vi "CRYGet Error Message.vi"(9 "String In":string, 10 "Error No":i32, 11 "Kind":string) -> (0 "Message Sub 3":string, 1 "Unicode Message Sub":string[](array[string]), 2 "Message Sub":string[](array[string]), 3 "Message":string, 4 "Unicode Message":string, 5 "Window Title":string)   [LabVIEW 2013]
uses:
  CRYMainGlobal.vi
panel:
  # "Get All Error Message."
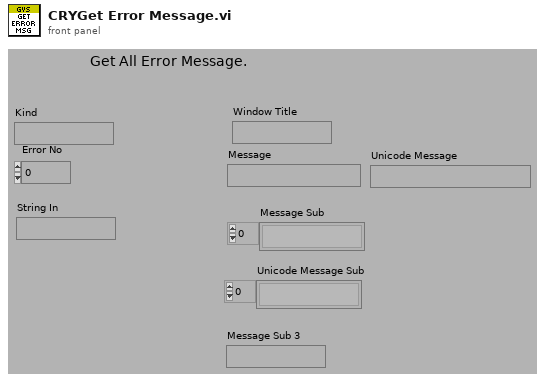
[diagram p1: front panel]
types:
  T1 = enum32{"English", "Chinese", "Korean", "Japanese", "Russian", "Chinese traditional"}
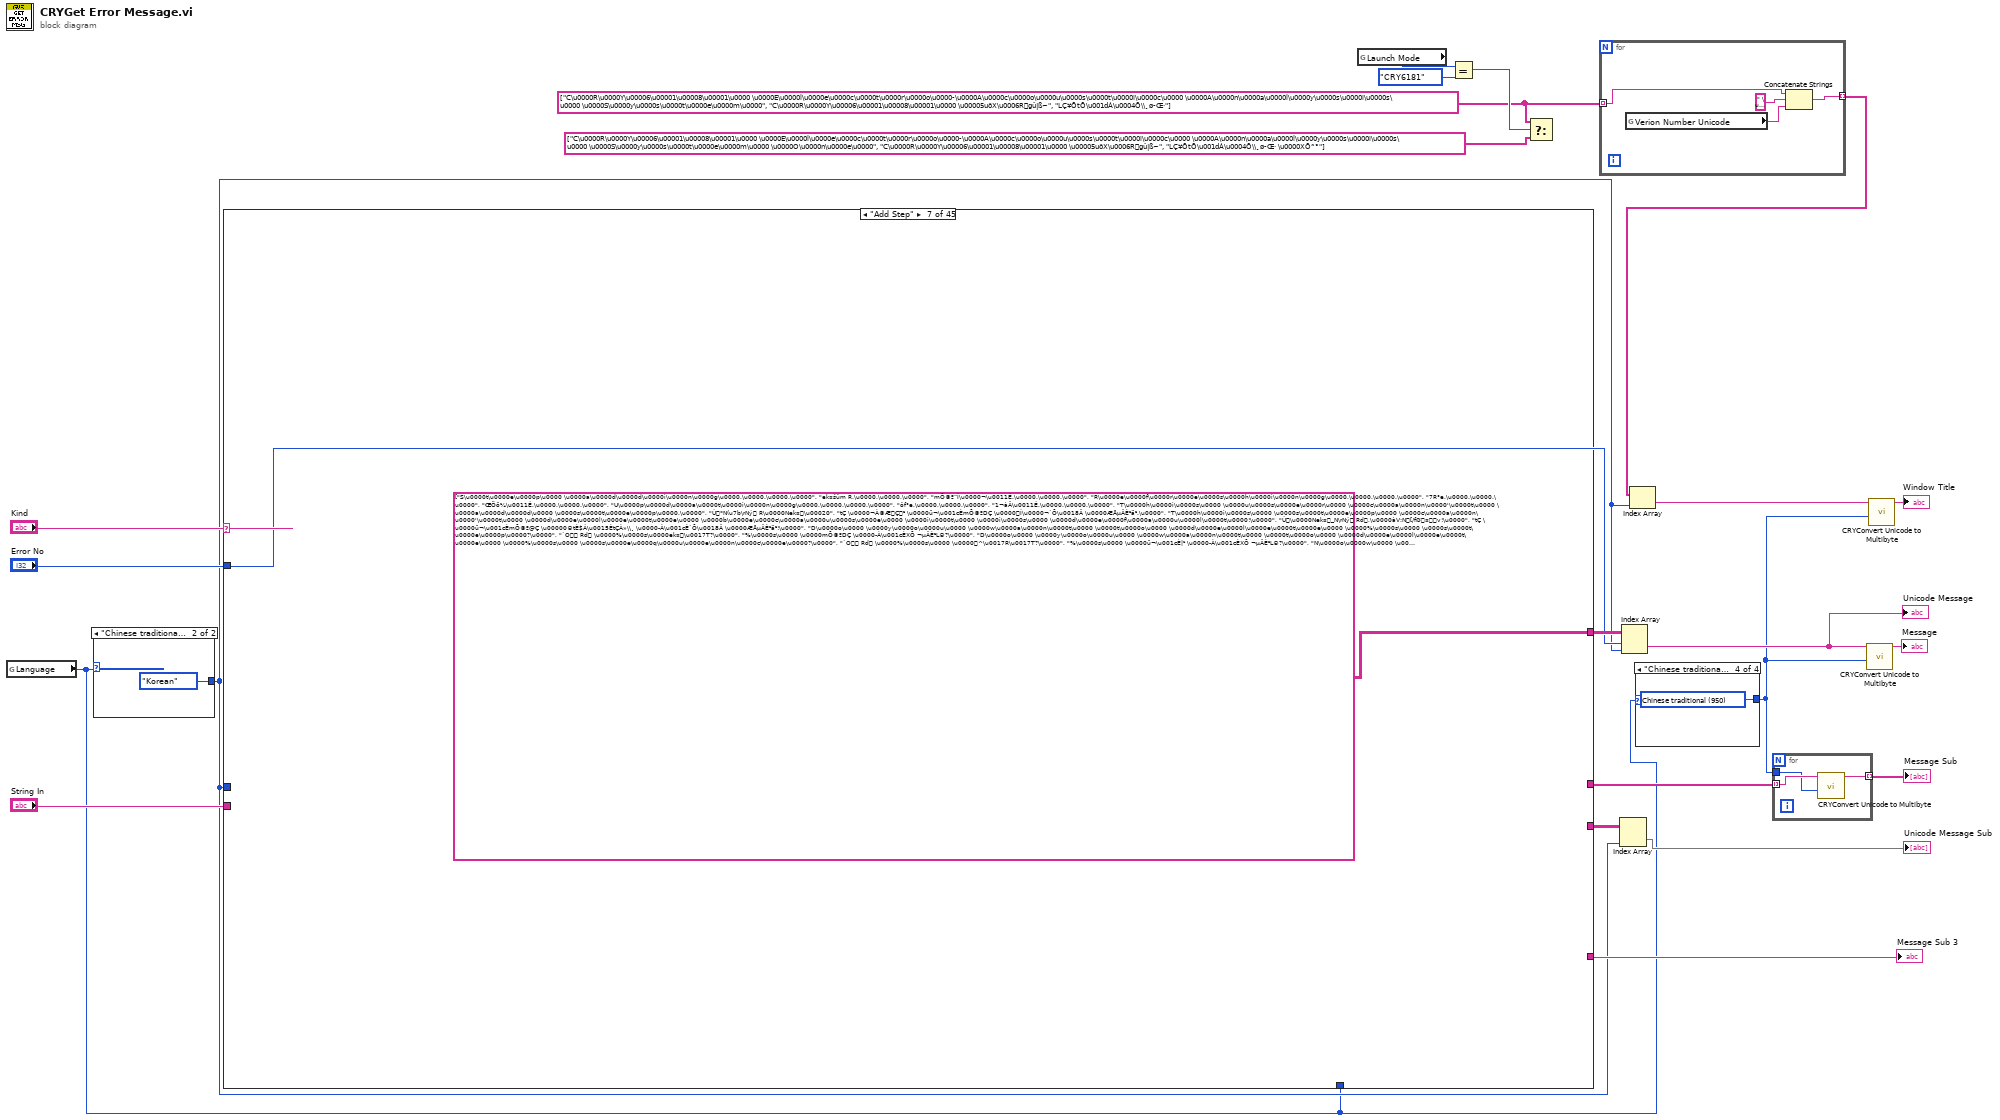
[diagram p0: block diagram]
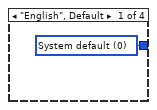
[diagram p3: hidden frame]
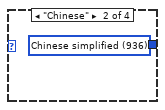
[diagram p4: hidden frame]
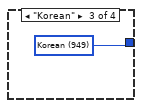
[diagram p5: hidden frame]
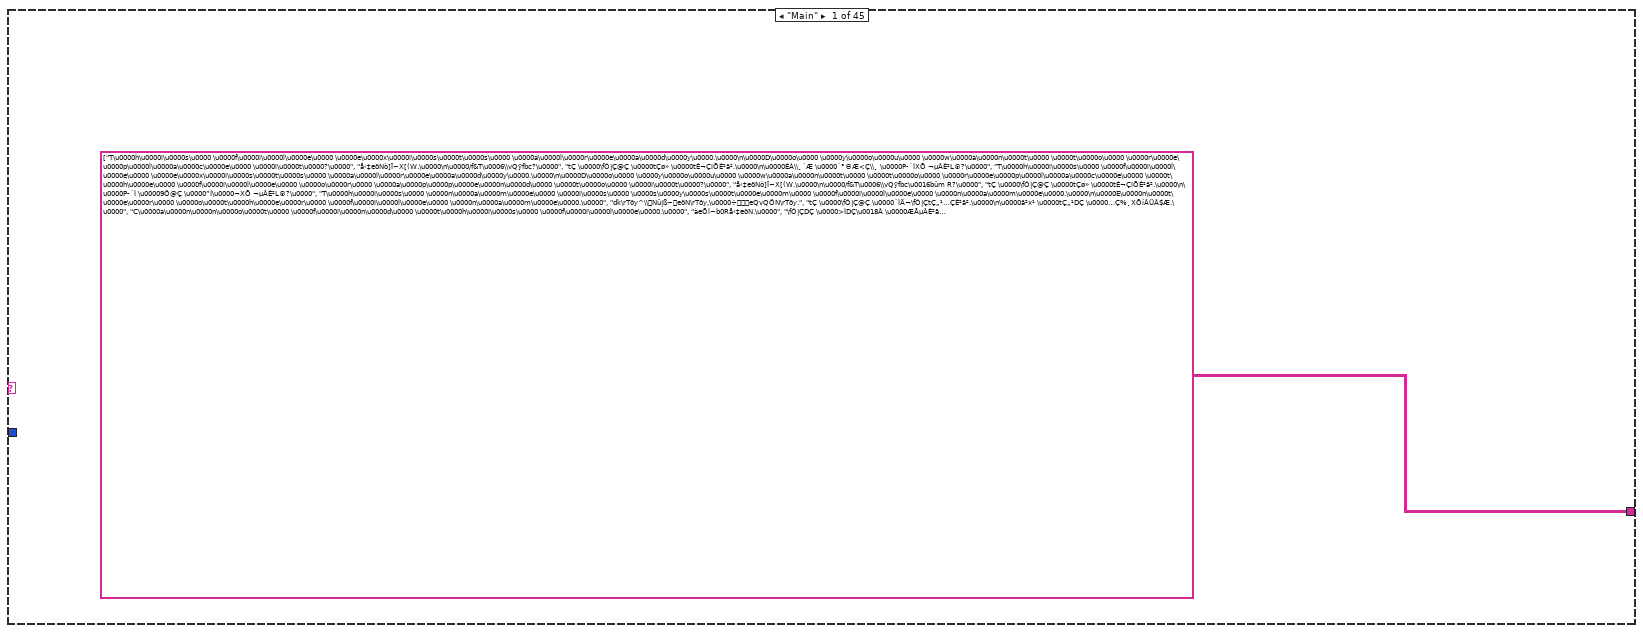
[diagram p6: hidden frame]
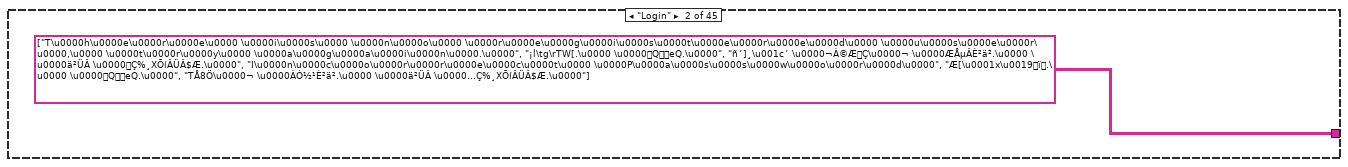
[diagram p7: hidden frame]
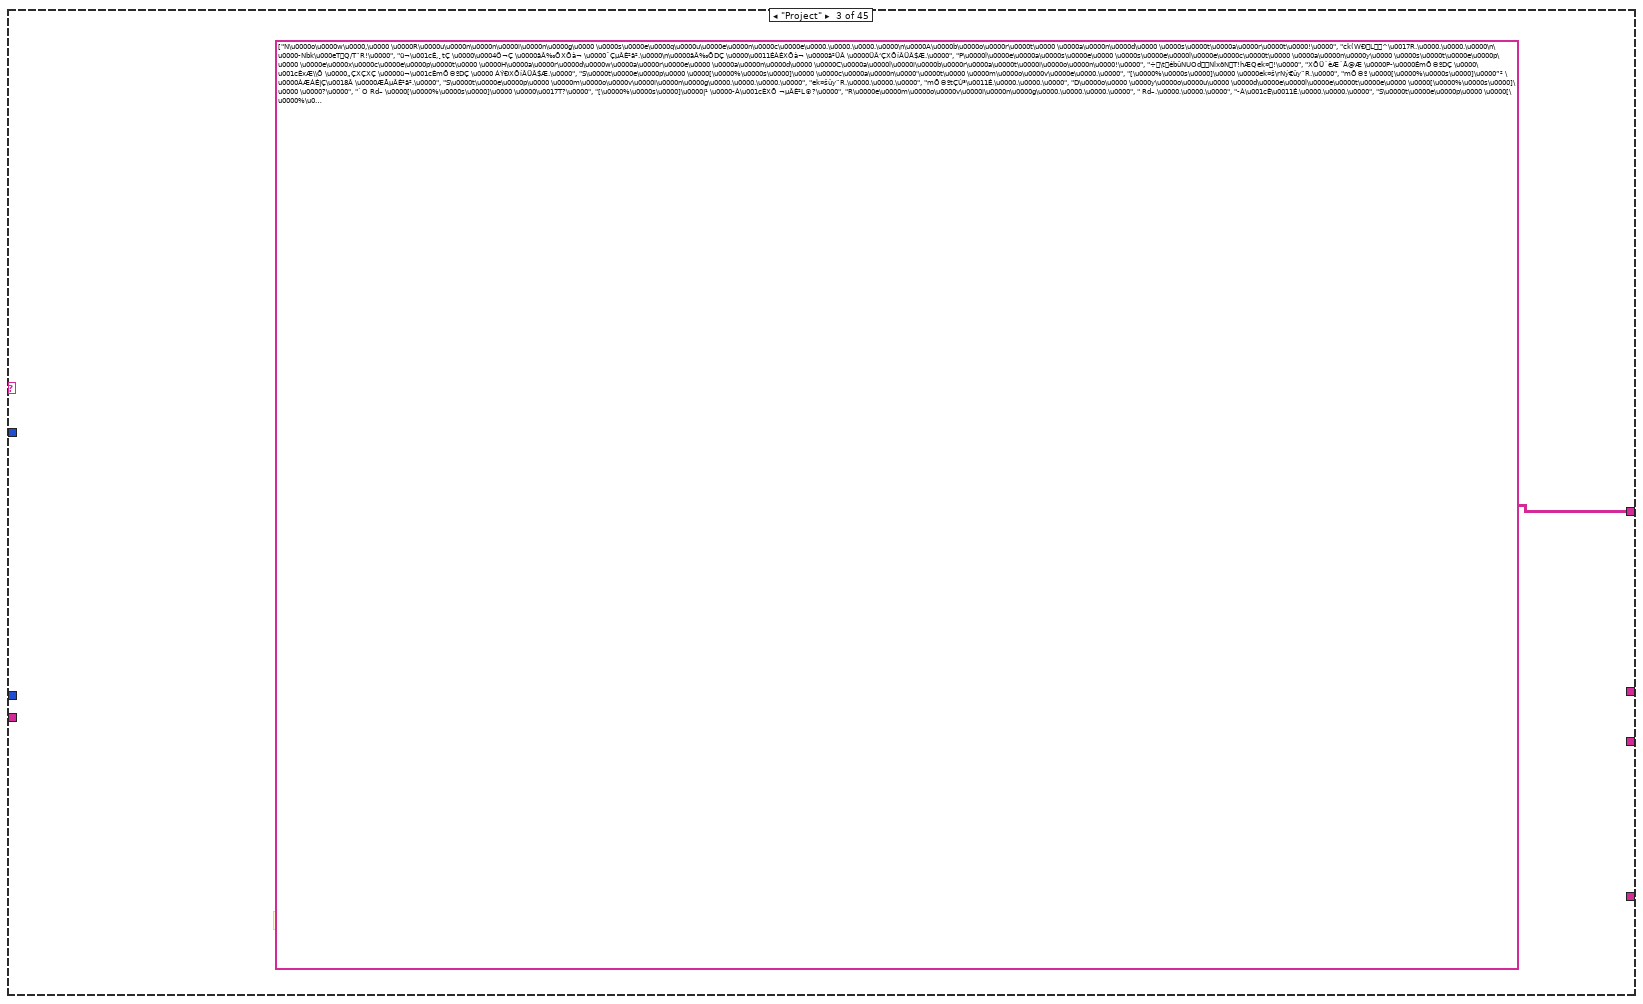
[diagram p8: hidden frame]
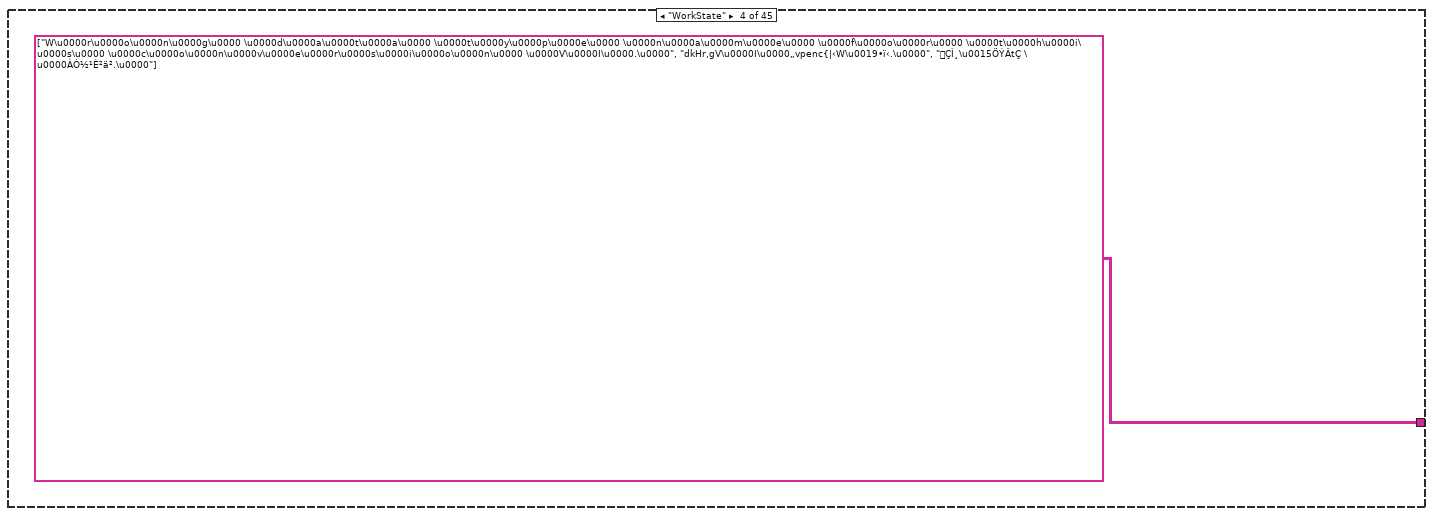
[diagram p9: hidden frame]
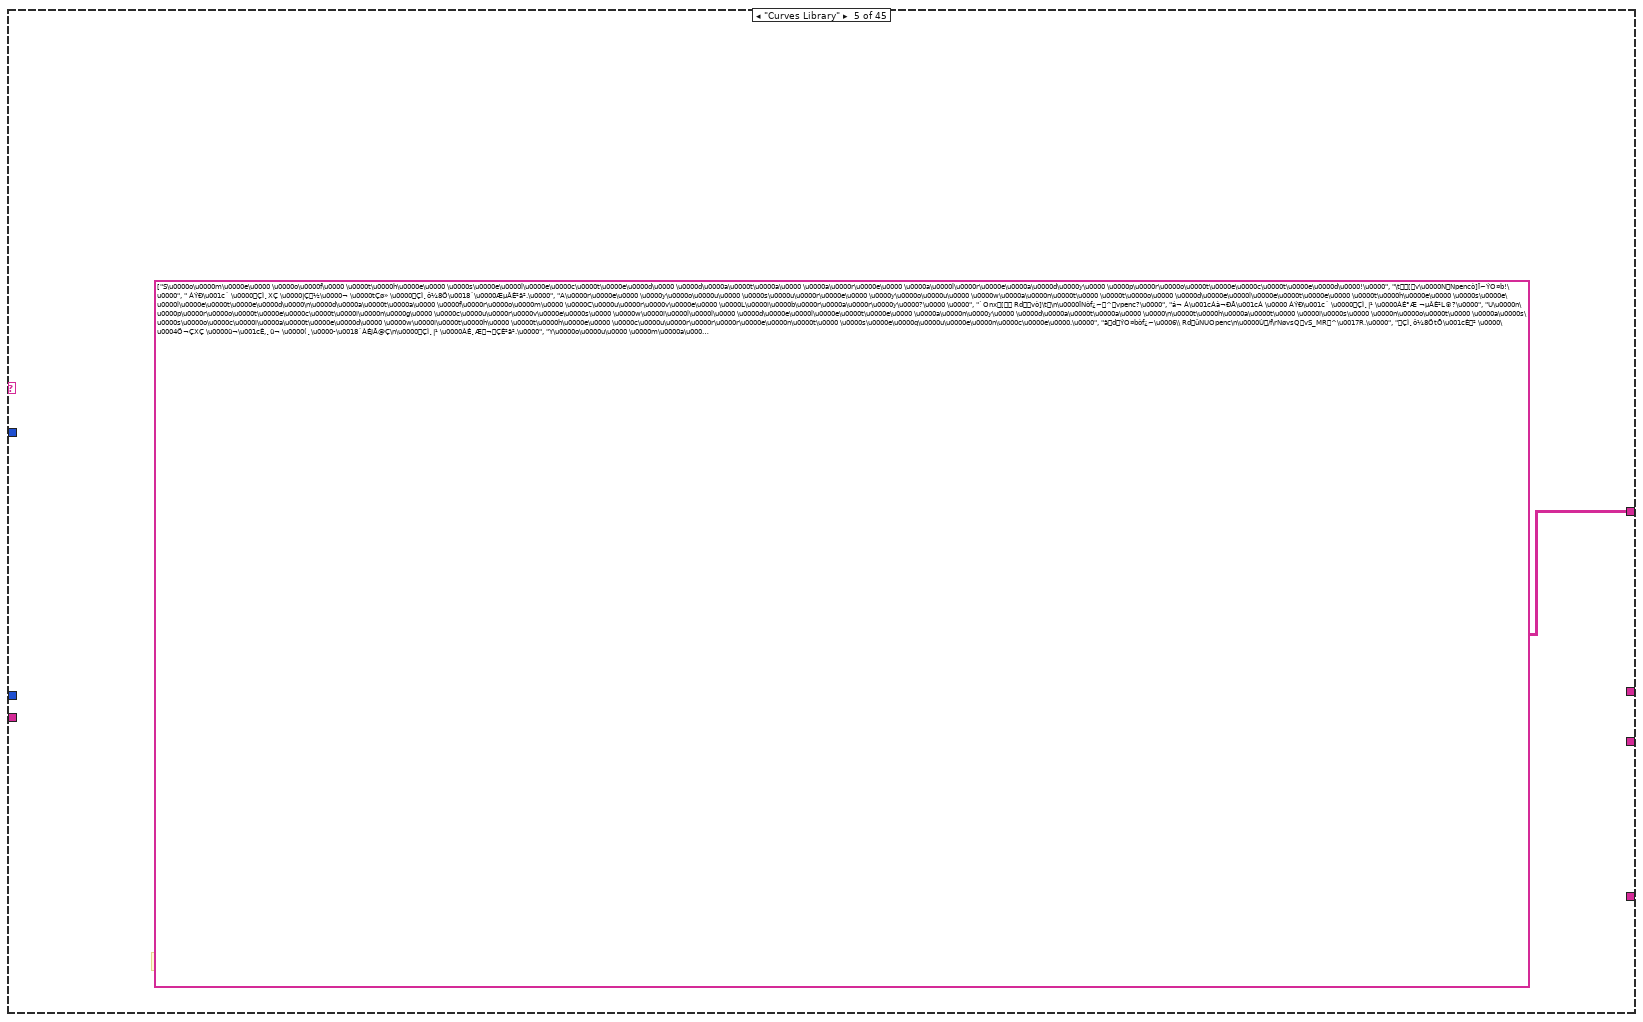
[diagram p10: hidden frame]
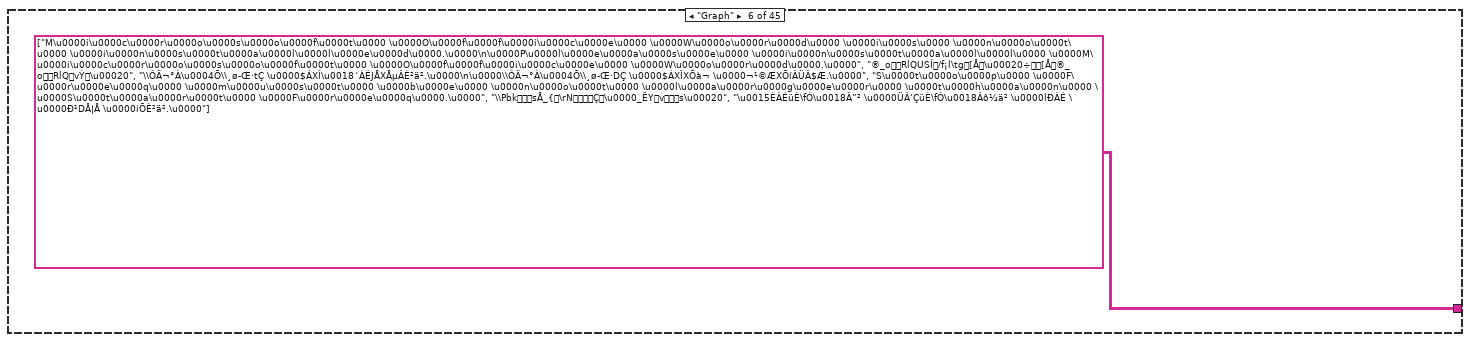
[diagram p11: hidden frame]
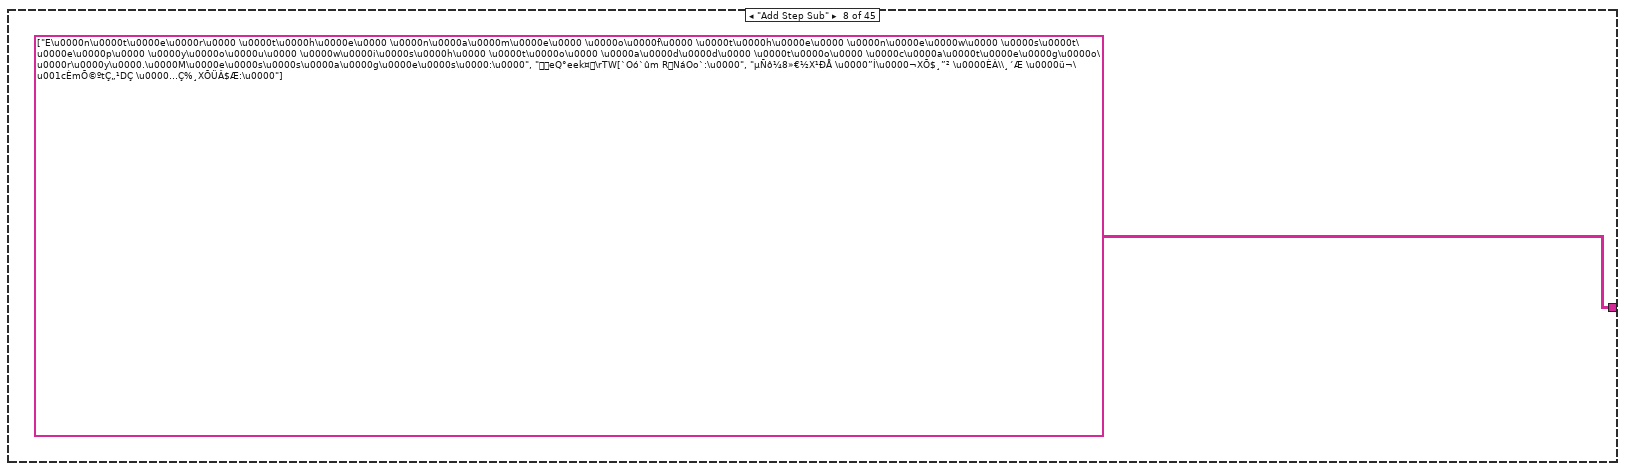
[diagram p12: hidden frame]
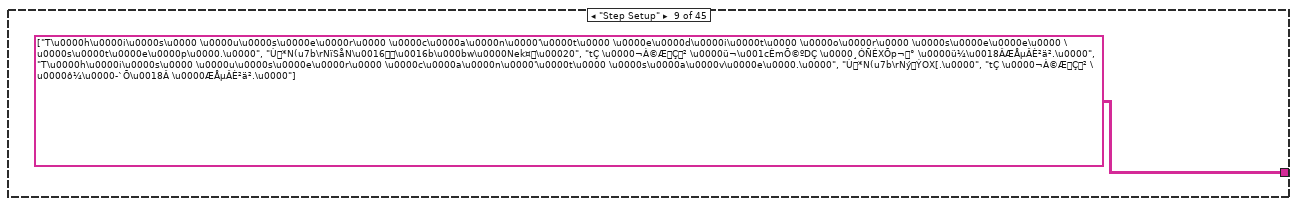
[diagram p13: hidden frame]
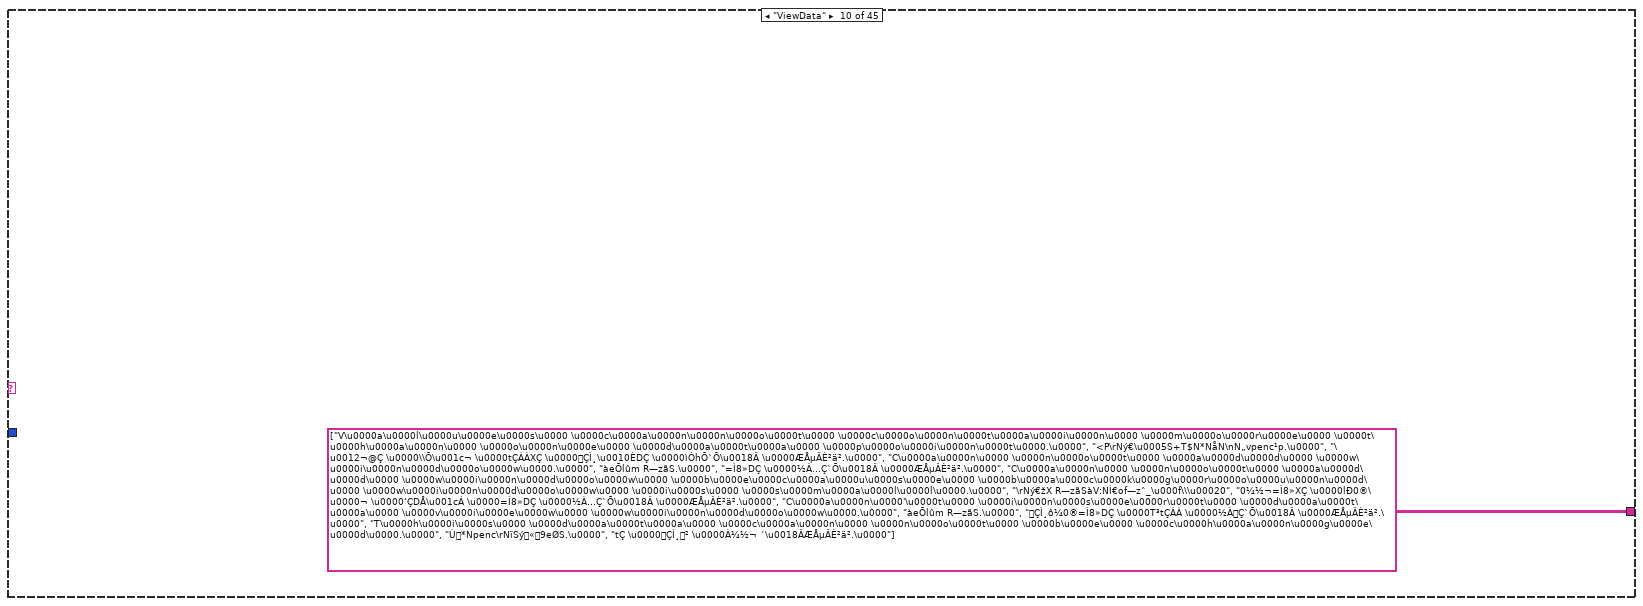
[diagram p14: hidden frame]
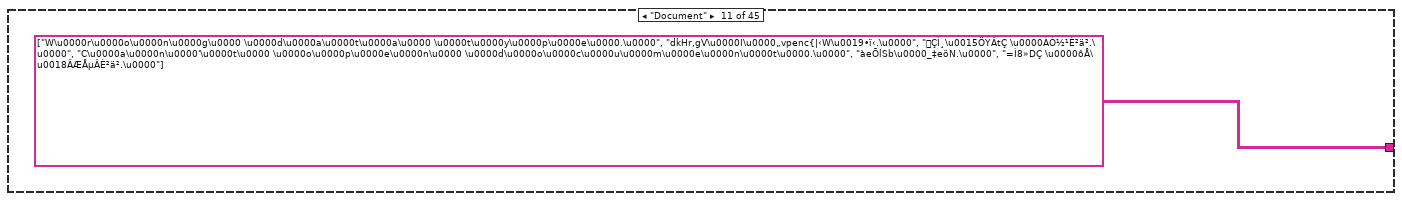
[diagram p15: hidden frame]
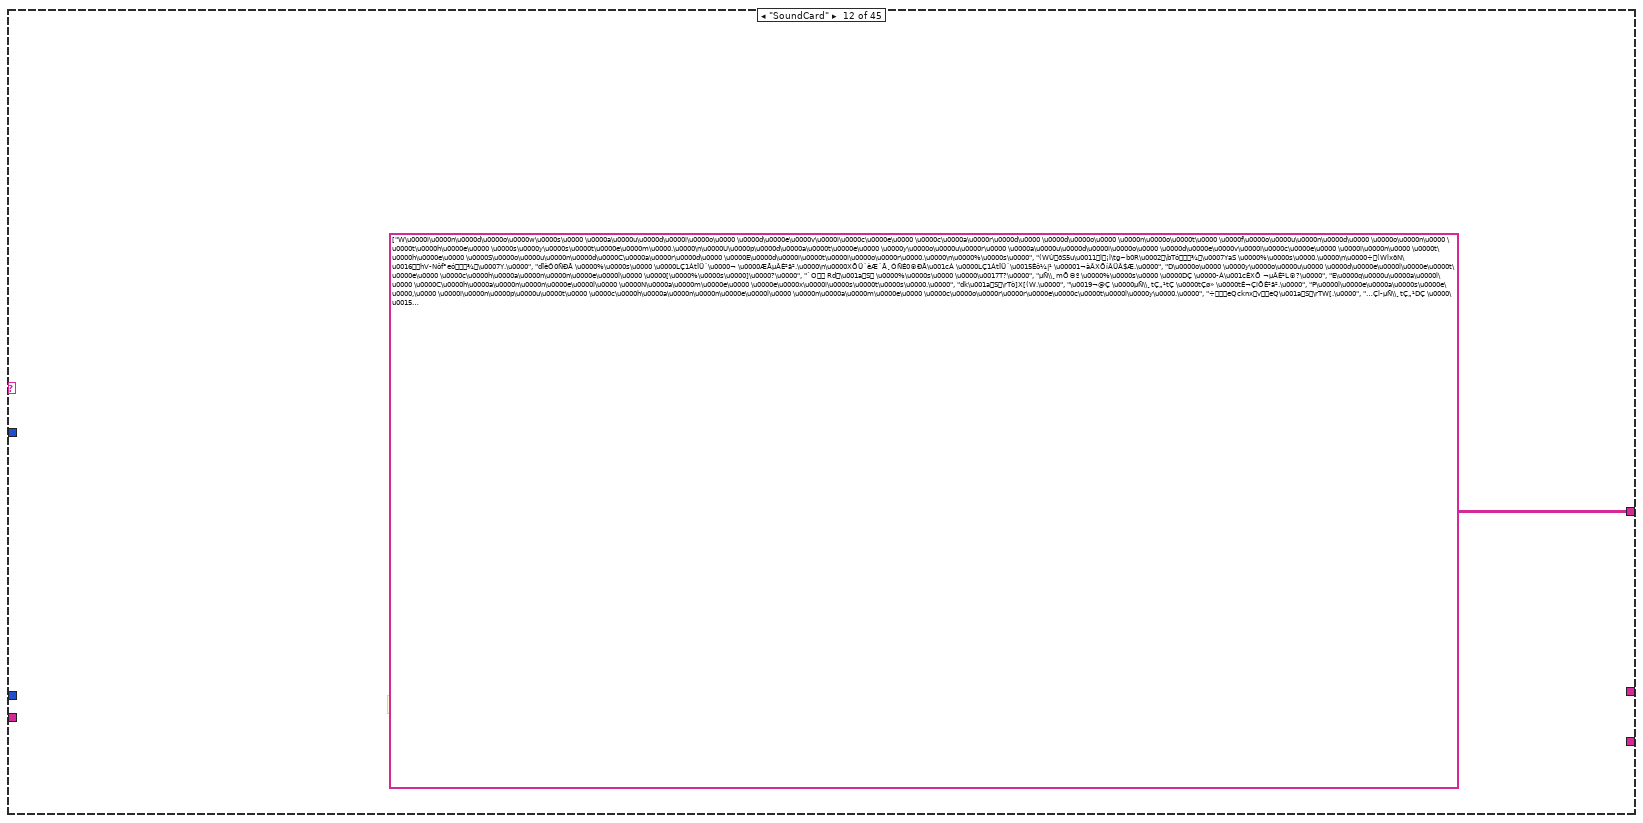
[diagram p16: hidden frame]
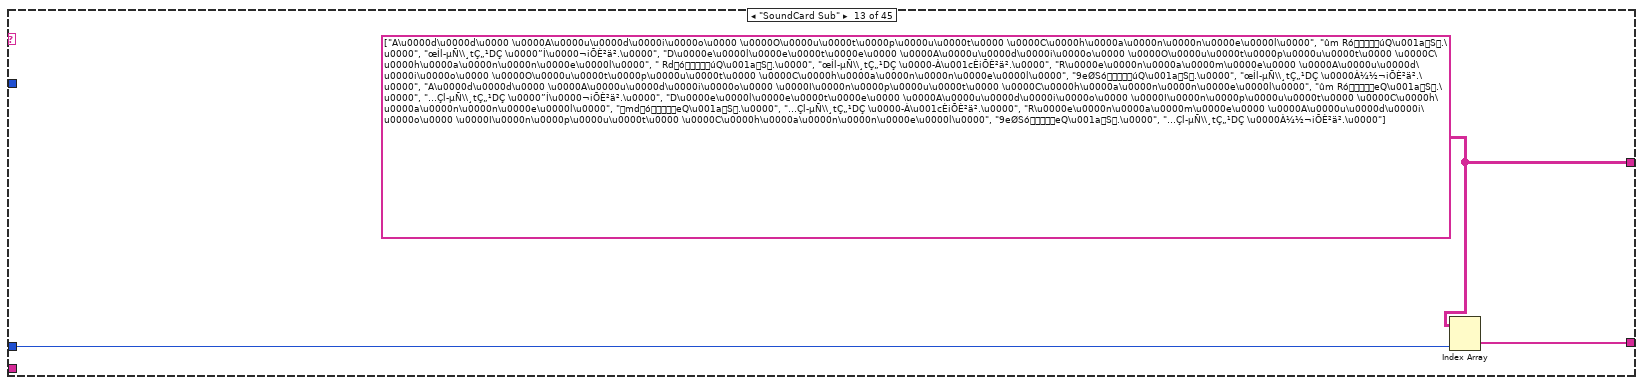
[diagram p17: hidden frame]
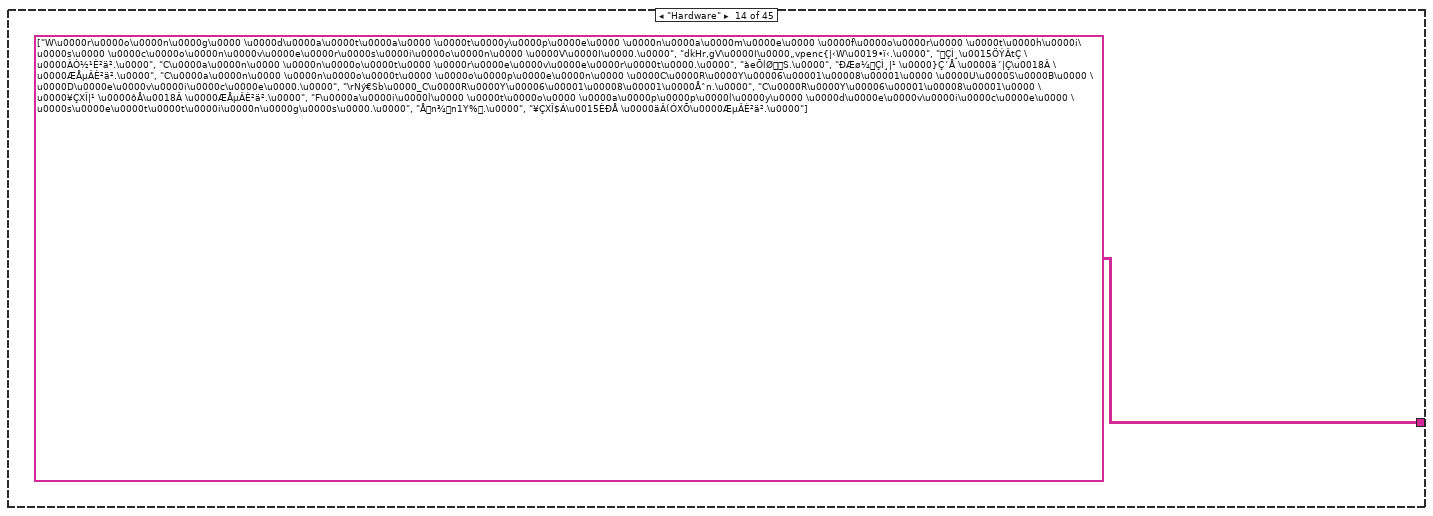
[diagram p18: hidden frame]
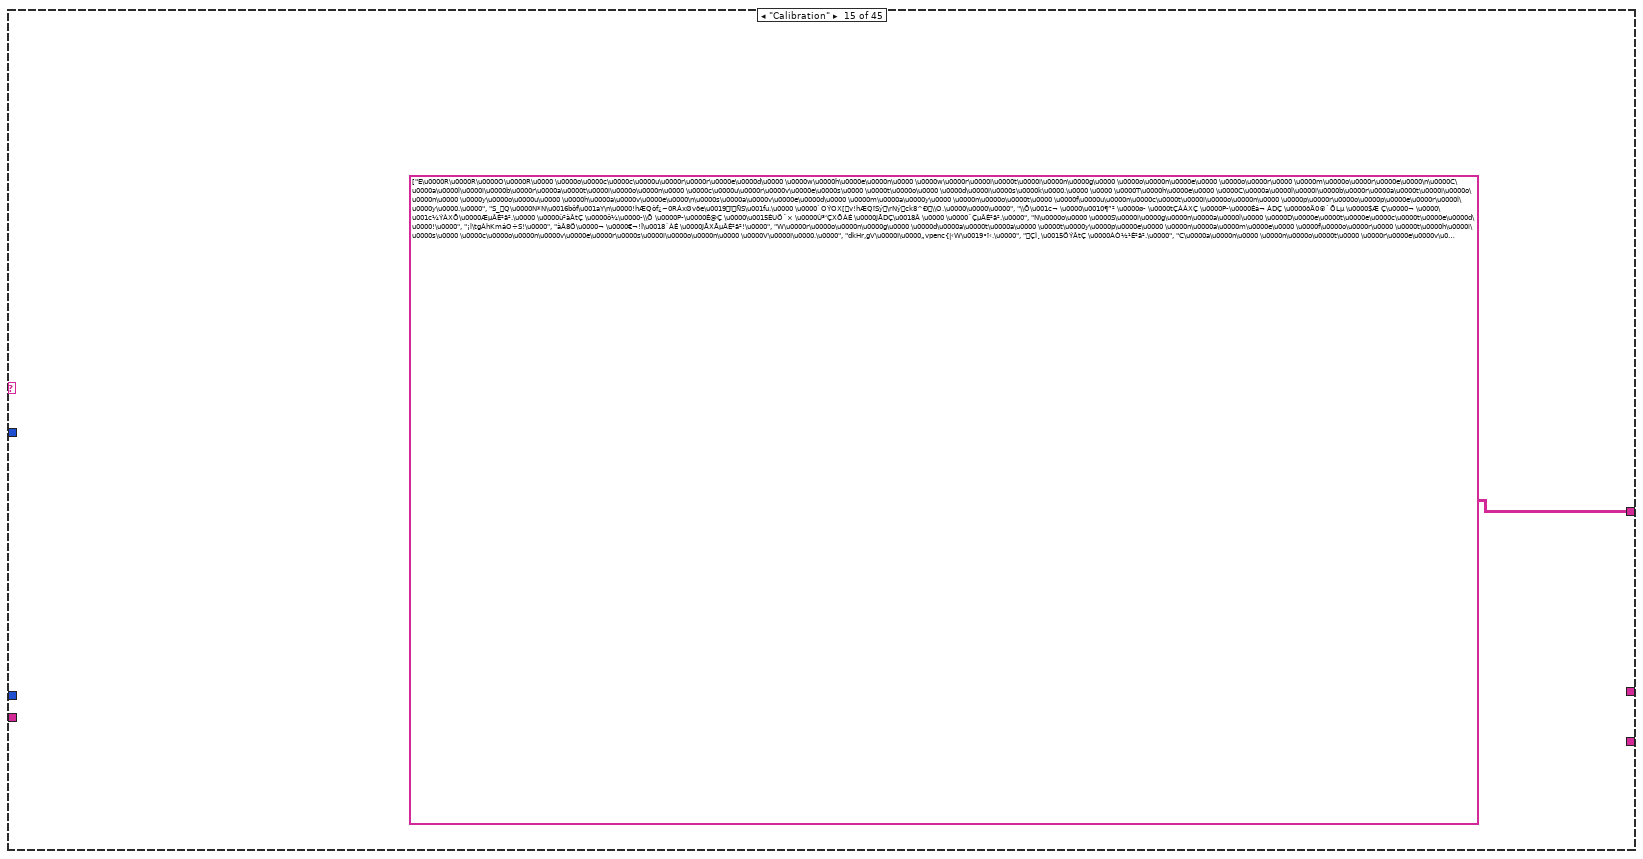
[diagram p19: hidden frame]
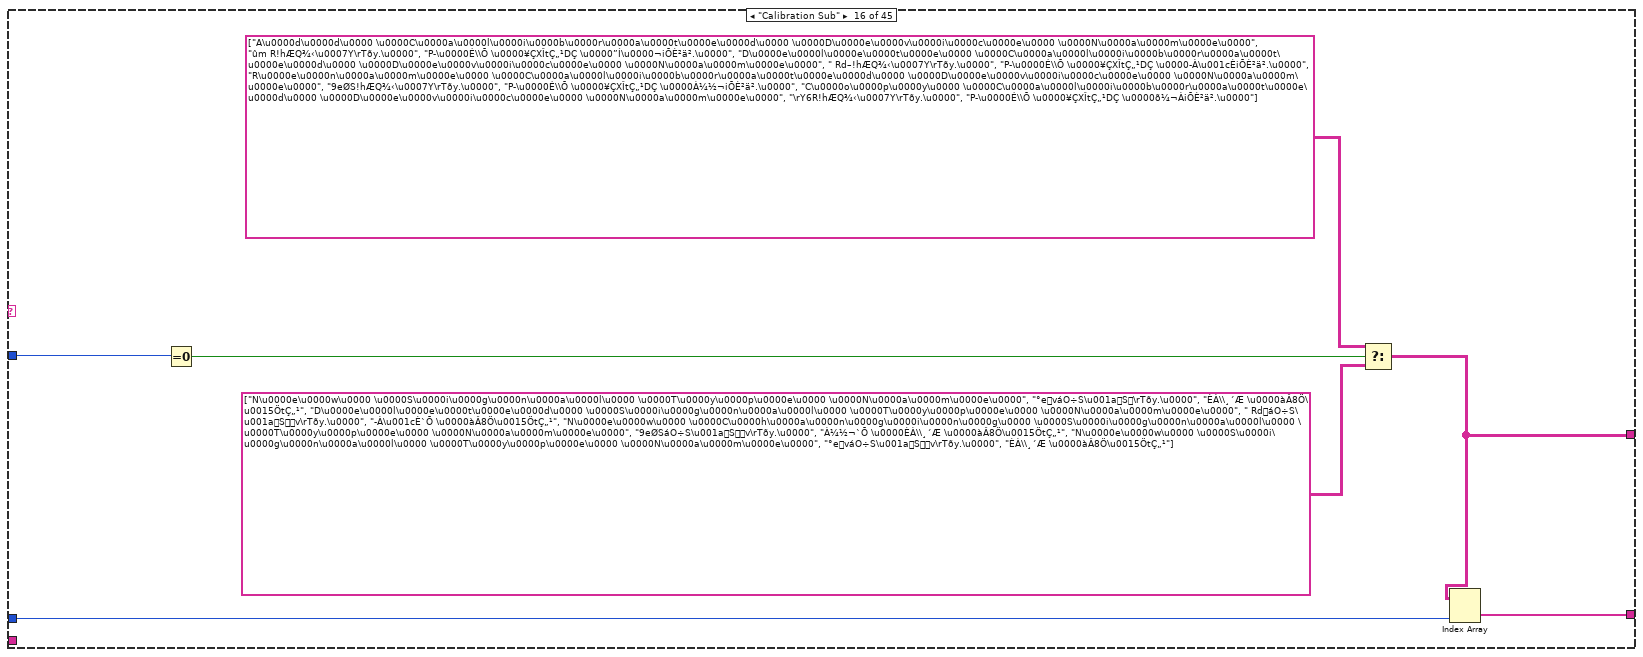
[diagram p20: hidden frame]
diagram:
  w2 = string[] ["C\u0000R\u0000Y\u00006\u00001\u00008\u00001\u0000 \u0000E\u0000l\u0000e\u0000c\u0000t\u0000r\u0000o\u0000-\u0000A\u0000c\u0000o\u0000u\u0000s\u0000t\u0000i\u0000c\u0000 \u0000A\u0000n\u0000a\u0000l\u0000y\u0000s\u0000i\u0000s\u0000 \u0000S\u0000y\u0000s\u0000t\u0000e\u0000m\u0000", "C\u0000R\u0000Y\u00006\u00001\u00008\u00001\u0000 \u00005uðX\u0006Rgû|ß~", "LÇ¥ÕtÕ\u001dÁ\u0004Õ\\¸ø­Œ·"]
  n1 = global read "CRYMainGlobal.vi" "Language"() -> (w7:T1)
  n2 = case shown="\"Chinese traditional\"" w7 {
    selector: w7 -> [w23 _]
    tunnel: [w23 T1."Korean" ("Language")] -> w8
    frame "English", Default {
    }
    frame "Chinese traditional" {
    }
  }
  n3 = case shown="\"Add Step\"" "Kind" {
    tunnel: [string[][] [["T\u0000h\u0000i\u0000s\u0000 \u0000f\u0000i\u0000l\u0000e\u0000 \u0000e\u0000x\u0000i\u0000s\u0000t\u0000s\u0000 \u0000a\u0000l\u0000r\u0000e\u0000a\u0000d\u0000y\u0000.\u0000\n\u0000D\u0000o\u0000 \u0000y\u0000o\u0000u\u0000 \u0000w\u0000a\u0000n\u0000t\u0000 \u0000t\u0000o\u0000 \u0000r\u0000e\u0000p\u0000l\u0000a\u0000c\u0000e\u0000 \u0000i\u0000t\u0000?\u0000", "å‹‡eöNò]Ï~X[(W.\u0000\n\u0000/f&T\u0006\\vQÿfbc?\u0000", "tÇ \u0000\fÓ|Ç@Ç \u0000tÇø» \u0000tÈ¬ÇiÕÈ²ä².\u0000\n\u0000ÈÀ\\¸´Æ \u0000´°©Æ<Ç\\¸ \u0000P­´ÌXÕ ¬µÂÈ²L®?\u0000"], ["T\u0000h\u0000i\u0000s\u0000 \u0000f\u0000i\u0000l\u0000e\u0000 \u0000e\u0000x\u0000i\u0000s\u0000t\u0000s\u0000 \u0000a\u0000l\u0000r\u0000e\u0000a\u0000d\u0000y\u0000.\u0000\n\u0000D\u0000o\u0000 \u0000y\u0000o\u0000u\u0000 \u0000w\u0000a\u0000n\u0000t\u0000 \u0000t\u0000o\u0000 \u0000r\u0000e\u0000p\u0000l\u0000a\u0000c\u0000e\u0000 \u0000t\u0000h\u0000e\u0000 \u0000f\u0000i\u0000l\u0000e\u0000 \u0000o\u0000r\u0000 \u0000a\u0000p\u0000p\u0000e\u0000n\u0000d\u0000 \u0000t\u0000o\u0000 \u0000i\u0000t\u0000?\u0000", "å‹‡eöNò]Ï~X[(W.\u0000\n\u0000/f&T\u0006\\vQÿfbc\u0016bûm R?\u0000", "tÇ \u0000\fÓ|Ç@Ç \u0000tÇø» \u0000tÈ¬ÇiÕÈ²ä².\u0000\n\u0000P­´Ì \u00009Ö@Ç \u0000”Í\u0000¬XÕ ¬µÂÈ²L®?\u0000"], ["T\u0000h\u0000i\u0000s\u0000 \u0000n\u0000a\u0000m\u0000e\u0000 \u0000i\u0000s\u0000 \u0000s\u0000y\u0000s\u0000t\u0000e\u0000m\u0000 \u0000f\u0000i\u0000l\u0000e\u0000 \u0000n\u0000a\u0000m\u0000e\u0000.\u0000\n\u0000E\u0000n\u0000t\u0000e\u0000r\u0000 \u0000o\u0000t\u0000h\u0000e\u0000r\u0000 \u0000f\u0000i\u0000l\u0000e\u0000 \u0000n\u0000a\u0000m\u0000e\u0000.\u0000", "dk\rTðy^\\Nû|ß~eöN\rTðy,\u0000÷eQvQÖN\rTðy.", "tÇ \u0000\fÓ|Ç@Ç \u0000´ÌÄ¬\fÓ|ÇtÇ„¹…ÇÈ²ä².\u0000\n\u0000ä²x¹ \u0000tÇ„¹DÇ \u0000…Ç%¸XÕíÂÜÂ$Æ.\u0000"], ["C\u0000a\u0000n\u0000n\u0000o\u0000t\u0000 \u0000f\u0000i\u0000n\u0000d\u0000 \u0000t\u0000h\u0000i\u0000s\u0000 \u0000f\u0000i\u0000l\u0000e\u0000.\u0000", "àeÕl~b0Rå‹‡eöN.\u0000", "\fÓ|ÇDÇ \u0000>ÌDÇ\u0018Â \u0000ÆÅµÂÈ²ä².\u0000"], ["F\u0000i\u0000l\u0000e\u0000 \u0000e\u0000x\u0000t\u0000e\u0000n\u0000s\u0000i\u0000o\u0000n\u0000 \u0000i\u0000s\u0000 \u0000n\u0000o\u0000t\u0000 \u0000e\u0000q\u0000u\u0000a\u0000l\u0000.\u0000 \u0000(\u0000%\u0000s\u0000)\u0000", "‡eöNibU\\\rT\rN\fT.\u0000(\u0000%\u0000s\u0000)\u0000", "\fÓ|ÇUÖ¥ÇÇ\u0000¬ \u0000\u0019¬ÀÉ \u0000JÅµÂÈ²ä².\u0000(\u0000%\u0000s\u0000)\u0000"], ["W\u0000r\u0000o\u0000n\u0000g\u0000 \u0000d\u0000a\u0000t\u0000a\u0000 \u0000t\u0000y\u0000p\u0000e\u0000 \u0000n\u0000a\u0000m\u0000e\u0000 \u0000f\u0000o\u0000r\u0000 \u0000t\u0000h\u0000i\u0000s\u0000 \u0000v\u0000e\u0000r\u0000s\u0000i\u0000o\u0000n\u0000 \u0000V\u0000I\u0000", "dkHr,gV\u0000I\u0000„vpenc{|‹W\u0019•ï‹.\u0000", "ÇÌ¸À¼XÖÜÂ \u0000ÇÌ¸\u0015ÖtÇ \u0000ÀÒ½¹È²ä².\u0000"], ["D\u0000o\u0000 \u0000y\u0000o\u0000u\u0000 \u0000w\u0000a\u0000n\u0000t\u0000 \u0000t\u0000o\u0000 \u0000s\u0000a\u0000v\u0000e\u0000 \u0000c\u0000h\u0000a\u0000n\u0000g\u0000e\u0000s\u0000 \u0000?\u0000", "/f&TÝOX[ò]ôf9e„v…Q¹[?\u0000", "ô¼\u0000­XÕ ¬µÂÈ²L®?\u0000"], ["E\u0000r\u0000r\u0000o\u0000r\u0000 \u0000o\u0000c\u0000c\u0000u\u0000r\u0000e\u0000d\u0000 \u0000i\u0000n\u0000 \u0000e\u0000x\u0000e\u0000c\u0000u\u0000t\u0000i\u0000n\u0000g\u0000 \u0000t\u0000h\u0000e\u0000 \u0000A\u0000d\u0000o\u0000b\u0000e\u0000 \u0000R\u0000e\u0000a\u0000d\u0000e\u0000r\u0000.\u0000e\u0000x\u0000e\u0000!\u0000\n\u0000P\u0000l\u0000e\u0000a\u0000s\u0000e\u0000 \u0000s\u0000e\u0000t\u0000u\u0000p\u0000 \u0000t\u0000h\u0000e\u0000 \u0000A\u0000d\u0000o\u0000b\u0000e\u0000 \u0000R\u0000e\u0000a\u0000d\u0000e\u0000r\u0000 \u0000P\u0000r\u0000o\u0000g\u0000r\u0000a\u0000m\u0000.\u0000", "÷‹‰[ÅˆA\u0000d\u0000o\u0000b\u0000e\u0000 \u0000R\u0000e\u0000a\u0000d\u0000e\u0000r\u0000.\u0000", "¬À©Æ$Á…º\u001cÁ|¹ \u0000ô¼0® \u0000\u0004ÇXÕìÅ \u0000P\u0000D\u0000F\u0000ôÅŒ·0® \u0000A\u0000c\u0000r\u0000o\u0000b\u0000a\u0000t\u0000|¹ \u0000$ÁXÎXÕíÂÜÂ$Æ.\u0000"], ["E\u0000r\u0000r\u0000o\u0000r\u0000 \u0000O\u0000c\u0000c\u0000u\u0000r\u0000e\u0000d\u0000 \u0000I\u0000n\u0000 \u0000d\u0000i\u0000s\u0000p\u0000l\u0000a\u0000y\u0000i\u0000n\u0000g\u0000 \u0000t\u0000h\u0000e\u0000 \u0000U\u0000s\u0000e\u0000r\u0000 \u0000M\u0000a\u0000n\u0000u\u0000a\u0000l\u0000!\u0000\n\u0000C\u0000R\u0000Y\u0000M\u0000a\u0000n\u0000u\u0000a\u0000l\u0000 \u0000f\u0000i\u0000l\u0000e\u0000 \u0000h\u0000a\u0000s\u0000 \u0000b\u0000e\u0000e\u0000n\u0000 \u0000m\u0000o\u0000v\u0000e\u0000d\u0000 \u0000o\u0000r\u0000 \u0000d\u0000e\u0000l\u0000e\u0000t\u0000e\u0000d\u0000.\u0000", "KbŒQ‡eöNò]«ˆûy¨R\u0016b Rd–.\u0000", "¬À©Æ$Á…º\u001cÁ\u0000¬ \u0000ÆÅµÂÈ²ä².\u0000 \u0000UÖxÇXÕíÂÜÂ$Æ.\u0000"], ["Y\u0000o\u0000u\u0000 \u0000a\u0000r\u0000e\u0000 \u0000s\u0000w\u0000i\u0000t\u0000c\u0000h\u0000i\u0000n\u0000g\u0000 \u0000b\u0000e\u0000t\u0000w\u0000e\u0000e\u0000n\u0000 \u0000C\u0000R\u0000Y\u00006\u00001\u00008\u00001\u0000 \u0000O\u0000n\u0000e\u0000 \u0000a\u0000n\u0000d\u0000 \u0000r\u0000e\u0000g\u0000u\u0000l\u0000a\u0000r\u0000 \u0000C\u0000R\u0000Y\u00006\u00001\u00008\u00001\u0000,\u0000 \u0000\n\u0000C\u0000R\u0000Y\u00006\u00001\u00008\u00001\u0000 \u0000m\u0000u\u0000s\u0000t\u0000 \u0000b\u0000e\u0000 \u0000r\u0000e\u0000s\u0000t\u0000a\u0000r\u0000t\u0000e\u0000d\u0000 \u0000a\u0000n\u0000d\u0000 \u0000i\u0000s\u0000 \u0000e\u0000x\u0000i\u0000t\u0000i\u0000n\u0000g\u0000 \u0000n\u0000o\u0000w\u0000.\u0000", "ck(WC\u0000R\u0000Y\u00006\u00001\u00008\u00001\u0000 \u0000O\u0000n\u0000e\u0000T\u0007hÆQC\u0000R\u0000Y\u00006\u00001\u00008\u00001\u0000KNô\u0007Rbc.\u0000\n\u0000C\u0000R\u0000Y\u00006\u00001\u00008\u00001\u0000Å_{Í°e/T¨R,\u0000ck(W\u0000úQ\u00020", "ù²àÂ@Ç \u0000ÀÉ\b® \u0000LÇ¥ÕtÕ\u001dÁ\u0004Õ\\¸ø­Œ·ü¬ \u0000LÇ¥ÕtÕ\u001dÁ\u0004Õ\\¸ø­Œ· \u0000XÕ˜°¬ÀtÇÐÅ \u0000\bÈXÖXÕ$¸à¬ \u0000XÕà¬ˆÇµÂÈ²ä².\u0000 \u0000 \u0000\n\u0000LÇ¥ÕtÕ\u001dÁ\u0004Õ\\¸ø­Œ·DÇ \u0000¬Ç0®Ù³XÕ|Å|Å \u0000XÕpº \u0000ç¬ \u0000\u0004Õ\\¸ø­Œ·@Ç \u0000DÆÌ¸)´È²ä².\u0000"], ["L\u0000a\u0000n\u0000g\u0000u\u0000a\u0000g\u0000e\u0000 \u0000s\u0000e\u0000t\u0000t\u0000i\u0000n\u0000g\u0000 \u0000i\u0000s\u0000 \u0000c\u0000h\u0000a\u0000n\u0000g\u0000e\u0000d\u0000.\u0000\n\u0000C\u0000R\u0000Y\u00006\u00001\u00008\u00001\u0000 \u0000m\u0000u\u0000s\u0000t\u0000 \u0000b\u0000e\u0000 \u0000r\u0000e\u0000s\u0000t\u0000a\u0000r\u0000t\u0000e\u0000d\u0000 \u0000a\u0000n\u0000d\u0000 \u0000i\u0000s\u0000 \u0000e\u0000x\u0000i\u0000t\u0000i\u0000n\u0000g\u0000 \u0000n\u0000o\u0000w\u0000.\u0000", "í\u0000¾n«9eØS\u00020\n\u0000C\u0000R\u0000Y\u00006\u00001\u00008\u00001\u0000Å_{Í°e/T¨Rck(W\u0000úQ\u00020", "¸Å´Å$Á\u0015ÈtÇ \u0000À¼½¬\u0018´\u0000ÆµÂÈ²ä².\u0000\n\u0000C\u0000R\u0000Y\u00006\u00001\u00008\u00001\u0000”² \u0000¬Ç0®Ù³XÕìÅ|Å \u0000iÕÈ²ä².\u0000"], ["N\u0000o\u0000 \u0000H\u0000a\u0000r\u0000d\u0000w\u0000a\u0000r\u0000e\u0000 \u0000K\u0000e\u0000y\u0000!\u0000", "¡l\tglxöNÆ[¥”!\u0000", "XÕÜ´èÆ´Å¤Ð\u0000¬ \u0000ÆÅµÂÈ²ä²!\u0000"]] ("Array") string[][] [["T\u0000h\u0000e\u0000r\u0000e\u0000 \u0000i\u0000s\u0000 \u0000n\u0000o\u0000 \u0000r\u0000e\u0000g\u0000i\u0000s\u0000t\u0000e\u0000r\u0000e\u0000d\u0000 \u0000u\u0000s\u0000e\u0000r\u0000,\u0000 \u0000t\u0000r\u0000y\u0000 \u0000a\u0000g\u0000a\u0000i\u0000n\u0000.\u0000", "¡l\tg\rTW[.\u0000 \u0000QeQ.\u0000", "ñ´]¸\u001c´ \u0000¬À©ÆÇ\u0000¬ \u0000ÆÅµÂÈ²ä².\u0000 \u0000ä²ÜÂ \u0000Ç%¸XÕíÂÜÂ$Æ.\u0000"], ["I\u0000n\u0000c\u0000o\u0000r\u0000r\u0000e\u0000c\u0000t\u0000 \u0000P\u0000a\u0000s\u0000s\u0000w\u0000o\u0000r\u0000d\u0000", "Æ[\u0001x\u0019ï.\u0000 \u0000QeQ.\u0000", "TÅ8Ö\u0000¬ \u0000ÀÒ½¹È²ä².\u0000 \u0000ä²ÜÂ \u0000…Ç%¸XÕíÂÜÂ$Æ.\u0000"]] string[][] [["N\u0000o\u0000w\u0000,\u0000 \u0000R\u0000u\u0000n\u0000n\u0000i\u0000n\u0000g\u0000 \u0000s\u0000e\u0000q\u0000u\u0000e\u0000n\u0000c\u0000e\u0000.\u0000.\u0000.\u0000\n\u0000A\u0000b\u0000o\u0000r\u0000t\u0000 \u0000a\u0000n\u0000d\u0000 \u0000s\u0000t\u0000a\u0000r\u0000t\u0000!\u0000", "ck(WÐL^\u0017R.\u0000.\u0000.\u0000\n\u0000-Nbk\u000eTQ/T¨R!\u0000", "ü¬\u001cÈ,¸tÇ \u0000\u0004Ö¬Ç \u0000äÂ‰ÕXÕà¬ \u0000ˆÇµÂÈ²ä².\u0000\n\u0000äÂ‰ÕDÇ \u0000\u0011ÉÀÉXÕà¬ \u0000ä²ÜÂ \u0000ÜÂ‘ÇXÕíÂÜÂ$Æ.\u0000"], ["P\u0000l\u0000e\u0000a\u0000s\u0000e\u0000 \u0000s\u0000e\u0000l\u0000e\u0000c\u0000t\u0000 \u0000a\u0000n\u0000y\u0000 \u0000s\u0000t\u0000e\u0000p\u0000 \u0000e\u0000x\u0000c\u0000e\u0000p\u0000t\u0000 \u0000H\u0000a\u0000r\u0000d\u0000w\u0000a\u0000r\u0000e\u0000 \u0000a\u0000n\u0000d\u0000 \u0000C\u0000a\u0000l\u0000i\u0000b\u0000r\u0000a\u0000t\u0000i\u0000o\u0000n\u0000!\u0000", "÷\tébûNUOdNlxöNT!hÆQek¤!\u0000", "XÕÜ´èÆ´Å@Æ \u0000P­\u0000ÉmÕ©ºDÇ \u0000\u001cÈxÆ\\Õ \u0000„ÇXÇXÇ \u0000ü¬\u001cÈmÕ©ºDÇ \u0000 ÁÝÐXÕíÂÜÂ$Æ.\u0000"], ["S\u0000t\u0000e\u0000p\u0000 \u0000[\u0000%\u0000s\u0000]\u0000 \u0000c\u0000a\u0000n\u0000'\u0000t\u0000 \u0000m\u0000o\u0000v\u0000e\u0000.\u0000", "[\u0000%\u0000s\u0000]\u0000 \u0000ek¤š\rNý€ûy¨R.\u0000", "mÕ©º \u0000[\u0000%\u0000s\u0000]\u0000”² \u0000ÀÆÁÉ|Ç\u0018Â \u0000ÆÅµÂÈ²ä².\u0000"], ["S\u0000t\u0000e\u0000p\u0000 \u0000m\u0000o\u0000v\u0000i\u0000n\u0000g\u0000.\u0000.\u0000.\u0000", "ek¤šûy¨R.\u0000.\u0000.\u0000", "mÕ©ºtÇÙ³\u0011É.\u0000.\u0000.\u0000"], ["D\u0000o\u0000 \u0000y\u0000o\u0000u\u0000 \u0000d\u0000e\u0000l\u0000e\u0000t\u0000e\u0000 \u0000[\u0000%\u0000s\u0000]\u0000 \u0000?\u0000", "`O Rd– \u0000[\u0000%\u0000s\u0000]\u0000 \u0000\u0017T?\u0000", "[\u0000%\u0000s\u0000]\u0000|¹ \u0000­À\u001cÈXÕ ¬µÂÈ²L®?\u0000"], ["R\u0000e\u0000m\u0000o\u0000v\u0000i\u0000n\u0000g\u0000.\u0000.\u0000.\u0000", " Rd–.\u0000.\u0000.\u0000", "­À\u001cÈ\u0011É.\u0000.\u0000.\u0000"], ["S\u0000t\u0000e\u0000p\u0000 \u0000[\u0000%\u0000s\u0000]\u0000 \u0000c\u0000a\u0000n\u0000'\u0000t\u0000 \u0000d\u0000e\u0000l\u0000e\u0000t\u0000e\u0000.\u0000", "[\u0000%\u0000s\u0000]\u0000 \u0000ek¤š\rNý€ Rd–.\u0000", "mÕ©º \u0000[\u0000%\u0000s\u0000]\u0000”² \u0000­À\u001cÈ`Õ\u0018Â \u0000ÆÅµÂÈ²ä².\u0000"], ["S\u0000t\u0000e\u0000p\u0000 \u0000l\u0000o\u0000a\u0000d\u0000i\u0000n\u0000g\u0000.\u0000.\u0000.\u0000", "ek¤}eQ-N.\u0000.\u0000.\u0000", "mÕ©º \u0000}Ç”²\u0011É.\u0000.\u0000.\u0000"], ["T\u0000S\u0000 \u0000n\u0000a\u0000m\u0000e\u0000 \u0000c\u0000h\u0000a\u0000n\u0000g\u0000i\u0000n\u0000g\u0000.\u0000.\u0000.\u0000", "y˜îvÈp\rTðyôf9e.\u0000.\u0000.\u0000", "ü¬\u001cÈ,¸tÇ„¹À¼½¬\u0011É.\u0000.\u0000"], ["S\u0000t\u0000e\u0000p\u0000 \u0000a\u0000d\u0000d\u0000i\u0000n\u0000g\u0000.\u0000.\u0000.\u0000", "ek¤šûm R.\u0000.\u0000.\u0000", "mÕ©º”Í\u0000¬\u0011É.\u0000.\u0000"], ["H\u0000a\u0000r\u0000d\u0000w\u0000a\u0000r\u0000e\u0000 \u0000o\u0000r\u0000 \u0000C\u0000a\u0000l\u0000i\u0000b\u0000r\u0000a\u0000t\u0000i\u0000o\u0000n\u0000 \u0000c\u0000a\u0000n\u0000 \u0000i\u0000n\u0000s\u0000e\u0000r\u0000t\u0000 \u0000o\u0000n\u0000l\u0000y\u0000 \u0000i\u0000n\u0000 \u0000f\u0000i\u0000r\u0000s\u0000t\u0000 \u0000a\u0000n\u0000d\u0000 \u0000s\u0000e\u0000c\u0000o\u0000n\u0000d\u0000 \u0000L\u0000i\u0000n\u0000e\u0000.\u0000 \u0000 \u0000P\u0000l\u0000e\u0000a\u0000s\u0000e\u0000 \u0000s\u0000e\u0000l\u0000e\u0000c\u0000t\u0000 \u0000t\u0000h\u0000e\u0000 \u0000l\u0000o\u0000c\u0000a\u0000t\u0000i\u0000o\u0000n\u0000 \u0000t\u0000o\u0000 \u0000i\u0000n\u0000s\u0000e\u0000r\u0000t\u0000!\u0000", "lxöN\u0016b!hÆQïSåNÒceQêS(W,{\u0000NT,{NL.\u0000\n\u0000÷\tébÒceQvMOn.\u0000", "XÕÜ´èÆ´Å@Æ \u0000P­\u0000ÉmÕ©º@Ç \u0000«Ìˆ¼øÉ@Æ \u0000P´ˆ¼øÉÐÅÌ¹ \u0000½À…Ç`Õ\u0018Â \u0000ˆÇµÂÈ²ä².\u0000\n\u0000½À…Ç`Õ \u0000\u0004ÇXÎ|¹ \u0000ä²ÜÂ \u0000 ÁÝÐXÕíÂÜÂ$Æ.\u0000"], ["H\u0000e\u0000r\u0000e\u0000,\u0000 \u0000i\u0000n\u0000s\u0000e\u0000r\u0000t\u0000 \u0000o\u0000n\u0000l\u0000y\u0000 \u0000H\u0000a\u0000r\u0000d\u0000w\u0000a\u0000r\u0000e\u0000.\u0000 \u0000 \u0000P\u0000l\u0000e\u0000a\u0000s\u0000e\u0000 \u0000r\u0000e\u0000t\u0000r\u0000y\u0000!\u0000", "(WÙÌ,\u0000ÒceQêS\tglxöN\u00020÷Q\u001d\\Õ\u0000NM!\u0000", "ìÅ0®ÐÅ”² \u0000XÕÜ´èÆ´ÅÌ¹ \u0000½À…Ç`Õ\u0018Â \u0000ˆÇµÂÈ²ä².\u0000 \u0000 \u0000ä²ÜÂ \u0000 ÁÝÐXÕíÂÜÂ$Æ!\u0000"], ["H\u0000e\u0000r\u0000e\u0000,\u0000 \u0000i\u0000n\u0000s\u0000e\u0000r\u0000t\u0000 \u0000o\u0000n\u0000l\u0000y\u0000 \u0000C\u0000a\u0000l\u0000i\u0000b\u0000r\u0000a\u0000t\u0000i\u0000o\u0000n\u0000.\u0000 \u0000 \u0000P\u0000l\u0000e\u0000a\u0000s\u0000e\u0000 \u0000r\u0000e\u0000t\u0000r\u0000y\u0000!\u0000", "(WÙÌ,\u0000ÒceQêS\tg!hÆQ\u00020÷Q\u001d\\Õ\u0000NM!\u0000", "ìÅ0®ÐÅ”² \u0000P­\u0000ÉmÕ©ºÌ¹ \u0000½À…Ç`Õ\u0018Â \u0000ˆÇµÂÈ²ä².\u0000 \u0000 \u0000ä²ÜÂ \u0000 ÁÝÐXÕíÂÜÂ$Æ!\u0000"], ["T\u0000h\u0000i\u0000s\u0000 \u0000s\u0000t\u0000e\u0000p\u0000 \u0000c\u0000a\u0000n\u0000 \u0000b\u0000e\u0000 \u0000i\u0000n\u0000s\u0000e\u0000r\u0000t\u0000e\u0000d\u0000 \u0000o\u0000n\u0000l\u0000y\u0000 \u0000u\u0000n\u0000d\u0000e\u0000r\u0000 \u0000C\u0000a\u0000l\u0000i\u0000b\u0000r\u0000a\u0000t\u0000i\u0000o\u0000n\u0000.\u0000", "Ù*Nek¤ïSåNÒceQêS\tg(W!hÆQ\u000bNb\u00020\n\u0000\u0000\u0000", "tÇ \u0000mÕ©º@Ç \u0000P­\u0000ÉmÕ©ºXÇ \u0000DÅ˜·½ÊÐÅÌ¹ \u0000½À…Ç`Õ\u0018Â \u0000ˆÇµÂÈ²ä².\u0000"], ["U\u0000p\u0000d\u0000a\u0000t\u0000i\u0000n\u0000g\u0000.\u0000.\u0000.\u0000", "ôf°e.\u0000.\u0000.\u0000", "1¬àÂ\u0011É.\u0000.\u0000.\u0000"], ["T\u0000h\u0000i\u0000s\u0000 \u0000s\u0000e\u0000q\u0000u\u0000e\u0000n\u0000c\u0000e\u0000 \u0000d\u0000o\u0000e\u0000s\u0000 \u0000n\u0000o\u0000t\u0000 \u0000e\u0000x\u0000i\u0000s\u0000t\u0000.\u0000", "Ù*N^\u0017R\rNX[(W.\u0000", "tÇ \u0000ü¬\u001cÈ,¸@Ç \u0000tÈ¬ÇXÕÀÉ \u0000JÅµÂÈ²ä².\u0000"], ["Y\u0000o\u0000u\u0000 \u0000a\u0000r\u0000e\u0000 \u0000i\u0000n\u0000s\u0000e\u0000r\u0000t\u0000i\u0000n\u0000g\u0000 \u0000a\u0000 \u0000s\u0000t\u0000e\u0000p\u0000 \u0000i\u0000n\u0000 \u0000t\u0000h\u0000e\u0000 \u0000m\u0000i\u0000d\u0000d\u0000l\u0000e\u0000 \u0000o\u0000f\u0000 \u0000a\u0000 \u0000j\u0000u\u0000m\u0000p\u0000.\u0000 \u0000D\u0000o\u0000 \u0000y\u0000o\u0000u\u0000 \u0000s\u0000t\u0000i\u0000l\u0000l\u0000 \u0000w\u0000a\u0000n\u0000t\u0000 \u0000t\u0000o\u0000 \u0000a\u0000d\u0000d\u0000 \u0000t\u0000h\u0000i\u0000s\u0000 \u0000s\u0000t\u0000e\u0000p\u0000?\u0000", "`OÒceQek¤(Wûy¨Rv-Nô\u00020Ø/f`Oó`ÒceQÙek¤l\u001fÿ", "tÇ‰ÕXÇ \u0000\u0011É\u0004¬ÐÅ \u0000¸ÓÑÉ0®|¹ \u0000|°ÌÆ#±à¬ˆÇµÂÈ²ä².\u0000 \u0000 \u0000ø­˜·Ä³ \u0000tÇ \u0000¸ÓÑÉ0®|¹ \u0000”Í\u0000¬XÕÜÂ ¬µÂÈ²L®?\u0000"], ["T\u0000h\u0000e\u0000 \u0000a\u0000c\u0000t\u0000i\u0000o\u0000n\u0000 \u0000y\u0000o\u0000u\u0000 \u0000a\u0000r\u0000e\u0000 \u0000a\u0000t\u0000t\u0000e\u0000m\u0000p\u0000t\u0000i\u0000n\u0000g\u0000 \u0000w\u0000i\u0000l\u0000l\u0000 \u0000b\u0000r\u0000e\u0000a\u0000k\u0000 \u0000o\u0000n\u0000e\u0000 \u0000o\u0000r\u0000 \u0000m\u0000o\u0000r\u0000e\u0000 \u0000j\u0000u\u0000m\u0000p\u0000s\u0000.\u0000 \u0000 \u0000D\u0000o\u0000 \u0000y\u0000o\u0000u\u0000 \u0000s\u0000t\u0000i\u0000l\u0000l\u0000 \u0000w\u0000a\u0000n\u0000t\u0000 \u0000t\u0000o\u0000 \u0000p\u0000e\u0000r\u0000f\u0000o\u0000r\u0000m\u0000 \u0000t\u0000h\u0000i\u0000s\u0000 \u0000a\u0000c\u0000t\u0000i\u0000o\u0000n\u0000?\u0000", "`OìN\u0012PbvL¨R\u0006\\\u001aOSb4x\u0000N*N\u0016b\u001aY*NóÃ\u00020`OØó`gbLÙ*N¨R\\O\u0017T?\u0000", "ù²àÂtÇ \u0000ÜÂÄ³XÕ”² \u0000Ù³‘Ç@Ç \u0000XÕ˜° \u00009Ö@Ç \u0000T³ \u0000Î¹@Ç \u0000tÇ‰ÕDÇ \u0000\fÓ4­`Õƒ¬…ÇÈ²ä².\u0000 \u0000 \u0000ø­˜·Ä³ \u0000tÇ \u0000Ù³‘ÇDÇ \u0000\u0018Â‰ÕXÕà¬öÂµÂÈ²L®?\u0000"], ["P\u0000l\u0000e\u0000a\u0000s\u0000e\u0000 \u0000s\u0000e\u0000l\u0000e\u0000c\u0000t\u0000 \u0000a\u0000n\u0000y\u0000 \u0000s\u0000t\u0000e\u0000p\u0000!\u0000", "÷\tébûNUO\u0000Nek¤!\u0000", "„ÇXÇXÇ \u0000¸ÓÑÉ0®|¹ \u0000 ÁÝÐXÕíÂÜÂ$Æ!\u0000"], ["T\u0000h\u0000i\u0000s\u0000 \u0000c\u0000a\u0000n\u0000n\u0000o\u0000t\u0000 \u0000b\u0000e\u0000 \u0000s\u0000e\u0000l\u0000e\u0000c\u0000t\u0000e\u0000d\u0000,\u0000 \u0000b\u0000e\u0000c\u0000a\u0000u\u0000s\u0000e\u0000 \u0000i\u0000t\u0000 \u0000i\u0000s\u0000 \u0000s\u0000t\u0000e\u0000p\u0000 \u0000o\u0000f\u0000 \u0000s\u0000u\u0000b\u0000 \u0000s\u0000e\u0000q\u0000u\u0000e\u0000n\u0000c\u0000e\u0000.\u0000 \u0000P\u0000l\u0000e\u0000a\u0000s\u0000e\u0000 \u0000s\u0000e\u0000l\u0000e\u0000c\u0000t\u0000 \u0000a\u0000n\u0000y\u0000 \u0000o\u0000t\u0000h\u0000e\u0000r\u0000 \u0000s\u0000t\u0000e\u0000p\u0000!\u0000", "Ù/fÝ~ù[\rNý«\téb\u00020÷\tébvQÖNv\u0000Nek¤!\u0000", "tÇƒ¬@Ç \u0000€½„½ü¬\u001cÈ,¸XÇ \u0000mÕ©ºtÇÀ»\\¸ \u0000 ÁÝÐ`Õ\u0018Â \u0000ÆÅµÂÈ²ä².\u0000 \u0000ä²x¹ \u0000\u0000³ÁÀDÇ \u0000 ÁÝÐXÕíÂÜÂ$Æ!\u0000"], ["T\u0000h\u0000i\u0000s\u0000 \u0000s\u0000e\u0000q\u0000u\u0000e\u0000n\u0000c\u0000e\u0000 \u0000c\u0000a\u0000n\u0000n\u0000o\u0000t\u0000 \u0000b\u0000e\u0000 \u0000i\u0000n\u0000s\u0000e\u0000r\u0000t\u0000e\u0000d\u0000 \u0000b\u0000e\u0000c\u0000a\u0000u\u0000s\u0000e\u0000 \u0000i\u0000t\u0000 \u0000c\u0000o\u0000n\u0000t\u0000a\u0000i\u0000n\u0000s\u0000 \u0000s\u0000u\u0000b\u0000s\u0000e\u0000q\u0000u\u0000e\u0000n\u0000c\u0000e\u0000.\u0000 \u0000P\u0000l\u0000e\u0000a\u0000s\u0000e\u0000 \u0000s\u0000e\u0000l\u0000e\u0000c\u0000t\u0000 \u0000a\u0000n\u0000y\u0000 \u0000o\u0000t\u0000h\u0000e\u0000r\u0000 \u0000s\u0000e\u0000q\u0000u\u0000e\u0000n\u0000c\u0000e\u0000!\u0000", "Ù*Nz^\rNýÒceQ,\u0000àV:N[\u0005S+TN\u000eTç~\u00020÷\tébvQÖN^\u0017R!\u0000", "tÇ \u0000ü¬\u001cÈ,¸@Ç \u0000€½„½ü¬\u001cÈ,¸DÇ \u0000ìÓhÕXÕà¬ˆÇ<ÇÀ»\\¸ \u0000|°ÌÆ#±DÇ\u0018Â \u0000ÆÅµÂÈ²ä².\u0000 \u0000ä²x¹ \u0000ü¬\u001cÈ,¸DÇ \u0000 ÁÝÐXÕíÂÜÂ$Æ!\u0000"], ["N\u0000o\u0000w\u0000 \u0000t\u0000h\u0000e\u0000r\u0000e\u0000 \u0000i\u0000s\u0000 \u0000n\u0000o\u0000t\u0000 \u0000s\u0000e\u0000l\u0000e\u0000c\u0000t\u0000e\u0000d\u0000 \u0000s\u0000t\u0000e\u0000p\u0000.\u0000 \u0000P\u0000l\u0000e\u0000a\u0000s\u0000e\u0000 \u0000s\u0000e\u0000l\u0000e\u0000c\u0000t\u0000 \u0000a\u0000n\u0000y\u0000 \u0000s\u0000t\u0000e\u0000p\u0000!\u0000", "°s(W\tg*g«\t-Nvek¤\u00020÷\tébûNUO\u0000Nek¤!\u0000", "\u0004Ö¬Ç \u0000 ÁÝÐ\u001c´ \u0000mÕ©ºtÇ \u0000ÆÅµÂÈ²ä².\u0000 \u0000„ÇXÇXÇ \u0000mÕ©ºDÇ \u0000 ÁÝÐXÕíÂÜÂ$Æ!\u0000"], ["P\u0000l\u0000e\u0000a\u0000s\u0000e\u0000,\u0000 \u0000s\u0000e\u0000t\u0000 \u0000u\u0000p\u0000 \u0000V\u0000I\u0000S\u0000A\u0000 \u0000d\u0000r\u0000i\u0000v\u0000e\u0000r\u0000.\u0000", "÷¾nV\u0000I\u0000S\u0000A\u0000q¨RoöN.\u0000", "D¾¬Àl­Ù³\u0004Õ\\¸ø­Œ·DÇ \u0000$ÁXÎXÕíÂÜÂ$Æ.\u0000"], ["B\u0000e\u0000c\u0000a\u0000u\u0000s\u0000e\u0000 \u0000t\u0000h\u0000i\u0000s\u0000 \u0000p\u0000r\u0000o\u0000g\u0000r\u0000a\u0000m\u0000 \u0000i\u0000s\u0000 \u0000t\u0000r\u0000i\u0000a\u0000l\u0000 \u0000v\u0000e\u0000r\u0000s\u0000i\u0000o\u0000n\u0000,\u0000 \u0000c\u0000a\u0000n\u0000n\u0000o\u0000t\u0000 \u0000b\u0000e\u0000 \u0000s\u0000a\u0000v\u0000e\u0000d\u0000 \u0000t\u0000h\u0000e\u0000 \u0000S\u0000e\u0000q\u0000u\u0000e\u0000n\u0000c\u0000e\u0000 \u0000a\u0000n\u0000d\u0000 \u0000S\u0000t\u0000e\u0000p\u0000 \u0000d\u0000a\u0000t\u0000a\u0000!\u0000", "àV:NÙ*N\u000bz^/fÕ(uHr,\u0000 \u0000\rNýÝOX[^\u0017RTek¤vpenc!\u0000", "tÇ \u0000\u0004Õ\\¸ø­·@Ç \u0000ÜÂØÕ\u0010ÓtÇÀ»\\¸ \u0000ü¬\u001cÈ,¸ü¬ \u0000ü¬\u001cÈmÕ©ºÇÌ¸|¹ \u0000ô¼\u0000­`Õ\u0018Â \u0000ÆÅµÂÈ²ä²!\u0000"], ["T\u0000h\u0000e\u0000 \u0000a\u0000c\u0000t\u0000i\u0000o\u0000n\u0000 \u0000y\u0000o\u0000u\u0000 \u0000a\u0000r\u0000e\u0000 \u0000a\u0000t\u0000t\u0000e\u0000m\u0000p\u0000t\u0000i\u0000n\u0000g\u0000 \u0000c\u0000a\u0000n\u0000n\u0000o\u0000t\u0000 \u0000b\u0000e\u0000 \u0000p\u0000e\u0000r\u0000f\u0000o\u0000r\u0000m\u0000a\u0000n\u0000c\u0000e\u0000d\u0000,\u0000 \u0000b\u0000e\u0000c\u0000a\u0000u\u0000s\u0000e\u0000 \u0000y\u0000o\u0000u\u0000 \u0000a\u0000r\u0000e\u0000 \u0000i\u0000n\u0000s\u0000e\u0000r\u0000t\u0000i\u0000n\u0000g\u0000 \u0000a\u0000 \u0000j\u0000u\u0000m\u0000p\u0000 \u0000i\u0000n\u0000 \u0000t\u0000h\u0000e\u0000 \u0000m\u0000i\u0000d\u0000d\u0000l\u0000e\u0000 \u0000o\u0000f\u0000 \u0000a\u0000 \u0000j\u0000u\u0000m\u0000p\u0000!\u0000", "(WóÃv-Nô\rNýÒceQæS\u0016Y\u0000N*NóÃ\u00020", "tÇ‰ÕXÇ \u0000\u0011É\u0004¬ÐÅ \u0000\u0010¶ \u0000ä²x¹ \u0000tÇ‰ÕDÇ \u0000|°ÌÆ#±”² \u0000Ù³‘Ç@Ç \u0000\u0018Â‰Õ ´\u0018Â \u0000ÆÅµÂÈ²ä²!\u0000"], ["P\u0000l\u0000e\u0000a\u0000s\u0000e\u0000,\u0000 \u0000i\u0000n\u0000p\u0000u\u0000t\u0000 \u0000s\u0000t\u0000e\u0000p\u0000 \u0000n\u0000a\u0000m\u0000e\u0000 \u0000c\u0000o\u0000r\u0000r\u0000e\u0000c\u0000t\u0000l\u0000y\u0000.\u0000", "÷eQcknxvek¤\rTW[.\u0000", "mÕ©ºtÇ„¹DÇ \u0000\u0015ÈUÖˆ× \u0000…Ç%¸XÕíÂÜÂ$Æ.\u0000"], ["B\u0000a\u0000c\u0000a\u0000u\u0000s\u0000e\u0000 \u0000t\u0000h\u0000i\u0000s\u0000 \u0000p\u0000r\u0000o\u0000g\u0000r\u0000a\u0000m\u0000 \u0000i\u0000s\u0000 \u0000t\u0000r\u0000i\u0000a\u0000l\u0000 \u0000v\u0000e\u0000r\u0000s\u0000i\u0000n\u0000,\u0000 \u0000t\u0000h\u0000e\u0000 \u0000s\u0000e\u0000q\u0000u\u0000e\u0000n\u0000c\u0000e\u0000 \u0000c\u0000a\u0000n\u0000n\u0000o\u0000t\u0000 \u0000b\u0000e\u0000 \u0000r\u0000u\u0000n\u0000n\u0000e\u0000d\u0000!\u0000", "àV:NÙ*N\u000bz^/fÕ(uHr\fÿ^\u0017R\rNýÐL!\u0000", "tÇ \u0000\u0004Õ\\¸ø­Œ·@Ç \u0000äÂØÕ\u0010ÓtÇÀ»\\¸ \u0000ü¬\u001cÈ,¸DÇ \u0000äÂ‰Õ`Õ\u0018ÂÆÅµÂÈ²ä²!\u0000"]] string[][] [["W\u0000r\u0000o\u0000n\u0000g\u0000 \u0000d\u0000a\u0000t\u0000a\u0000 \u0000t\u0000y\u0000p\u0000e\u0000 \u0000n\u0000a\u0000m\u0000e\u0000 \u0000f\u0000o\u0000r\u0000 \u0000t\u0000h\u0000i\u0000s\u0000 \u0000c\u0000o\u0000n\u0000v\u0000e\u0000r\u0000s\u0000i\u0000o\u0000n\u0000 \u0000V\u0000I\u0000.\u0000", "dkHr,gV\u0000I\u0000„vpenc{|‹W\u0019•ï‹.\u0000", "ÇÌ¸\u0015ÖÝÂtÇ \u0000ÀÒ½¹È²ä².\u0000"]] string[][] [["S\u0000o\u0000m\u0000e\u0000 \u0000o\u0000f\u0000 \u0000t\u0000h\u0000e\u0000 \u0000s\u0000e\u0000l\u0000e\u0000c\u0000t\u0000e\u0000d\u0000 \u0000d\u0000a\u0000t\u0000a\u0000 \u0000a\u0000r\u0000e\u0000 \u0000a\u0000l\u0000r\u0000e\u0000a\u0000d\u0000y\u0000 \u0000p\u0000r\u0000o\u0000t\u0000e\u0000c\u0000t\u0000e\u0000d\u0000!\u0000", "\t[v\u0000NNpencò]Ï~ÝO¤b!\u0000", " ÁÝÐ\u001c´ \u0000ÇÌ¸XÇ \u0000|Ç½\u0000¬ \u0000tÇø» \u0000ÇÌ¸ô¼8Ö\u0018´\u0000ÆµÂÈ²ä².\u0000"], ["A\u0000r\u0000e\u0000 \u0000y\u0000o\u0000u\u0000 \u0000s\u0000u\u0000r\u0000e\u0000 \u0000y\u0000o\u0000u\u0000 \u0000w\u0000a\u0000n\u0000t\u0000 \u0000t\u0000o\u0000 \u0000d\u0000e\u0000l\u0000e\u0000t\u0000e\u0000 \u0000t\u0000h\u0000e\u0000 \u0000s\u0000e\u0000l\u0000e\u0000t\u0000e\u0000d\u0000\n\u0000d\u0000a\u0000t\u0000a\u0000 \u0000f\u0000r\u0000o\u0000m\u0000 \u0000C\u0000u\u0000r\u0000v\u0000e\u0000 \u0000L\u0000i\u0000b\u0000r\u0000a\u0000r\u0000y\u0000?\u0000 \u0000", "`Onx[ Rdvò]\t\n\u0000ÎNòf¿~^vpenc?\u0000", "á¬ Á\u001cÁà¬ÐÅ\u001cÁ \u0000 ÁÝÐ\u001c´ \u0000ÇÌ¸|¹ \u0000ÀÉ°Æ ¬µÂÈ²L®?\u0000"], ["U\u0000n\u0000p\u0000r\u0000o\u0000t\u0000e\u0000c\u0000t\u0000i\u0000n\u0000g\u0000 \u0000c\u0000u\u0000r\u0000v\u0000e\u0000s\u0000 \u0000w\u0000i\u0000l\u0000l\u0000 \u0000d\u0000e\u0000l\u0000e\u0000t\u0000e\u0000 \u0000a\u0000n\u0000y\u0000 \u0000d\u0000a\u0000t\u0000a\u0000 \u0000\n\u0000t\u0000h\u0000a\u0000t\u0000 \u0000i\u0000s\u0000 \u0000n\u0000o\u0000t\u0000 \u0000a\u0000s\u0000s\u0000o\u0000c\u0000i\u0000a\u0000t\u0000e\u0000d\u0000 \u0000w\u0000i\u0000t\u0000h\u0000 \u0000t\u0000h\u0000e\u0000 \u0000c\u0000u\u0000r\u0000r\u0000r\u0000e\u0000n\u0000t\u0000 \u0000s\u0000e\u0000q\u0000u\u0000e\u0000n\u0000c\u0000e\u0000.\u0000", "ãdÝO¤bòf¿~\u0006\\ RdûNUOpenc\n\u0000Ù/f\rNøvsQvS_MR^\u0017R.\u0000", "ÇÌ¸ô¼8ÖtÕ\u001cÈ² \u0000\u0004Ö¬ÇXÇ \u0000ü¬\u001cÈ,¸ü¬ \u0000(¸\u0000­\u0018´ÀÉJÅ@Ç\n\u0000ÇÌ¸|¹ \u0000ÀÉ¸Æ¬ÇÈ²ä².\u0000"], ["Y\u0000o\u0000u\u0000 \u0000m\u0000a\u0000y\u0000 \u0000n\u0000o\u0000t\u0000 \u0000s\u0000e\u0000l\u0000e\u0000c\u0000t\u0000 \u0000m\u0000o\u0000r\u0000e\u0000 \u0000t\u0000h\u0000a\u0000n\u0000 \u0000t\u0000w\u0000o\u0000 \u0000w\u0000a\u0000v\u0000e\u0000f\u0000o\u0000r\u0000m\u0000s\u0000 \u0000t\u0000o\u0000 \u0000s\u0000a\u0000v\u0000e\u0000 \u0000t\u0000o\u0000 \u0000a\u0000 \u0000s\u0000i\u0000n\u0000g\u0000l\u0000e\u0000 \u0000W\u0000A\u0000V\u0000 \u0000f\u0000i\u0000l\u0000e\u0000.\u0000", "`OïSý\rN\téb$N*NåN\nNvâlb_ÝOX[0R\u0000N*NUS\u0000NvW\u0000A\u0000V\u0000eöN.\u0000", "\\Õ\u001c¬XÇ \u0000W\u0000A\u0000V\u0000\fÓ|ÇÐÅ \u0000P´\u001c¬tÇÁÀXÇ \u0000ÜÂ\u0004¬\fÓ\u0015ÖDÇ \u0000\n\u0000ô¼\u0000­`Õ\u0018Â \u0000ÆÅµÂÈ²ä².\u0000"], ["W\u0000a\u0000v\u0000e\u0000 \u0000f\u0000i\u0000l\u0000e\u0000 \u0000s\u0000a\u0000v\u0000e\u0000 \u0000e\u0000r\u0000r\u0000o\u0000r\u0000!\u0000", "W\u0000a\u0000v\u0000e\u0000‡eöNÝOX[\u0019•ï‹!\u0000", "W\u0000a\u0000v\u0000e\u0000\fÓ|Çô¼\u0000­ \u0000$Æ Ç!\u0000"], ["C\u0000a\u0000n\u0000n\u0000o\u0000t\u0000 \u0000a\u0000p\u0000p\u0000e\u0000n\u0000d\u0000 \u0000i\u0000n\u0000 \u0000t\u0000h\u0000e\u0000 \u0000c\u0000a\u0000s\u0000e\u0000 \u0000o\u0000f\u0000 \u0000w\u0000a\u0000v\u0000e\u0000f\u0000o\u0000r\u0000m\u0000.\u0000", "(Wâlb_vÅ`µQ\u000bN\rNýý R.\u0000", "W\u0000a\u0000v\u0000e\u0000\fÓ|ÇÐÅ”² \u0000”Í\u0000¬`Õ\u0018Â \u0000ÆÅµÂÈ²ä².\u0000"], ["C\u0000h\u0000a\u0000n\u0000n\u0000e\u0000l\u0000 \u0000n\u0000u\u0000m\u0000b\u0000e\u0000r\u0000 \u0000i\u0000s\u0000 \u0000w\u0000r\u0000o\u0000n\u0000g\u0000.\u0000", "\u001aS÷S\u0001x/f\u0019ïv.\u0000", "µÑ\\¸ˆ¼8Ö\u0000¬ \u0000ÀÒ½¹È²ä².\u0000"], ["W\u0000a\u0000v\u0000e\u0000 \u0000f\u0000i\u0000l\u0000e\u0000 \u0000o\u0000p\u0000e\u0000n\u0000 \u0000e\u0000r\u0000r\u0000o\u0000r\u0000!\u0000", "W\u0000a\u0000v\u0000e\u0000‡eöNSb\u0000_\u0019•ï‹!\u0000", "W\u0000a\u0000v\u0000e\u0000\fÓ|ÇôÅ0® \u0000$Æ Ç!\u0000"], [" \u0000C\u0000a\u0000n\u0000n\u0000o\u0000t\u0000 \u0000u\u0000n\u0000d\u0000e\u0000r\u0000s\u0000t\u0000a\u0000n\u0000d\u0000 \u0000t\u0000x\u0000t\u0000 \u0000f\u0000i\u0000l\u0000e\u0000 \u0000f\u0000o\u0000r\u0000m\u0000a\u0000t\u0000.\u0000", "àeÕl\u0006tã‰t\u0000x\u0000t\u0000‡eöN<h\u000f_.\u0000", "t\u0000x\u0000t\u0000\fÓ|Ç\u0015ÖÝÂDÇ \u0000¬¹tÕ`Õ\u0018Â \u0000ÆÅµÂÈ²ä².\u0000 \u0000"], ["C\u0000a\u0000n\u0000n\u0000o\u0000t\u0000 \u0000p\u0000l\u0000o\u0000t\u0000 \u0000t\u0000h\u0000e\u0000s\u0000e\u0000 \u0000d\u0000a\u0000t\u0000a\u0000 \u0000t\u0000o\u0000g\u0000e\u0000t\u0000h\u0000e\u0000r\u0000 \u0000!\u0000\n\u0000Y\u0000o\u0000u\u0000 \u0000m\u0000u\u0000s\u0000t\u0000 \u0000s\u0000e\u0000l\u0000e\u0000c\u0000t\u0000 \u0000c\u0000u\u0000r\u0000v\u0000e\u0000s\u0000 \u0000w\u0000i\u0000t\u0000h\u0000 \u0000a\u0000 \u0000m\u0000a\u0000x\u0000i\u0000m\u0000u\u0000m\u0000 \u0000o\u0000f\u0000 \u0000t\u0000w\u0000o\u0000 \u0000d\u0000i\u0000f\u0000f\u0000e\u0000r\u0000e\u0000n\u0000t\u0000 \u0000u\u0000n\u0000i\u0000t\u0000 \u0000s\u0000e\u0000t\u0000s\u0000,\u0000 \u0000i\u0000n\u0000c\u0000l\u0000u\u0000d\u0000i\u0000n\u0000g\u0000 \u0000p\u0000h\u0000a\u0000s\u0000e\u0000.\u0000", "\rNý\u0000Nw>f:yÙNpenc!\u0000\n\u0000¨`Å_{\téb\u0000g\u001aYv$N*N\rN\fTvUSMOvòf¿~.\u0000", "tÇð· \u0000ÇÌ¸² \u0000\u0019¬tÇ \u0000ô¼ìÅ\u0004É\u0018Â \u0000ÆÅµÂÈ²ä².\u0000\n\u0000\u0004ÇÁÀDÇ \u0000ìÓhÕXÕìÅ \u0000\\Í\u0000³ \u00002\u0000\u001c¬XÇ \u0000\u001cÁ\\¸ä²x¹ \u0000è²\u0004Ç|¹ \u0000\u0000¬ÄÉ \u0000ÇÌ¸|¹ \u0000 ÁÝÐXÕíÂÜÂ$Æ.\u0000"], ["C\u0000a\u0000n\u0000n\u0000o\u0000t\u0000 \u0000p\u0000l\u0000o\u0000t\u0000 \u0000t\u0000h\u0000e\u0000s\u0000e\u0000 \u0000d\u0000a\u0000t\u0000a\u0000 \u0000t\u0000o\u0000g\u0000e\u0000t\u0000h\u0000e\u0000r\u0000 \u0000!\u0000\n\u0000Y\u0000o\u0000u\u0000 \u0000m\u0000u\u0000s\u0000t\u0000 \u0000s\u0000e\u0000l\u0000e\u0000c\u0000t\u0000 \u0000W\u0000a\u0000v\u0000e\u0000f\u0000o\u0000r\u0000m\u0000s\u0000 \u0000w\u0000i\u0000t\u0000h\u0000 \u0000a\u0000 \u0000m\u0000a\u0000x\u0000i\u0000m\u0000u\u0000m\u0000 \u0000o\u0000f\u0000 \u0000t\u0000w\u0000o\u0000 \u0000d\u0000i\u0000f\u0000f\u0000e\u0000r\u0000e\u0000n\u0000t\u0000 \u0000u\u0000n\u0000i\u0000t\u0000 \u0000s\u0000e\u0000t\u0000s\u0000,\u0000 \u0000i\u0000n\u0000c\u0000l\u0000u\u0000d\u0000i\u0000n\u0000g\u0000 \u0000p\u0000h\u0000a\u0000s\u0000e\u0000.\u0000", "\rNý\u0000NwØ~6RÙNpenc!\u0000\n\u0000¨`Å_{\téb\u0000g'Yv$N*N\rN\fTvUSMOÆvâlb_.\u0000", "tÇð· \u0000ÇÌ¸² \u0000\u0019¬tÇ \u0000ô¼ìÅ\u0004É\u0018Â \u0000ÆÅµÂÈ²ä².\u0000\n\u0000\u0004ÇÁÀDÇ \u0000ìÓhÕXÕìÅ \u0000\\Í\u0000³ \u00002\u0000\u001c¬XÇ \u0000 \u0000\u001cÁ\\¸ä²x¹ \u0000è²\u0004Ç|¹ \u0000\u0000¬ÄÉ \u0000ÜÂ\u0004¬\fÓ\u0015ÖDÇ \u0000 ÁÝÐXÕíÂÜÂ$Æ.\u0000"], ["C\u0000a\u0000n\u0000n\u0000o\u0000t\u0000 \u0000p\u0000l\u0000o\u0000t\u0000 \u0000m\u0000o\u0000r\u0000e\u0000 \u0000t\u0000h\u0000a\u0000n\u0000 \u0000o\u0000n\u0000e\u0000 \u0000w\u0000a\u0000v\u0000e\u0000f\u0000o\u0000r\u0000m\u0000 \u0000 \u0000i\u0000n\u0000 \u0000i\u0000n\u0000t\u0000e\u0000n\u0000s\u0000i\u0000t\u0000y\u0000 \u0000g\u0000r\u0000a\u0000p\u0000h\u0000.\u0000", "\rNý€Ø~6R\u0000N*NåN\nN„v:_¦^þV„vâlb_.\u0000", "\u0000¼Ä³ø­|·\u0004ÕÐÅ”² \u0000\\Õ\u001c¬tÇÁÀXÇ \u0000ÜÂ\u0004¬\fÓ\u0015ÖDÇ \u0000‘ÇÄ³`Õ\u0018Â \u0000ÆÅµÂÈ²ä².\u0000"], ["D\u0000a\u0000t\u0000a\u0000 \u0000f\u0000o\u0000r\u0000m\u0000a\u0000t\u0000 \u0000i\u0000s\u0000 \u0000w\u0000r\u0000o\u0000n\u0000g\u0000.\u0000", "penc/f\u0019•ï‹„v.\u0000", "ÇÌ¸\u0015ÖÝÂtÇ \u0000ÀÒ½¹È²ä².\u0000"], ["C\u0000a\u0000l\u0000i\u0000b\u0000r\u0000a\u0000t\u0000i\u0000o\u0000n\u0000 \u0000d\u0000a\u0000t\u0000a\u0000 \u0000c\u0000a\u0000n\u0000n\u0000o\u0000t\u0000 \u0000b\u0000e\u0000 \u0000d\u0000e\u0000l\u0000e\u0000t\u0000e\u0000d\u0000.\u0000", "!hÆQòf¿~\rNý€ Rd–.\u0000", "P­\u0000ÉÇÌ¸² \u0000ÀÉ¸Æ\u0018Â \u0000ÆÅµÂÈ²ä².\u0000"], ["O\u0000n\u0000l\u0000y\u0000 \u0000o\u0000n\u0000e\u0000 \u0000d\u0000a\u0000t\u0000a\u0000 \u0000c\u0000a\u0000n\u0000 \u0000b\u0000e\u0000 \u0000i\u0000m\u0000p\u0000o\u0000r\u0000t\u0000e\u0000d\u0000.\u0000", "êS\tg\u0000N*NpencïSåNü[eQ.\u0000", "\\Õ\u001c¬XÇ \u0000ÇÌ¸Ì¹DÇ \u0000Çl­`Õ\u0018Â \u0000ÇµÂÈ²ä².\u0000"], ["T\u0000h\u0000i\u0000s\u0000 \u0000d\u0000a\u0000t\u0000a\u0000 \u0000i\u0000s\u0000 \u0000n\u0000o\u0000t\u0000 \u0000d\u0000i\u0000g\u0000i\u0000t\u0000a\u0000l\u0000 \u0000d\u0000a\u0000t\u0000a\u0000.\u0000", "ÙNpenc\rN/fpeW[penc\u00020", "tÇ \u0000ÇÌ¸² \u0000\u0018ÂÇàÂ8ÖÇÌ¸\u0000¬ \u0000DÅÙ²È²ä².\u0000"], ["P\u0000l\u0000e\u0000a\u0000s\u0000e\u0000,\u0000 \u0000i\u0000n\u0000p\u0000u\u0000t\u0000 \u0000n\u0000a\u0000m\u0000e\u0000 \u0000c\u0000o\u0000r\u0000r\u0000e\u0000c\u0000t\u0000l\u0000y\u0000.\u0000", "÷eQcknxv\rTW[", "tÇ„¹DÇ \u0000\u0015ÈUÖˆ× \u0000…Ç%¸XÕíÂÜÂ$Æ.\u0000"], ["C\u0000a\u0000n\u0000'\u0000t\u0000 \u0000r\u0000e\u0000n\u0000a\u0000m\u0000e\u0000 \u0000g\u0000r\u0000o\u0000u\u0000p\u0000 \u0000t\u0000o\u0000 \u0000a\u0000 \u0000C\u0000u\u0000r\u0000v\u0000e\u0000 \u0000L\u0000i\u0000b\u0000r\u0000a\u0000r\u0000y\u0000 \u0000i\u0000t\u0000e\u0000m\u0000 \u0000w\u0000h\u0000i\u0000c\u0000h\u0000 \u0000a\u0000l\u0000r\u0000e\u0000a\u0000d\u0000y\u0000 \u0000e\u0000x\u0000i\u0000s\u0000t\u0000s\u0000.\u0000", "\rNý€Í‘}T\rTÄ~ò]Ï~X[(W„vòf¿~“^y˜îv.\u0000", "tÇø» \u0000tÈ¬ÇXÕ”² \u0000á¬ Á\u001cÁà¬mÕ©º<Ç\\¸ \u0000ø­ù¸tÇ„¹DÇ \u0000À¼½¬`Õ\u0018Â \u0000ÆÅµÂÈ²ä².\u0000"]] string[][] [["M\u0000i\u0000c\u0000r\u0000o\u0000s\u0000o\u0000f\u0000t\u0000 \u0000O\u0000f\u0000f\u0000i\u0000c\u0000e\u0000 \u0000W\u0000o\u0000r\u0000d\u0000 \u0000i\u0000s\u0000 \u0000n\u0000o\u0000t\u0000 \u0000i\u0000n\u0000s\u0000t\u0000a\u0000l\u0000l\u0000e\u0000d\u0000.\u0000\n\u0000P\u0000l\u0000e\u0000a\u0000s\u0000e\u0000 \u0000i\u0000n\u0000s\u0000t\u0000a\u0000l\u0000l\u0000 \u0000M\u0000i\u0000c\u0000r\u0000o\u0000s\u0000o\u0000f\u0000t\u0000 \u0000O\u0000f\u0000f\u0000i\u0000c\u0000e\u0000 \u0000W\u0000o\u0000r\u0000d\u0000.\u0000", "®_oRlQUSÍ/f¡l\tg[Å\u00020÷[Å®_oRlQvÝ\u00020", "\\ÔÄ¬°À\u0004Õ\\¸ø­Œ·tÇ \u0000$ÁXÎ\u0018´ÀÉJÅXÅµÂÈ²ä².\u0000\n\u0000\\ÔÄ¬°À\u0004Õ\\¸ø­Œ·DÇ \u0000$ÁXÎXÕà¬ \u0000¬¹©ÆXÕíÂÜÂ$Æ.\u0000"], ["S\u0000t\u0000o\u0000p\u0000 \u0000F\u0000r\u0000e\u0000q\u0000 \u0000m\u0000u\u0000s\u0000t\u0000 \u0000b\u0000e\u0000 \u0000n\u0000o\u0000t\u0000 \u0000l\u0000a\u0000r\u0000g\u0000e\u0000r\u0000 \u0000t\u0000h\u0000a\u0000n\u0000 \u0000S\u0000t\u0000a\u0000r\u0000t\u0000 \u0000F\u0000r\u0000e\u0000q\u0000.\u0000", "\\PbksÅ_{\rNÇ\u0000_ËYvs\u00020", "\u0015ÈÀÉüÈ\fÓ\u0018Â”² \u0000ÜÂ‘ÇüÈ\fÓ\u0018Âô¼ä² \u0000lÐÀÉ \u0000Ð¹DÅ|Å \u0000iÕÈ²ä².\u0000"]] string[][] [["S\u0000t\u0000e\u0000p\u0000 \u0000a\u0000d\u0000d\u0000i\u0000n\u0000g\u0000.\u0000.\u0000.\u0000", "ek¤šûm R.\u0000.\u0000.\u0000", "mÕ©º”Í\u0000¬\u0011É.\u0000.\u0000.\u0000"], ["R\u0000e\u0000f\u0000r\u0000e\u0000s\u0000h\u0000i\u0000n\u0000g\u0000.\u0000.\u0000.\u0000", "7R°e.\u0000.\u0000.\u0000", "ŒÖõ¼\u0011É.\u0000.\u0000.\u0000"], ["U\u0000p\u0000d\u0000a\u0000t\u0000i\u0000n\u0000g\u0000.\u0000.\u0000.\u0000", "ôf°e.\u0000.\u0000.\u0000", "1¬àÂ\u0011É.\u0000.\u0000.\u0000"], ["T\u0000h\u0000i\u0000s\u0000 \u0000u\u0000s\u0000e\u0000r\u0000 \u0000c\u0000a\u0000n\u0000'\u0000t\u0000 \u0000a\u0000d\u0000d\u0000 \u0000s\u0000t\u0000e\u0000p\u0000.\u0000", "Ù*N(u7b\rNý R\u0000Nek¤\u00020", "tÇ \u0000¬À©ÆÇ² \u0000ü¬\u001cÈmÕ©ºDÇ \u0000Í\u0000¬`Õ\u0018Â \u0000ÆÅµÂÈ²ä².\u0000"], ["T\u0000h\u0000i\u0000s\u0000 \u0000s\u0000t\u0000e\u0000p\u0000 \u0000c\u0000a\u0000n\u0000'\u0000t\u0000 \u0000d\u0000e\u0000l\u0000e\u0000t\u0000e\u0000 \u0000b\u0000e\u0000c\u0000a\u0000u\u0000s\u0000e\u0000 \u0000i\u0000t\u0000 \u0000i\u0000s\u0000 \u0000d\u0000e\u0000f\u0000a\u0000u\u0000l\u0000t\u0000!\u0000", "Ù\u0000Nek¤_N\rNý Rd,\u0000àV:N[/fØ¤v!\u0000", "tÇ \u0000ü¬\u001cÈmÕ©º@Ç \u00000®tÈ$Á\u0015ÈtÇÀ»\\¸ \u0000­À\u001cÈ`Õ\u0018Â \u0000ÆÅµÂÈ²ä²!\u0000"], ["D\u0000o\u0000 \u0000y\u0000o\u0000u\u0000 \u0000w\u0000a\u0000n\u0000t\u0000 \u0000t\u0000o\u0000 \u0000d\u0000e\u0000l\u0000e\u0000t\u0000e\u0000 \u0000%\u0000s\u0000 \u0000s\u0000t\u0000e\u0000p\u0000?\u0000", "`O Rd \u0000%\u0000s\u0000ek¤\u0017T?\u0000", "%\u0000s\u0000 \u0000mÕ©ºDÇ \u0000­À\u001cÈXÕ ¬µÂÈ²L®?\u0000"], ["D\u0000o\u0000 \u0000y\u0000o\u0000u\u0000 \u0000w\u0000a\u0000n\u0000t\u0000 \u0000t\u0000o\u0000 \u0000d\u0000e\u0000l\u0000e\u0000t\u0000e\u0000 \u0000%\u0000s\u0000 \u0000s\u0000e\u0000q\u0000u\u0000e\u0000n\u0000c\u0000e\u0000?\u0000", "`O Rd \u0000%\u0000s\u0000 \u0000^\u0017R\u0017T?\u0000", "%\u0000s\u0000 \u0000ü¬\u001cÈ|¹ \u0000­À\u001cÈXÕ ¬µÂÈ²L®?\u0000"], ["N\u0000o\u0000w\u0000 \u0000t\u0000h\u0000e\u0000r\u0000e\u0000 \u0000i\u0000s\u0000 \u0000n\u0000o\u0000t\u0000 \u0000s\u0000e\u0000l\u0000e\u0000c\u0000t\u0000e\u0000d\u0000 \u0000s\u0000t\u0000e\u0000p\u0000.\u0000 \u0000P\u0000l\u0000e\u0000a\u0000s\u0000e\u0000 \u0000s\u0000e\u0000l\u0000e\u0000c\u0000t\u0000 \u0000a\u0000n\u0000y\u0000 \u0000s\u0000t\u0000e\u0000p\u0000!\u0000", "°s(W\tg*g«\t-Nvek¤\u00020÷\tébûNUO\u0000Nek¤!\u0000\n\u0000\u0000\u0000", "\u0004Ö¬Ç \u0000 ÁÝÐ\u001c´ \u0000mÕ©ºtÇ \u0000ÆÅµÂÈ²ä².\u0000 \u0000„ÇXÇXÇ \u0000mÕ©ºDÇ \u0000 ÁÝÐXÕíÂÜÂ$Æ!\u0000"], ["T\u0000h\u0000i\u0000s\u0000 \u0000s\u0000t\u0000e\u0000p\u0000 \u0000c\u0000a\u0000n\u0000n\u0000o\u0000t\u0000 \u0000b\u0000e\u0000 \u0000s\u0000e\u0000l\u0000e\u0000c\u0000t\u0000e\u0000d\u0000,\u0000 \u0000b\u0000e\u0000c\u0000a\u0000u\u0000s\u0000e\u0000 \u0000i\u0000t\u0000 \u0000h\u0000a\u0000s\u0000 \u0000w\u0000r\u0000o\u0000n\u0000g\u0000 \u0000d\u0000a\u0000t\u0000a\u0000 \u0000t\u0000y\u0000p\u0000e\u0000.\u0000 \u0000P\u0000l\u0000e\u0000a\u0000s\u0000e\u0000 \u0000s\u0000e\u0000l\u0000e\u0000c\u0000t\u0000 \u0000a\u0000n\u0000y\u0000 \u0000o\u0000t\u0000h\u0000e\u0000r\u0000 \u0000s\u0000t\u0000e\u0000p\u0000!\u0000", "àeÕl\tébàV:NÙ*Nyîvvpenc<h\u000f_\u0019ï\u00020÷\tébvQÖNûNUO\u0000Nek¤!\u0000", "tÇ \u0000mÕ©º@Ç \u0000ÇÌ¸\u0015ÖÝÂtÇ \u0000Ç»º\u0018´\u0000Æ<ÇÀ»\\¸ \u0000 ÁÝÐ`Õ\u0018Â \u0000ÆÅµÂÈ²ä².\u0000 \u0000ä²x¹ \u0000mÕ©ºDÇ \u0000 ÁÝÐXÕíÂÜÂ$Æ!\u0000"], ["B\u0000e\u0000c\u0000a\u0000u\u0000s\u0000e\u0000 \u0000t\u0000h\u0000i\u0000s\u0000 \u0000p\u0000r\u0000o\u0000g\u0000r\u0000a\u0000m\u0000 \u0000i\u0000s\u0000 \u0000t\u0000r\u0000i\u0000a\u0000l\u0000 \u0000v\u0000e\u0000r\u0000s\u0000i\u0000o\u0000n\u0000,\u0000 \u0000c\u0000a\u0000n\u0000n\u0000o\u0000t\u0000 \u0000b\u0000e\u0000 \u0000a\u0000d\u0000d\u0000e\u0000d\u0000!\u0000", "àV:NÙ*N\u000bz^/fÕ(uHr,\u0000 \u0000\rNý Rz^Tek¤vpenc!\u0000", "tÇ \u0000\u0004Õ\\¸ø­Œ·@Ç \u0000ÜÂØÕ\u0010ÓtÇÀ»\\¸ \u0000”Í\u0000¬`Õ\u0018ÂÆÅµÂÈ²ä²!\u0000"], ["T\u0000h\u0000i\u0000s\u0000 \u0000V\u0000I\u0000 \u0000f\u0000i\u0000l\u0000e\u0000 \u0000d\u0000o\u0000e\u0000s\u0000 \u0000n\u0000o\u0000t\u0000 \u0000e\u0000x\u0000i\u0000s\u0000t\u0000.\u0000", "ÙV\u0000I\u0000eöN¡l\tgX[(W.\u0000", "tÇ \u0000V\u0000I\u0000\fÓ|Ç@Ç \u0000tÈ¬ÇXÕÀÉ \u0000JÅµÂÈ²ä².\u0000"], ["W\u0000h\u0000e\u0000n\u0000 \u0000c\u0000u\u0000r\u0000v\u0000e\u0000 \u0000l\u0000i\u0000b\u0000r\u0000a\u0000r\u0000y\u0000 \u0000i\u0000s\u0000 \u0000a\u0000u\u0000t\u0000o\u0000g\u0000r\u0000o\u0000u\u0000p\u0000i\u0000n\u0000g\u0000,\u0000 \u0000t\u0000h\u0000e\u0000 \u0000s\u0000e\u0000q\u0000u\u0000e\u0000n\u0000c\u0000e\u0000 \u0000c\u0000a\u0000n\u0000n\u0000o\u0000t\u0000 \u0000b\u0000e\u0000 \u0000i\u0000n\u0000s\u0000e\u0000r\u0000t\u0000e\u0000d\u0000.\u0000 \u0000I\u0000f\u0000 \u0000y\u0000o\u0000u\u0000 \u0000i\u0000n\u0000s\u0000e\u0000r\u0000t\u0000 \u0000s\u0000e\u0000q\u0000u\u0000e\u0000n\u0000c\u0000e\u0000,\u0000 \u0000p\u0000l\u0000e\u0000a\u0000s\u0000e\u0000 \u0000a\u0000u\u0000t\u0000o\u0000g\u0000r\u0000o\u0000u\u0000p\u0000 \u0000o\u0000f\u0000f\u0000 \u0000i\u0000n\u0000 \u0000t\u0000h\u0000e\u0000 \u0000c\u0000u\u0000r\u0000v\u0000e\u0000 \u0000l\u0000i\u0000b\u0000r\u0000a\u0000r\u0000y\u0000.\u0000", "Ygòf¿~^/fê¨R\u0006RÄ~`O\rNïSåNûm R^\u0017R\u00020HQã>eê¨R\u0006RÄ~\u00020", "á¬ Á\u001cÁà¬\u0000¬ \u0000ÇÙ³ø­ù¸TÖÁÀÜÐtÇtº \u0000ü¬\u001cÈ,¸DÇ \u0000½ÀÇ`Õ\u0018ÂÆÅµÂÈ²ä².\u0000 \u0000ü¬\u001cÈ,¸DÇ \u0000½ÀÇXÕ$¸tº \u0000á¬ Á\u001cÁà¬XÇ \u0000ÇÙ³ø­ù¸TÖ|¹ \u0000tÕ\u001cÈXÕíÂÜÂ$Æ.\u0000"]] string[][] [["E\u0000n\u0000t\u0000e\u0000r\u0000 \u0000t\u0000h\u0000e\u0000 \u0000n\u0000a\u0000m\u0000e\u0000 \u0000o\u0000f\u0000 \u0000t\u0000h\u0000e\u0000 \u0000n\u0000e\u0000w\u0000 \u0000s\u0000t\u0000e\u0000p\u0000 \u0000y\u0000o\u0000u\u0000 \u0000w\u0000i\u0000s\u0000h\u0000 \u0000t\u0000o\u0000 \u0000a\u0000d\u0000d\u0000 \u0000t\u0000o\u0000 \u0000c\u0000a\u0000t\u0000e\u0000g\u0000o\u0000r\u0000y\u0000.\u0000M\u0000e\u0000s\u0000s\u0000a\u0000g\u0000e\u0000s\u0000:\u0000", "eQ°eek¤\rTW[`Oó`ûm RNáOo`:\u0000", "µÑô¼8»€½X¹ÐÅ \u0000”Í\u0000¬XÕ$¸”² \u0000ÈÀ\\¸´Æ \u0000ü¬\u001cÈmÕ©ºtÇ„¹DÇ \u0000…Ç%¸XÕÜÂ$Æ:\u0000"]] string[][] [["T\u0000h\u0000i\u0000s\u0000 \u0000u\u0000s\u0000e\u0000r\u0000 \u0000c\u0000a\u0000n\u0000'\u0000t\u0000 \u0000e\u0000d\u0000i\u0000t\u0000 \u0000o\u0000r\u0000 \u0000s\u0000e\u0000e\u0000 \u0000s\u0000t\u0000e\u0000p\u0000.\u0000", "Ù*N(u7b\rNïSåN\u0016\u0016b\u000bw\u0000Nek¤\u00020", "tÇ \u0000¬À©ÆÇ² \u0000ü¬\u001cÈmÕ©ºDÇ \u0000¸ÓÑÉXÕp¬° \u0000ü¼\u0018ÂÆÅµÂÈ²ä².\u0000"], ["T\u0000h\u0000i\u0000s\u0000 \u0000u\u0000s\u0000e\u0000r\u0000 \u0000c\u0000a\u0000n\u0000'\u0000t\u0000 \u0000s\u0000a\u0000v\u0000e\u0000.\u0000", "Ù*N(u7b\rNýÝOX[.\u0000", "tÇ \u0000¬À©ÆÇ² \u0000ô¼\u0000­`Õ\u0018Â \u0000ÆÅµÂÈ²ä².\u0000"]] string[][] [["V\u0000a\u0000l\u0000u\u0000e\u0000s\u0000 \u0000c\u0000a\u0000n\u0000n\u0000o\u0000t\u0000 \u0000c\u0000o\u0000n\u0000t\u0000a\u0000i\u0000n\u0000 \u0000m\u0000o\u0000r\u0000e\u0000 \u0000t\u0000h\u0000a\u0000n\u0000 \u0000o\u0000n\u0000e\u0000 \u0000d\u0000a\u0000t\u0000a\u0000 \u0000p\u0000o\u0000i\u0000n\u0000t\u0000.\u0000", "<P\rNý€\u0005S+T$N*NåN\nN„vpenc¹p.\u0000", "\u0012¬@Ç \u0000\\Õ\u001c¬ \u0000tÇÁÀXÇ \u0000ÇÌ¸\u0010ÈDÇ \u0000ìÓhÕ`Õ\u0018Â \u0000ÆÅµÂÈ²ä².\u0000"], ["C\u0000a\u0000n\u0000 \u0000n\u0000o\u0000t\u0000 \u0000a\u0000d\u0000d\u0000 \u0000w\u0000i\u0000n\u0000d\u0000o\u0000w\u0000.\u0000", "àeÕlûm R—zãS.\u0000", "=Ì8»DÇ \u0000½À…Ç`Õ\u0018Â \u0000ÆÅµÂÈ²ä².\u0000"], ["C\u0000a\u0000n\u0000 \u0000n\u0000o\u0000t\u0000 \u0000a\u0000d\u0000d\u0000 \u0000w\u0000i\u0000n\u0000d\u0000o\u0000w\u0000 \u0000b\u0000e\u0000c\u0000a\u0000u\u0000s\u0000e\u0000 \u0000b\u0000a\u0000c\u0000k\u0000g\u0000r\u0000o\u0000u\u0000n\u0000d\u0000 \u0000w\u0000i\u0000n\u0000d\u0000o\u0000w\u0000 \u0000i\u0000s\u0000 \u0000s\u0000m\u0000a\u0000l\u0000l\u0000.\u0000", "\rNý€žX R—zãSàV:NÌ€of—zˆ_\u000f\\\u00020", "0¼½¬=Ì8»XÇ \u0000lÐ0®\u0000¬ \u0000‘ÇDÅ\u001cÁ \u0000=Ì8»DÇ \u0000½À…Ç`Õ\u0018Â \u0000ÆÅµÂÈ²ä².\u0000"], ["C\u0000a\u0000n\u0000'\u0000t\u0000 \u0000i\u0000n\u0000s\u0000e\u0000r\u0000t\u0000 \u0000d\u0000a\u0000t\u0000a\u0000 \u0000v\u0000i\u0000e\u0000w\u0000 \u0000w\u0000i\u0000n\u0000d\u0000o\u0000w\u0000.\u0000", "àeÕlûm R—zãS.\u0000", "ÇÌ¸ô¼0®=Ì8»DÇ \u0000T³tÇÁÀ \u0000½ÀÇ`Õ\u0018Â \u0000ÆÅµÂÈ²ä².\u0000"], ["T\u0000h\u0000i\u0000s\u0000 \u0000d\u0000a\u0000t\u0000a\u0000 \u0000c\u0000a\u0000n\u0000 \u0000n\u0000o\u0000t\u0000 \u0000b\u0000e\u0000 \u0000c\u0000h\u0000a\u0000n\u0000g\u0000e\u0000d\u0000.\u0000", "Ù*Npenc\rNïSý«9eØS.\u0000", "tÇ \u0000ÇÌ¸² \u0000À¼½¬ ´\u0018ÂÆÅµÂÈ²ä².\u0000"]] string[][] [["W\u0000r\u0000o\u0000n\u0000g\u0000 \u0000d\u0000a\u0000t\u0000a\u0000 \u0000t\u0000y\u0000p\u0000e\u0000.\u0000", "dkHr,gV\u0000I\u0000„vpenc{|‹W\u0019•ï‹.\u0000", "ÇÌ¸\u0015ÖÝÂtÇ \u0000ÀÒ½¹È²ä².\u0000"], ["C\u0000a\u0000n\u0000'\u0000t\u0000 \u0000o\u0000p\u0000e\u0000n\u0000 \u0000d\u0000o\u0000c\u0000u\u0000m\u0000e\u0000n\u0000t\u0000.\u0000", "àeÕlSb\u0000_‡eöN.\u0000", "=Ì8»DÇ \u0000ôÅ\u0018ÂÆÅµÂÈ²ä².\u0000"]] string[][] [["W\u0000i\u0000n\u0000d\u0000o\u0000w\u0000s\u0000 \u0000a\u0000u\u0000d\u0000i\u0000o\u0000 \u0000d\u0000e\u0000v\u0000i\u0000c\u0000e\u0000 \u0000c\u0000a\u0000r\u0000d\u0000 \u0000d\u0000o\u0000 \u0000n\u0000o\u0000t\u0000 \u0000f\u0000o\u0000u\u0000n\u0000d\u0000 \u0000o\u0000n\u0000 \u0000t\u0000h\u0000e\u0000 \u0000s\u0000y\u0000s\u0000t\u0000e\u0000m\u0000.\u0000\n\u0000U\u0000p\u0000d\u0000a\u0000t\u0000e\u0000 \u0000y\u0000o\u0000u\u0000r\u0000 \u0000a\u0000u\u0000d\u0000i\u0000o\u0000 \u0000d\u0000e\u0000v\u0000i\u0000c\u0000e\u0000 \u0000i\u0000n\u0000 \u0000t\u0000h\u0000e\u0000 \u0000S\u0000o\u0000u\u0000n\u0000d\u0000C\u0000a\u0000r\u0000d\u0000 \u0000E\u0000d\u0000i\u0000t\u0000i\u0000o\u0000r\u0000.\u0000\n\u0000%\u0000s\u0000", "(WÙðS5u\u0011Ì¡l\tg~b0R\u0002\bTó¾\u0007YaS \u0000%\u0000s\u0000.\u0000\n\u0000÷(WlxöN\u0016hV-Nôf°eó¾\u0007Y.\u0000", "dÏèÔ0ÑÐÅ \u0000%\u0000s\u0000 \u0000LÇ1ÁtÎÜ´\u0000¬ \u0000ÆÅµÂÈ²ä².\u0000\n\u0000XÕÜ´èÆ´Å¸ÓÑÉ0®ÐÅ\u001cÁ \u0000LÇ1ÁtÎÜ´\u0015Èô¼|¹ \u00001¬àÂXÕíÂÜÂ$Æ.\u0000"], ["D\u0000o\u0000 \u0000y\u0000o\u0000u\u0000 \u0000d\u0000e\u0000l\u0000e\u0000t\u0000e\u0000 \u0000c\u0000h\u0000a\u0000n\u0000n\u0000e\u0000l\u0000 \u0000[\u0000%\u0000s\u0000]\u0000?\u0000", "`O Rd\u001aS \u0000%\u0000s\u0000 \u0000\u0017T?\u0000", "µÑ\\¸mÕ©º \u0000%\u0000s\u0000 \u0000DÇ \u0000­À\u001cÈXÕ ¬µÂÈ²L®?\u0000"], ["E\u0000q\u0000u\u0000a\u0000l\u0000 \u0000C\u0000h\u0000a\u0000n\u0000n\u0000e\u0000l\u0000 \u0000N\u0000a\u0000m\u0000e\u0000 \u0000e\u0000x\u0000i\u0000s\u0000t\u0000s\u0000.\u0000", "dk\u001aS\rTò]X[(W.\u0000", "\u0019¬@Ç \u0000µÑ\\¸tÇ„¹tÇ \u0000tÇø» \u0000tÈ¬ÇiÕÈ²ä².\u0000"], ["P\u0000l\u0000e\u0000a\u0000s\u0000e\u0000,\u0000 \u0000i\u0000n\u0000p\u0000u\u0000t\u0000 \u0000c\u0000h\u0000a\u0000n\u0000n\u0000e\u0000l\u0000 \u0000n\u0000a\u0000m\u0000e\u0000 \u0000c\u0000o\u0000r\u0000r\u0000e\u0000c\u0000t\u0000l\u0000y\u0000.\u0000", "÷eQcknxveQ\u001aS\rTW[.\u0000", "…Çl­µÑ\\¸tÇ„¹DÇ \u0000\u0015ÈUÖˆ× \u0000…Ç%¸XÕíÂÜÂ$Æ.\u0000"], ["W\u0000r\u0000o\u0000n\u0000g\u0000 \u0000d\u0000a\u0000t\u0000a\u0000 \u0000t\u0000y\u0000p\u0000e\u0000 \u0000n\u0000a\u0000m\u0000e\u0000 \u0000f\u0000o\u0000r\u0000 \u0000t\u0000h\u0000i\u0000s\u0000 \u0000c\u0000o\u0000n\u0000v\u0000e\u0000r\u0000s\u0000i\u0000o\u0000n\u0000 \u0000V\u0000I\u0000", "dkHr,gV\u0000I\u0000„vpenc{|‹W\u0019•ï‹.\u0000", "ÇÌ¸\u0015ÖÝÂtÇ \u0000ÀÒ½¹È²ä².\u0000"], ["S\u0000e\u0000l\u0000e\u0000c\u0000t\u0000 \u0000O\u0000u\u0000t\u0000p\u0000u\u0000t\u0000 \u0000C\u0000h\u0000a\u0000n\u0000n\u0000e\u0000l\u0000", "÷\týlúQ\u001aS.\u0000", "œÍl­µÑ\\¸|¹ \u0000 ÁÝÐXÕíÂÜÂ$Æ.\u0000"], ["S\u0000e\u0000l\u0000e\u0000c\u0000t\u0000 \u0000I\u0000n\u0000p\u0000u\u0000t\u0000 \u0000C\u0000h\u0000a\u0000n\u0000n\u0000e\u0000l\u0000", "÷\tébeQ\u001aS.\u0000", "…Çl­µÑ\\¸|¹ \u0000 ÁÝÐXÕíÂÜÂ$Æ.\u0000"], ["C\u0000a\u0000n\u0000 \u0000n\u0000o\u0000t\u0000 \u0000r\u0000e\u0000v\u0000e\u0000r\u0000t\u0000.\u0000", "àeÕlØS.\u0000", "ÐÆø¼ÇÌ¸|¹ \u0000}Ç´Å \u0000ä´|Ç\u0018Â \u0000ÆÅµÂÈ²ä².\u0000"], ["E\u0000q\u0000u\u0000a\u0000l\u0000 \u0000C\u0000h\u0000a\u0000n\u0000n\u0000e\u0000l\u0000 \u0000N\u0000a\u0000m\u0000e\u0000 \u0000e\u0000x\u0000i\u0000s\u0000t\u0000s\u0000.\u0000 \u0000E\u0000q\u0000u\u0000a\u0000l\u0000 \u0000C\u0000h\u0000a\u0000n\u0000n\u0000e\u0000l\u0000 \u0000N\u0000a\u0000m\u0000e\u0000 \u0000d\u0000e\u0000l\u0000e\u0000t\u0000e\u0000.\u0000", "dk\u001aS\rTò]X[(W.\u0000 \u0000\u001aS\rT Rd.\u0000", "\u0019¬@Ç \u0000µÑ\\¸tÇ„¹tÇ \u0000tÇø» \u0000tÈ¬ÇiÕÈ²ä².\u0000 \u0000\u0019¬@Ç \u0000µÑ\\¸tÇ„¹@Ç \u0000­À\u001cÈiÕÈ²ä².\u0000"], ["T\u0000h\u0000i\u0000s\u0000 \u0000w\u0000i\u0000l\u0000l\u0000 \u0000c\u0000l\u0000o\u0000s\u0000e\u0000 \u0000a\u0000l\u0000l\u0000 \u0000o\u0000p\u0000e\u0000r\u0000a\u0000t\u0000o\u0000r\u0000s\u0000.\u0000", "\u0006\\\u001aOsQí•@b\tg„vêNhˆ.\u0000", "Ù³‘Ç\u0011ÉxÇ \u0000\u0000¬ÁÀÄ¬0®|¹ \u0000¨ºP´ \u0000…ÈÌ¸iÕÈ²ä².\u0000"]] w39 string[][] [["W\u0000r\u0000o\u0000n\u0000g\u0000 \u0000d\u0000a\u0000t\u0000a\u0000 \u0000t\u0000y\u0000p\u0000e\u0000 \u0000n\u0000a\u0000m\u0000e\u0000 \u0000f\u0000o\u0000r\u0000 \u0000t\u0000h\u0000i\u0000s\u0000 \u0000c\u0000o\u0000n\u0000v\u0000e\u0000r\u0000s\u0000i\u0000o\u0000n\u0000 \u0000V\u0000I\u0000.\u0000", "dkHr,gV\u0000I\u0000„vpenc{|‹W\u0019•ï‹.\u0000", "ÇÌ¸\u0015ÖÝÂtÇ \u0000ÀÒ½¹È²ä².\u0000"], ["C\u0000a\u0000n\u0000 \u0000n\u0000o\u0000t\u0000 \u0000r\u0000e\u0000v\u0000e\u0000r\u0000t\u0000.\u0000", "àeÕlØS.\u0000", "ÐÆø¼ÇÌ¸|¹ \u0000}Ç´Å \u0000ä´|Ç\u0018Â \u0000ÆÅµÂÈ²ä².\u0000"], ["C\u0000a\u0000n\u0000 \u0000n\u0000o\u0000t\u0000 \u0000o\u0000p\u0000e\u0000n\u0000 \u0000C\u0000R\u0000Y\u00006\u00001\u00008\u00001\u0000 \u0000U\u0000S\u0000B\u0000 \u0000D\u0000e\u0000v\u0000i\u0000c\u0000e\u0000.\u0000", "\rNý€Sb\u0000_C\u0000R\u0000Y\u00006\u00001\u00008\u00001\u0000Åˆn.\u0000", "C\u0000R\u0000Y\u00006\u00001\u00008\u00001\u0000 \u0000¥ÇXÎ|¹ \u0000ôÅ\u0018Â \u0000ÆÅµÂÈ²ä².\u0000"], ["F\u0000a\u0000i\u0000l\u0000 \u0000t\u0000o\u0000 \u0000a\u0000p\u0000p\u0000l\u0000y\u0000 \u0000d\u0000e\u0000v\u0000i\u0000c\u0000e\u0000 \u0000s\u0000e\u0000t\u0000t\u0000i\u0000n\u0000g\u0000s\u0000.\u0000", "Ån¾n1Y%.\u0000", "¥ÇXÎ$Á\u0015ÈÐÅ \u0000äÂ(ÓXÕ\u0000ÆµÂÈ²ä².\u0000"]] string[][] [["E\u0000R\u0000R\u0000O\u0000R\u0000 \u0000o\u0000c\u0000c\u0000u\u0000r\u0000r\u0000e\u0000d\u0000 \u0000w\u0000h\u0000e\u0000n\u0000 \u0000w\u0000r\u0000i\u0000t\u0000i\u0000n\u0000g\u0000 \u0000o\u0000n\u0000e\u0000 \u0000o\u0000r\u0000 \u0000m\u0000o\u0000r\u0000e\u0000\n\u0000C\u0000a\u0000l\u0000i\u0000b\u0000r\u0000a\u0000t\u0000i\u0000o\u0000n\u0000 \u0000c\u0000u\u0000r\u0000v\u0000e\u0000s\u0000 \u0000t\u0000o\u0000 \u0000d\u0000i\u0000s\u0000k\u0000.\u0000 \u0000 \u0000T\u0000h\u0000e\u0000 \u0000C\u0000a\u0000l\u0000i\u0000b\u0000r\u0000a\u0000t\u0000i\u0000o\u0000n\u0000 \u0000y\u0000o\u0000u\u0000 \u0000h\u0000a\u0000v\u0000e\u0000\n\u0000s\u0000a\u0000v\u0000e\u0000d\u0000 \u0000m\u0000a\u0000y\u0000 \u0000n\u0000o\u0000t\u0000 \u0000f\u0000u\u0000n\u0000c\u0000t\u0000i\u0000o\u0000n\u0000 \u0000p\u0000r\u0000o\u0000p\u0000e\u0000r\u0000l\u0000y\u0000.\u0000", "S_Q\u0000N*N\u0016bôf\u001aY\n\u0000!hÆQòf¿~0RÁxØvöe\u0019ïÑS\u001fu.\u0000 \u0000`OÝOX[v!hÆQïSý\rNýck8^Ð\\O.\u0000\u0000\u0000", "\\Õ\u001c¬ \u0000\u0010¶”² \u0000ø­ \u0000tÇÁÀXÇ \u0000P­\u0000Éá¬ ÁDÇ \u0000ðÄ0®`ÕLµ \u0000$Æ Ç\u0000¬ \u0000\u001c¼ÝÀXÕ\u0000ÆµÂÈ²ä².\u0000 \u0000ù²àÂtÇ \u0000ô¼\u0000­\\Õ \u0000P­\u0000É@Ç \u0000\u0015ÈUÖˆ× \u0000Ù³‘ÇXÕÀÉ \u0000JÅDÇ\u0018Â \u0000 \u0000ˆÇµÂÈ²ä².\u0000"], ["N\u0000o\u0000 \u0000S\u0000i\u0000g\u0000n\u0000a\u0000l\u0000 \u0000D\u0000e\u0000t\u0000e\u0000c\u0000t\u0000e\u0000d\u0000!\u0000", "¡l\tgÀhKmáO÷S!\u0000", "àÂ8Ö\u0000¬ \u0000€¬!Î\u0018´ÀÉ \u0000JÅXÅµÂÈ²ä²!\u0000"], ["W\u0000r\u0000o\u0000n\u0000g\u0000 \u0000d\u0000a\u0000t\u0000a\u0000 \u0000t\u0000y\u0000p\u0000e\u0000 \u0000n\u0000a\u0000m\u0000e\u0000 \u0000f\u0000o\u0000r\u0000 \u0000t\u0000h\u0000i\u0000s\u0000 \u0000c\u0000o\u0000n\u0000v\u0000e\u0000r\u0000s\u0000i\u0000o\u0000n\u0000 \u0000V\u0000I\u0000.\u0000", "dkHr,gV\u0000I\u0000„vpenc{|‹W\u0019•ï‹.\u0000", "ÇÌ¸\u0015ÖÝÂtÇ \u0000ÀÒ½¹È²ä².\u0000"], ["C\u0000a\u0000n\u0000 \u0000n\u0000o\u0000t\u0000 \u0000r\u0000e\u0000v\u0000e\u0000r\u0000t\u0000.\u0000", "àeÕlØS.\u0000", "ÐÆø¼ÇÌ¸|¹ \u0000}Ç´Å \u0000ä´|Ç\u0018Â \u0000ÆÅµÂÈ²ä².\u0000"], ["A\u0000r\u0000e\u0000 \u0000y\u0000o\u0000u\u0000 \u0000s\u0000u\u0000r\u0000e\u0000 \u0000y\u0000o\u0000u\u0000 \u0000w\u0000a\u0000n\u0000t\u0000 \u0000t\u0000o\u0000 \u0000d\u0000e\u0000l\u0000e\u0000t\u0000e\u0000 \u0000[\u0000%\u0000s\u0000]\u0000?\u0000", "`O Rd \u0000%\u0000s\u0000 \u0000\u0017T?\u0000", "%\u0000s\u0000 \u0000DÇ \u0000­À\u001cÈXÕ ¬µÂÈ²L®?\u0000"], ["Y\u0000o\u0000u\u0000 \u0000c\u0000a\u0000n\u0000'\u0000t\u0000 \u0000s\u0000a\u0000v\u0000e\u0000.\u0000", "\rNý€ÝOX[.\u0000", "ô¼\u0000­`Õ\u0018Â \u0000ÆÅµÂÈ²ä².\u0000"], ["Y\u0000o\u0000u\u0000 \u0000c\u0000a\u0000n\u0000'\u0000t\u0000 \u0000d\u0000e\u0000l\u0000e\u0000t\u0000e\u0000.\u0000", "\rNý€ Rd–.\u0000", "­À\u001cÈ`Õ\u0018Â \u0000ÆÅµÂÈ²ä².\u0000"], ["Y\u0000o\u0000u\u0000 \u0000c\u0000a\u0000n\u0000'\u0000t\u0000 \u0000r\u0000e\u0000n\u0000a\u0000m\u0000e\u0000.\u0000", "\rNý€Í‘}T\rT.\u0000", "À¼½¬`Õ\u0018Â \u0000ÆÅµÂÈ²ä².\u0000"], ["T\u0000h\u0000i\u0000s\u0000 \u0000t\u0000y\u0000p\u0000e\u0000 \u0000n\u0000a\u0000m\u0000e\u0000 \u0000e\u0000x\u0000i\u0000s\u0000t\u0000s\u0000 \u0000a\u0000l\u0000r\u0000e\u0000a\u0000d\u0000y\u0000.\u0000", "ÙÍy{|W\rTðyò]Ï~X[(W", "tÇø» \u0000tÈ¬ÇiÕÈ²ä².\u0000"], ["I\u0000n\u0000p\u0000u\u0000t\u0000 \u0000S\u0000i\u0000g\u0000n\u0000a\u0000l\u0000 \u0000T\u0000y\u0000p\u0000e\u0000", "eQáO÷S{|W", "…Çl­àÂ8Ö\u0015ÖÜÐ|¹ \u0000 ÁÝÐXÕíÂÜÂ$Æ.\u0000"], ["O\u0000u\u0000t\u0000p\u0000u\u0000t\u0000 \u0000S\u0000i\u0000g\u0000n\u0000a\u0000l\u0000 \u0000T\u0000y\u0000p\u0000e\u0000", "úQáO÷S{|W", "œÍl­àÂ8Ö\u0015ÖÜÐ|¹ \u0000 ÁÝÐXÕíÂÜÂ$Æ.\u0000"], ["I\u0000m\u0000p\u0000o\u0000r\u0000t\u0000 \u0000C\u0000a\u0000l\u0000i\u0000b\u0000r\u0000a\u0000t\u0000i\u0000o\u0000n\u0000 \u0000D\u0000a\u0000t\u0000a\u0000", "!hÆQpencü[eQ", "á¬ ÁÇÌ¸õ¼¬À"], ["B\u0000e\u0000c\u0000a\u0000u\u0000s\u0000e\u0000 \u0000c\u0000u\u0000r\u0000v\u0000e\u0000 \u0000n\u0000a\u0000m\u0000e\u0000 \u0000d\u0000o\u0000n\u0000'\u0000t\u0000 \u0000e\u0000x\u0000i\u0000s\u0000t\u0000,\u0000 \u0000a\u0000f\u0000t\u0000e\u0000r\u0000 \u0000y\u0000o\u0000u\u0000 \u0000p\u0000r\u0000e\u0000s\u0000s\u0000 \u0000[\u0000A\u0000p\u0000p\u0000l\u0000y\u0000]\u0000 \u0000 \u0000i\u0000n\u0000 \u0000E\u0000d\u0000i\u0000t\u0000o\u0000r\u0000,\u0000 \u0000 \u0000p\u0000l\u0000e\u0000a\u0000s\u0000e\u0000,\u0000 \u0000p\u0000r\u0000e\u0000s\u0000s\u0000 \u0000[\u0000C\u0000o\u0000p\u0000y\u0000 \u0000F\u0000r\u0000o\u0000m\u0000 \u0000C\u0000u\u0000r\u0000v\u0000e\u0000 \u0000L\u0000i\u0000b\u0000r\u0000a\u0000r\u0000y\u0000]\u0000.\u0000", "àV:Nòf¿~\rTðy\rNX[(W,\u0000(\u0000^(u)\u0000°eû\u0016hV\u000eT,\u0000÷\rY6R.\u0000", "á¬ Á\u001cÁà¬tÇ„¹tÇ \u0000ÆÅ<ÇÀ»\\¸ \u0000¸ÓÑÉ0®ÐÅ\u001cÁ \u0000[\u0000\u0001È©Æ]\u0000DÇ \u0000\u0004²x¹ \u0000ÄÖ \u0000tÇ \u0000pÈ‘ÇtÇ \u0000\u0000¬¥²iÕÈ²ä².\u0000"], ["C\u0000a\u0000l\u0000i\u0000b\u0000r\u0000a\u0000t\u0000i\u0000o\u0000n\u0000 \u0000F\u0000i\u0000l\u0000e\u0000 \u0000[\u0000%\u0000s\u0000]\u0000 \u0000d\u0000o\u0000e\u0000s\u0000 \u0000n\u0000o\u0000t\u0000 \u0000e\u0000x\u0000i\u0000s\u0000t\u0000.\u0000", "!hÆQ‡eöN \u0000[\u0000%\u0000s\u0000]\u0000v^\rNX[(W\u00020", "[\u0000%\u0000s\u0000]\u0000 \u0000P­\u0000É\fÓ|ÇtÇ \u0000ÆÅµÂÈ²ä².\u0000"]] w42 string[][] [["W\u0000r\u0000o\u0000n\u0000g\u0000 \u0000d\u0000a\u0000t\u0000a\u0000 \u0000t\u0000y\u0000p\u0000e\u0000 \u0000n\u0000a\u0000m\u0000e\u0000 \u0000f\u0000o\u0000r\u0000 \u0000t\u0000h\u0000i\u0000s\u0000 \u0000c\u0000o\u0000n\u0000v\u0000e\u0000r\u0000s\u0000i\u0000o\u0000n\u0000 \u0000V\u0000I\u0000.\u0000", "dkHr,gV\u0000I\u0000„vpenc{|‹W\u0019•ï‹.\u0000", "ÇÌ¸\u0015ÖÝÂtÇ \u0000ÀÒ½¹È²ä².\u0000"], ["C\u0000a\u0000n\u0000'\u0000t\u0000 \u0000r\u0000e\u0000a\u0000d\u0000 \u0000h\u0000a\u0000r\u0000d\u0000w\u0000a\u0000r\u0000e\u0000 \u0000i\u0000n\u0000t\u0000e\u0000r\u0000f\u0000a\u0000c\u0000e\u0000 \u0000i\u0000n\u0000f\u0000o\u0000r\u0000m\u0000a\u0000t\u0000i\u0000o\u0000n\u0000.\u0000", "àeÕlû‹ÖSlxöN¥cãSáOo`.\u0000", "XÕÜ´èÆ´Å\u0000³tº$Á\u0015È\u0015Èô¼|¹ \u0000}ÇDÇ\u0018Â \u0000ÆÅµÂÈ²ä².\u0000"], ["C\u0000a\u0000n\u0000 \u0000n\u0000o\u0000t\u0000 \u0000r\u0000e\u0000v\u0000e\u0000r\u0000t\u0000.\u0000", "àeÕlØS.\u0000", "ÐÆø¼ÇÌ¸|¹ \u0000}Ç´Å \u0000ä´|Ç\u0018Â \u0000ÆÅµÂÈ²ä².\u0000"], ["C\u0000a\u0000n\u0000 \u0000n\u0000o\u0000t\u0000 \u0000i\u0000n\u0000i\u0000t\u0000 \u0000u\u0000s\u0000b\u0000 \u0000d\u0000e\u0000v\u0000i\u0000c\u0000e\u0000.\u0000", "\rNý€\u001dRËY\u0016SU\u0000S\u0000B\u0000¾‹\u0007Y\u00020", "U\u0000S\u0000B\u0000¥ÇXÎ|¹ \u0000\bÍ0®TÖ \u0000`Õ\u0018Â \u0000ÆÅµÂÈ²ä².\u0000"], ["C\u0000a\u0000n\u0000 \u0000n\u0000o\u0000t\u0000 \u0000s\u0000e\u0000t\u0000 \u0000D\u0000i\u0000g\u0000i\u0000t\u0000a\u0000l\u0000 \u0000I\u0000O\u0000 \u0000P\u0000o\u0000r\u0000t\u0000 \u00001\u0000.\u0000", "\rNý€¾‹npeW[I\u0000O\u0000ïzãS1\u0000\u00020", "D\u0000i\u0000g\u0000i\u0000t\u0000a\u0000l\u0000 \u0000I\u0000O\u0000 \u0000ìÓl­ \u00001\u0000 \u0000DÇ \u0000$Á\u0015È`Õ\u0018Â \u0000ÆÅµÂÈ²ä².\u0000"], ["C\u0000a\u0000n\u0000 \u0000n\u0000o\u0000t\u0000 \u0000s\u0000e\u0000t\u0000 \u0000D\u0000i\u0000g\u0000i\u0000t\u0000a\u0000l\u0000 \u0000I\u0000O\u0000 \u0000P\u0000o\u0000r\u0000t\u0000 \u00002\u0000.\u0000", "\rNý€¾‹npeW[I\u0000O\u0000ïzãS2\u0000\u00020", "D\u0000i\u0000g\u0000i\u0000t\u0000a\u0000l\u0000 \u0000I\u0000O\u0000 \u0000ìÓl­ \u00002\u0000 \u0000DÇ \u0000$Á\u0015È`Õ\u0018Â \u0000ÆÅµÂÈ²ä².\u0000"]] string[][] [["W\u0000r\u0000o\u0000n\u0000g\u0000 \u0000d\u0000a\u0000t\u0000a\u0000 \u0000t\u0000y\u0000p\u0000e\u0000 \u0000n\u0000a\u0000m\u0000e\u0000 \u0000f\u0000o\u0000r\u0000 \u0000t\u0000h\u0000i\u0000s\u0000 \u0000c\u0000o\u0000n\u0000v\u0000e\u0000r\u0000s\u0000i\u0000o\u0000n\u0000 \u0000V\u0000I\u0000", "dkHr,gV\u0000I\u0000„vpenc{|‹W\u0019•ï‹.\u0000", "ÇÌ¸\u0015ÖÝÂtÇ \u0000ÀÒ½¹È²ä².\u0000"], ["L\u0000o\u0000g\u0000 \u0000S\u0000w\u0000e\u0000e\u0000p\u0000 \u0000S\u0000t\u0000a\u0000r\u0000t\u0000 \u0000F\u0000r\u0000e\u0000q\u0000u\u0000e\u0000n\u0000c\u0000y\u0000 \u0000m\u0000u\u0000s\u0000t\u0000 \u0000b\u0000e\u0000 \u0000l\u0000e\u0000s\u0000s\u0000 \u0000t\u0000h\u0000a\u0000n\u0000 \u0000t\u0000h\u0000e\u0000 \u0000S\u0000t\u0000o\u0000p\u0000 \u0000F\u0000r\u0000e\u0000q\u0000u\u0000e\u0000n\u0000c\u0000y\u0000.\u0000", "ù[pekbÏc\u0000_ËY‘˜‡sÅ_{˜\u000f\\ŽN\\Pbk‘˜‡s.\u0000", "üÈ\fÓ\u0018Â\\¸ø­üÈ¬ÀXÇ \u0000ÜÂ‘ÇüÈ\fÓ\u0018Â”² \u0000\u0015ÈÀÉüÈ\fÓ\u0018Âô¼ä² \u0000‘ÇDÅ|Å \u0000iÕÈ²ä².\u0000"], ["C\u0000a\u0000l\u0000c\u0000u\u0000l\u0000a\u0000t\u0000i\u0000n\u0000g\u0000.\u0000.\u0000.\u0000", "¡‹—{.\u0000.\u0000.\u0000", "Ä¬°À\u0011É.\u0000.\u0000"], ["W\u0000A\u0000R\u0000N\u0000I\u0000N\u0000G\u0000!\u0000 \u0000S\u0000e\u0000l\u0000e\u0000c\u0000t\u0000e\u0000d\u0000 \u0000l\u0000o\u0000w\u0000e\u0000r\u0000 \u0000f\u0000r\u0000e\u0000q\u0000u\u0000e\u0000n\u0000c\u0000y\u0000 \u0000i\u0000s\u0000 \u0000o\u0000u\u0000t\u0000s\u0000i\u0000d\u0000e\u0000 \u0000p\u0000r\u0000e\u0000s\u0000e\u0000n\u0000t\u0000 \u0000C\u0000a\u0000l\u0000i\u0000b\u0000r\u0000a\u0000t\u0000i\u0000o\u0000n\u0000 \u0000r\u0000a\u0000n\u0000g\u0000e\u0000.\u0000 \u0000P\u0000l\u0000e\u0000a\u0000s\u0000e\u0000 \u0000s\u0000e\u0000l\u0000e\u0000c\u0000t\u0000 \u0000a\u0000 \u0000 \u0000f\u0000r\u0000e\u0000q\u0000u\u0000e\u0000n\u0000c\u0000y\u0000 \u0000g\u0000r\u0000e\u0000a\u0000t\u0000h\u0000e\u0000r\u0000 \u0000t\u0000h\u0000a\u0000n\u0000 \u0000o\u0000r\u0000 \u0000e\u0000q\u0000u\u0000a\u0000l\u0000 \u0000t\u0000o\u0000 \u0000%\u0000.\u00002\u0000f\u0000 \u0000H\u0000z\u0000", "fJT!\u0000\tébNOvs/fîvMR!hck\u0003ôV\u0016Y.\u0000 \u0000\tébvs\u0000g\u0011\\'YN\u0016bI{N \u0000%\u0000.\u00002\u0000f\u0000 \u0000H\u0000z\u0000.\u0000", "½¬à¬!\u0000 \u0000 ÁÝÐ\u001c´ \u0000DÅ˜· \u0000üÈ\fÓ\u0018Â”² \u0000P­\u0000É”¼\u0004Ç\u0016¼ÐÅ \u0000ˆÇµÂÈ²ä².\u0000 \u0000%\u0000.\u00002\u0000f\u0000 \u0000H\u0000z\u0000@Æ \u0000\u0019¬p¬˜° \u0000ø­ô¼ä² \u0000pÐ \u0000üÈ\fÓ\u0018Â|¹ \u0000 ÁÝÐXÕíÂÜÂ$Æ.\u0000"], ["W\u0000A\u0000R\u0000N\u0000I\u0000N\u0000G\u0000!\u0000 \u0000S\u0000e\u0000l\u0000e\u0000c\u0000t\u0000e\u0000d\u0000 \u0000u\u0000p\u0000p\u0000e\u0000r\u0000 \u0000f\u0000r\u0000e\u0000q\u0000u\u0000e\u0000n\u0000c\u0000y\u0000 \u0000i\u0000s\u0000 \u0000o\u0000u\u0000t\u0000s\u0000i\u0000d\u0000e\u0000 \u0000p\u0000r\u0000e\u0000s\u0000e\u0000n\u0000t\u0000 \u0000C\u0000a\u0000l\u0000i\u0000b\u0000r\u0000a\u0000t\u0000i\u0000o\u0000n\u0000 \u0000r\u0000a\u0000n\u0000g\u0000e\u0000.\u0000 \u0000P\u0000l\u0000e\u0000a\u0000s\u0000e\u0000 \u0000s\u0000e\u0000l\u0000e\u0000c\u0000t\u0000 \u0000a\u0000 \u0000 \u0000f\u0000r\u0000e\u0000q\u0000u\u0000e\u0000n\u0000c\u0000y\u0000 \u0000l\u0000e\u0000s\u0000s\u0000 \u0000t\u0000h\u0000a\u0000n\u0000 \u0000o\u0000r\u0000 \u0000e\u0000q\u0000u\u0000a\u0000l\u0000 \u0000t\u0000o\u0000 \u0000%\u0000.\u00002\u0000f\u0000 \u0000H\u0000z\u0000", "fJT!\u0000\tébv\nNPs/fîvMR!hÆQ\u0003ôVKN\u0016Y.\u0000 \u0000\tébvs\u0000g\u0011\\'YN\u0016bI{N \u0000%\u0000.\u00002\u0000f\u0000 \u0000H\u0000z\u0000.\u0000", "½¬à¬!\u0000 \u0000 ÁÝÐ\u001c´ \u0000ÃÆ \u0000üÈ\fÓ\u0018Â”² \u0000P­\u0000É”¼\u0004Ç\u0016¼ÐÅ \u0000ˆÇµÂÈ²ä².\u0000 \u0000%\u0000.\u00002\u0000f\u0000 \u0000H\u0000z\u0000@Æ \u0000\u0019¬p¬˜° \u0000ø­ô¼ä² \u0000‘Ç@Ç \u0000üÈ\fÓ\u0018Â|¹ \u0000 ÁÝÐXÕíÂÜÂ$Æ.\u0000"], ["W\u0000A\u0000R\u0000N\u0000I\u0000N\u0000G\u0000!\u0000 \u0000S\u0000e\u0000l\u0000e\u0000c\u0000t\u0000e\u0000d\u0000 \u0000l\u0000o\u0000w\u0000e\u0000r\u0000 \u0000f\u0000r\u0000e\u0000q\u0000u\u0000e\u0000n\u0000c\u0000y\u0000 \u0000i\u0000s\u0000 \u0000o\u0000u\u0000t\u0000s\u0000i\u0000d\u0000e\u0000 \u0000p\u0000r\u0000e\u0000s\u0000e\u0000n\u0000t\u0000 \u0000M\u0000o\u0000u\u0000t\u0000h\u0000 \u0000C\u0000a\u0000l\u0000i\u0000b\u0000r\u0000a\u0000t\u0000i\u0000o\u0000n\u0000 \u0000r\u0000a\u0000n\u0000g\u0000e\u0000.\u0000 \u0000P\u0000l\u0000e\u0000a\u0000s\u0000e\u0000 \u0000s\u0000e\u0000l\u0000e\u0000c\u0000t\u0000 \u0000a\u0000 \u0000 \u0000f\u0000r\u0000e\u0000q\u0000u\u0000e\u0000n\u0000c\u0000y\u0000 \u0000g\u0000r\u0000e\u0000a\u0000t\u0000h\u0000e\u0000r\u0000 \u0000t\u0000h\u0000a\u0000n\u0000 \u0000o\u0000r\u0000 \u0000e\u0000q\u0000u\u0000a\u0000l\u0000 \u0000t\u0000o\u0000:\u0000%\u0000.\u00002\u0000f\u0000 \u0000H\u0000z\u0000", "fJT!\u0000\tébNOvs/fîvMR!hck\u0003ôV\u0016Y.\u0000 \u0000\tébvs\u0000g\u0011\\'YN\u0016bI{N \u0000%\u0000.\u00002\u0000f\u0000 \u0000H\u0000z\u0000.\u0000", "½¬à¬!\u0000 \u0000 ÁÝÐ\u001c´ \u0000DÅ˜· \u0000üÈ\fÓ\u0018Â”² \u0000…ÇP­\u0000É”¼\u0004ÇXÇ \u0000\u0016¼ÐÅ \u0000ˆÇµÂÈ²ä².\u0000 \u0000%\u0000.\u00002\u0000f\u0000 \u0000H\u0000z\u0000@Æ \u0000\u0019¬p¬˜° \u0000ø­ô¼ä² \u0000pÐ \u0000üÈ\fÓ\u0018Â|¹ \u0000 ÁÝÐXÕíÂÜÂ$Æ.\u0000"], ["W\u0000A\u0000R\u0000N\u0000I\u0000N\u0000G\u0000!\u0000 \u0000S\u0000e\u0000l\u0000e\u0000c\u0000t\u0000e\u0000d\u0000 \u0000u\u0000p\u0000p\u0000e\u0000r\u0000 \u0000f\u0000r\u0000e\u0000q\u0000u\u0000e\u0000n\u0000c\u0000y\u0000 \u0000i\u0000s\u0000 \u0000o\u0000u\u0000t\u0000s\u0000i\u0000d\u0000e\u0000 \u0000p\u0000r\u0000e\u0000s\u0000e\u0000n\u0000t\u0000 \u0000M\u0000o\u0000u\u0000t\u0000h\u0000 \u0000C\u0000a\u0000l\u0000i\u0000b\u0000r\u0000a\u0000t\u0000i\u0000o\u0000n\u0000 \u0000r\u0000a\u0000n\u0000g\u0000e\u0000.\u0000 \u0000P\u0000l\u0000e\u0000a\u0000s\u0000e\u0000 \u0000s\u0000e\u0000l\u0000e\u0000c\u0000t\u0000 \u0000a\u0000 \u0000 \u0000f\u0000r\u0000e\u0000q\u0000u\u0000e\u0000n\u0000c\u0000y\u0000 \u0000l\u0000e\u0000s\u0000s\u0000 \u0000t\u0000h\u0000a\u0000n\u0000 \u0000o\u0000r\u0000 \u0000e\u0000q\u0000u\u0000a\u0000l\u0000 \u0000t\u0000o\u0000:\u0000%\u0000.\u00002\u0000f\u0000 \u0000H\u0000z\u0000", "fJT!\u0000\tébv\nNPs/fîvMR!hÆQ\u0003ôVKN\u0016Y.\u0000 \u0000\tébvs\u0000g\u0011\\'YN\u0016bI{N \u0000%\u0000.\u00002\u0000f\u0000 \u0000H\u0000z\u0000.\u0000", "½¬à¬!\u0000 \u0000 ÁÝÐ\u001c´ \u0000ÃÆ \u0000üÈ\fÓ\u0018Â”² \u0000…ÇP­\u0000É”¼\u0004ÇXÇ \u0000\u0016¼ÐÅ \u0000ˆÇµÂÈ²ä².\u0000 \u0000%\u0000.\u00002\u0000f\u0000 \u0000H\u0000z\u0000@Æ \u0000\u0019¬p¬˜° \u0000ø­ô¼ä² \u0000‘Ç@Ç \u0000üÈ\fÓ\u0018Â|¹ \u0000 ÁÝÐXÕíÂÜÂ$Æ.\u0000"], ["W\u0000A\u0000R\u0000N\u0000I\u0000N\u0000G\u0000!\u0000 \u0000S\u0000e\u0000l\u0000e\u0000c\u0000t\u0000e\u0000d\u0000 \u0000S\u0000t\u0000e\u0000p\u0000 \u0000S\u0000i\u0000z\u0000e\u0000 \u0000i\u0000s\u0000 \u0000i\u0000n\u0000c\u0000o\u0000m\u0000p\u0000a\u0000t\u0000i\u0000b\u0000l\u0000e\u0000 \u0000w\u0000i\u0000t\u0000h\u0000 \u0000p\u0000r\u0000e\u0000s\u0000e\u0000n\u0000t\u0000 \u0000C\u0000a\u0000l\u0000i\u0000b\u0000r\u0000a\u0000t\u0000i\u0000o\u0000n\u0000 \u0000S\u0000t\u0000e\u0000p\u0000 \u0000S\u0000i\u0000z\u0000e\u0000.\u0000 \u0000T\u0000h\u0000e\u0000 \u0000E\u0000q\u0000u\u0000a\u0000l\u0000i\u0000z\u0000a\u0000t\u0000i\u0000o\u0000n\u0000 \u0000c\u0000u\u0000r\u0000v\u0000e\u0000 \u0000h\u0000a\u0000s\u0000 \u0000b\u0000e\u0000e\u0000n\u0000 \u0000i\u0000n\u0000t\u0000e\u0000r\u0000p\u0000o\u0000l\u0000a\u0000t\u0000e\u0000d\u0000.\u0000", "fJT!\u0000\t[vek/f\rN&{\bTîvMRv!hÆQek.\u0000 \u0000GWaòf¿~ò]Ï~Òc.\u0000", "½¬à¬!\u0000 \u0000 ÁÝÐ\u001c´ \u0000x¬LÇlÐ0®”² \u0000\u0004Ö¬Ç \u0000P­\u0000Éx¬LÇlÐ0®@Æ \u0000¨º\u001cÂ)´È²ä².\u0000 \u0000\u0015ÈÜ­á¬ Á@Ç \u0000ô¼\u0004¬\u0018´\u0000ÆµÂÈ²ä².\u0000"], ["E\u0000R\u0000R\u0000O\u0000R\u0000 \u0000s\u0000e\u0000t\u0000t\u0000i\u0000n\u0000g\u0000 \u0000D\u0000C\u0000 \u0000v\u0000o\u0000l\u0000t\u0000a\u0000g\u0000e\u0000 \u0000o\u0000u\u0000t\u0000 \u0000t\u0000h\u0000r\u0000o\u0000u\u0000g\u0000h\u0000 \u0000C\u0000O\u0000M\u0000 \u0000%\u0000d\u0000", "\u0019•ï‹¾‹nôvAm5u‹S0RC\u0000O\u0000M\u0000 \u0000%\u0000d\u0000.\u0000", "ìÓl­ \u0000%\u0000d\u0000|¹ \u0000µÑtÕ\u001cÁ \u0000˜°\u0000¬”² \u0000ÁÉX¹\u0004ÈUÅ$Á\u0015ÈtÇ \u0000˜Ç»º\u0018´\u0000ÆµÂÈ²ä².\u0000"], ["T\u0000h\u0000e\u0000 \u0000s\u0000t\u0000i\u0000m\u0000u\u0000l\u0000u\u0000s\u0000 \u0000t\u0000o\u0000 \u0000b\u0000e\u0000 \u0000p\u0000l\u0000a\u0000y\u0000e\u0000d\u0000 \u0000h\u0000a\u0000s\u0000 \u0000a\u0000n\u0000 \u0000a\u0000m\u0000p\u0000l\u0000i\u0000t\u0000u\u0000d\u0000e\u0000 \u0000g\u0000r\u0000e\u0000a\u0000t\u0000e\u0000r\u0000 \u0000t\u0000h\u0000a\u0000n\u0000 \u0000t\u0000h\u0000e\u0000 \u0000r\u0000a\u0000n\u0000g\u0000e\u0000 \u0000o\u0000f\u0000 \u0000t\u0000h\u0000e\u0000 \u0000s\u0000e\u0000l\u0000e\u0000c\u0000t\u0000e\u0000d\u0000 \u0000h\u0000a\u0000r\u0000d\u0000w\u0000a\u0000r\u0000e\u0000.\u0000\n\u0000P\u0000l\u0000e\u0000a\u0000s\u0000e\u0000 \u0000c\u0000h\u0000e\u0000c\u0000k\u0000 \u0000H\u0000a\u0000r\u0000d\u0000w\u0000a\u0000r\u0000e\u0000 \u0000s\u0000e\u0000t\u0000u\u0000p\u0000,\u0000 \u0000C\u0000a\u0000l\u0000i\u0000b\u0000r\u0000a\u0000t\u0000i\u0000o\u0000n\u0000 \u0000S\u0000e\u0000n\u0000s\u0000i\u0000t\u0000i\u0000v\u0000i\u0000t\u0000y\u0000 \u0000v\u0000a\u0000l\u0000u\u0000e\u0000s\u0000 \u0000a\u0000n\u0000d\u0000 \u0000S\u0000t\u0000i\u0000m\u0000u\u0000l\u0000u\u0000s\u0000 \u0000P\u0000a\u0000r\u0000a\u0000m\u0000e\u0000t\u0000e\u0000r\u0000s\u0000.\u0000", "­d>evÀo±RvE^¦^'YN\t[vlxöN\u0003ôV.\u0000\n\u0000÷ÀhåglxöN¾n,\u0000 \u0000!hÆQupOe¦^<PTÀo±RÂSpe.\u0000", "¬ÇÝÀ\u0018´² \u0000Çù­àÂ8Ö² \u0000 ÁÝÐ\u001c´ \u0000¥ÇXÎXÇ \u0000¼\u0004Çô¼ä² \u0000pÐ \u0000ÄÉíÓDÇ \u0000\u0000¬ÀÉà¬ÇµÂÈ²ä².\u0000\n\u0000XÕÜ´èÆ´Å$Á\u0015È,\u0000 \u0000P­\u0000É$Á\u0015È,\u0000 \u0000Çù­àÂ8Ö\fÓ|·Tº0Ñä´DÇ \u0000UÖxÇXÕíÂÜÂ$Æ.\u0000"], ["C\u0000a\u0000n\u0000 \u0000n\u0000o\u0000t\u0000 \u0000r\u0000e\u0000v\u0000e\u0000r\u0000t\u0000.\u0000", "àeÕlØS.\u0000", "ÐÆø¼ÇÌ¸|¹ \u0000}Ç´Å \u0000ä´|Ç\u0018Â \u0000ÆÅµÂÈ²ä².\u0000"]] _ string[][] [["W\u0000r\u0000o\u0000n\u0000g\u0000 \u0000d\u0000a\u0000t\u0000a\u0000 \u0000t\u0000y\u0000p\u0000e\u0000 \u0000n\u0000a\u0000m\u0000e\u0000 \u0000f\u0000o\u0000r\u0000 \u0000t\u0000h\u0000i\u0000s\u0000 \u0000c\u0000o\u0000n\u0000v\u0000e\u0000r\u0000s\u0000i\u0000o\u0000n\u0000 \u0000V\u0000I\u0000", "dkHr,gV\u0000I\u0000„vpenc{|‹W\u0019•ï‹.\u0000", "ÇÌ¸\u0015ÖÝÂtÇ \u0000ÀÒ½¹È²ä².\u0000"], ["D\u0000u\u0000p\u0000l\u0000i\u0000c\u0000a\u0000t\u0000e\u0000 \u0000c\u0000h\u0000a\u0000n\u0000n\u0000e\u0000l\u0000s\u0000 \u0000a\u0000r\u0000e\u0000 \u0000n\u0000o\u0000t\u0000 \u0000a\u0000l\u0000l\u0000o\u0000w\u0000e\u0000d\u0000 \u0000i\u0000n\u0000 \u0000a\u0000 \u0000s\u0000i\u0000n\u0000g\u0000l\u0000e\u0000 \u0000a\u0000c\u0000q\u0000u\u0000i\u0000s\u0000i\u0000t\u0000i\u0000o\u0000n\u0000 \u0000s\u0000t\u0000e\u0000p\u0000.\u0000", "\rNAQ¸(W\u0000N*NUS\u0000NvÇÆek¤\u000b \u000b /fÍ\rYv\u001aS.\u0000", "\u0011Éõ¼\u001c´ \u0000µÑ\\¸ä´@Ç \u0000è²\u001cÂDÌÑÉ)¼ÝÂÐÅ\u001cÁ \u0000ÈÕ©Æ\u0018´ÀÉ \u0000JÅµÂÈ²ä².\u0000"], ["A\u0000l\u0000l\u0000 \u0000i\u0000n\u0000p\u0000u\u0000t\u0000 \u0000c\u0000h\u0000a\u0000n\u0000n\u0000e\u0000l\u0000s\u0000 \u0000m\u0000u\u0000s\u0000t\u0000 \u0000h\u0000a\u0000v\u0000e\u0000 \u0000t\u0000h\u0000e\u0000 \u0000s\u0000a\u0000m\u0000e\u0000 \u0000b\u0000i\u0000t\u0000 \u0000d\u0000e\u0000p\u0000t\u0000h\u0000 \u0000a\u0000n\u0000d\u0000 \u0000a\u0000l\u0000l\u0000 \u0000o\u0000u\u0000t\u0000p\u0000u\u0000t\u0000 \u0000c\u0000h\u0000a\u0000n\u0000n\u0000e\u0000l\u0000s\u0000 \u0000m\u0000u\u0000s\u0000t\u0000 \u0000h\u0000a\u0000v\u0000e\u0000 \u0000t\u0000h\u0000e\u0000 \u0000s\u0000a\u0000m\u0000e\u0000 \u0000b\u0000i\u0000t\u0000 \u0000d\u0000e\u0000p\u0000t\u0000h\u0000.\u0000", "@b\tgeQ\u001aSÅ_{\tgøv\fTvMOñm¦^T@b\tgúQ\u001aSÅ_{\tgøv\fTvMOñm¦^.\u0000", "¨ºà´ \u0000Çl­µÑ\\¸ä´@Ç \u0000\u0019¬@Ç \u0000É·ÇTÖD¾¸Ò\u0018Â|¹ \u0000\u0000¬8È|Å \u0000XÕpº \u0000¨ºà´ \u0000Íl­µÑ\\¸ä´@Ç \u0000\u0019¬@Ç \u0000É·ÇTÖD¾¸Ò\u0018Â|¹ \u0000\u0000¬8È|Å \u0000iÕÈ²ä².\u0000"], ["T\u0000h\u0000e\u0000 \u0000s\u0000t\u0000i\u0000m\u0000u\u0000l\u0000u\u0000s\u0000 \u0000h\u0000a\u0000s\u0000 \u0000a\u0000 \u0000d\u0000i\u0000f\u0000f\u0000e\u0000r\u0000e\u0000n\u0000t\u0000 \u0000s\u0000a\u0000m\u0000p\u0000l\u0000i\u0000n\u0000g\u0000 \u0000r\u0000a\u0000t\u0000e\u0000 \u0000t\u0000h\u0000a\u0000n\u0000 \u0000t\u0000h\u0000e\u0000 \u0000o\u0000u\u0000t\u0000p\u0000u\u0000t\u0000 \u0000c\u0000h\u0000a\u0000n\u0000n\u0000e\u0000l\u0000 \u0000s\u0000e\u0000l\u0000e\u0000c\u0000t\u0000e\u0000d\u0000 \u0000i\u0000n\u0000 \u0000A\u0000c\u0000q\u0000u\u0000i\u0000s\u0000i\u0000t\u0000i\u0000o\u0000n\u0000 \u0000E\u0000d\u0000i\u0000t\u0000o\u0000r\u0000.\u0000 \u0000 \u0000T\u0000h\u0000i\u0000s\u0000 \u0000i\u0000s\u0000 \u0000n\u0000o\u0000t\u0000 \u0000a\u0000 \u0000s\u0000u\u0000p\u0000p\u0000o\u0000r\u0000t\u0000e\u0000d\u0000 \u0000s\u0000e\u0000t\u0000u\u0000p\u0000.\u0000", "Ào±R\tg\rN\fTvÇ7hsÔk(WÇÆ\u0016hV-N\tébúQ\u001aS\n\u0000Ù\rN/f\u0000N*N×S/e\u0001cv[Å.\u0000", "Çù­àÂ8Ö² \u0000àÂ8ÖDÌÑÉ0®ÐÅ\u001cÁ \u0000 ÁÝÐ\u001c´ \u0000Íl­µÑ\\¸@Æ \u0000ä²x¹ \u0000\\Ôø¼TÖüÈ\fÓ\u0018Â|¹ \u0000\u0000¬ÀÉà¬ \u0000ÇµÂÈ²ä².\u0000\n\u0000tÇ¬@Ç \u0000\u001cÈõ¬\u0018´ÀÉ \u0000JÅ² \u0000$Á\u0015ÈÇÈ²ä².\u0000"], ["S\u0000t\u0000i\u0000m\u0000u\u0000l\u0000u\u0000s\u0000 \u0000d\u0000a\u0000t\u0000a\u0000 \u0000d\u0000o\u0000e\u0000s\u0000 \u0000n\u0000o\u0000t\u0000 \u0000e\u0000x\u0000i\u0000s\u0000t\u0000.\u0000", "Ào±Rpenc\rNX[(W.\u0000", "Çù­àÂ8ÖÇÌ¸\u0000¬ \u0000tÈ¬ÇXÕÀÉ \u0000JÅµÂÈ²ä².\u0000"], ["T\u0000h\u0000i\u0000s\u0000 \u0000A\u0000q\u0000u\u0000i\u0000s\u0000i\u0000t\u0000i\u0000o\u0000n\u0000 \u0000S\u0000t\u0000e\u0000p\u0000 \u0000i\u0000s\u0000 \u0000n\u0000o\u0000t\u0000 \u0000S\u0000u\u0000p\u0000p\u0000o\u0000r\u0000t\u0000e\u0000d\u0000.\u0000 \u0000D\u0000u\u0000p\u0000l\u0000i\u0000c\u0000a\u0000t\u0000e\u0000 \u0000C\u0000h\u0000a\u0000n\u0000n\u0000e\u0000l\u0000s\u0000 \u0000a\u0000r\u0000e\u0000 \u0000n\u0000o\u0000t\u0000 \u0000a\u0000l\u0000l\u0000o\u0000w\u0000e\u0000d\u0000 \u0000i\u0000n\u0000 \u0000a\u0000 \u0000s\u0000i\u0000n\u0000g\u0000l\u0000e\u0000 \u0000A\u0000q\u0000u\u0000i\u0000s\u0000i\u0000t\u0000i\u0000o\u0000n\u0000 \u0000S\u0000t\u0000e\u0000p\u0000.\u0000", "ÙÇÆek¤/f\rN«/e\u0001cv.\u0000 \u0000\rNAQ¸(W\u0000N*NUS\u0000NvÇÆek¤/fÍ\rYv\u001aS.\u0000", "tÇ \u0000àÂ8ÖDÌÑÉ@Ç \u0000\u001cÈõ¬\u0018´ÀÉ \u0000JÅµÂÈ²ä².\u0000 \u0000 \u0000\u0011Éõ¼\u001c´ \u0000µÑ\\¸ä´@Ç \u0000è²\u001cÂDÌÑÉ)¼ÝÂÐÅ\u001cÁ \u0000ÈÕ©Æ\u0018´ÀÉ \u0000JÅµÂÈ²ä².\u0000"], ["P\u0000a\u0000d\u0000d\u0000i\u0000n\u0000g\u0000 \u0000T\u0000i\u0000m\u0000e\u0000 \u0000o\u0000r\u0000 \u0000R\u0000e\u0000c\u0000o\u0000r\u0000d\u0000 \u0000T\u0000i\u0000m\u0000e\u0000 \u0000R\u0000a\u0000n\u0000g\u0000e\u0000 \u0000E\u0000r\u0000r\u0000o\u0000r\u0000!\u0000\n\u0000P\u0000a\u0000d\u0000d\u0000i\u0000n\u0000g\u0000(\u00005\u00000\u0000m\u0000s\u0000~\u00002\u0000s\u0000)\u0000,\u0000 \u0000R\u0000e\u0000c\u0000o\u0000r\u0000d\u0000 \u0000T\u0000i\u0000m\u0000e\u0000(\u00005\u00000\u0000m\u0000s\u0000~\u00001\u00000\u0000s\u0000)\u0000", "kXEQöeô•\u0016b°‹U_öeô•\u0003ƒôV\u0019•ï‹!\u0000\n\u0000kXEQ(\u00005\u00000\u0000ëkÒy-\u00002\u0000Òy)\u0000,\u0000 \u0000°‹U_öeô•(\u00005\u00000\u0000ëkÒy-\u00001\u00000\u0000Òy)\u0000\n\u0000", "(Ó)µÜÂ\u0004¬ \u00009Ö@Ç \u00000®]¸ÜÂ\u0004¬ \u0000”¼\u0004Ç$Æ Ç!\u0000 \u0000(Ó)µ(\u00005\u00000\u0000m\u0000s\u0000~\u00002\u0000s\u0000)\u0000,\u0000 \u00000®]¸ÜÂ\u0004¬(\u00005\u00000\u0000m\u0000s\u0000~\u00001\u00000\u0000s\u0000)\u0000"], ["P\u0000l\u0000e\u0000a\u0000s\u0000e\u0000,\u0000 \u0000i\u0000n\u0000p\u0000u\u0000t\u0000 \u0000c\u0000u\u0000r\u0000v\u0000e\u0000 \u0000n\u0000a\u0000m\u0000e\u0000.\u0000", "÷eQòf¿~\rTðy.\u0000", "á¬ ÁtÇ„¹DÇ \u0000…Ç%¸XÕíÂÜÂ$Æ.\u0000"], ["C\u0000a\u0000n\u0000 \u0000n\u0000o\u0000t\u0000 \u0000r\u0000e\u0000v\u0000e\u0000r\u0000t\u0000.\u0000", "àeÕlØS.\u0000", "ÐÆø¼ÇÌ¸|¹ \u0000}Ç´Å \u0000ä´|Ç\u0018Â \u0000ÆÅµÂÈ²ä².\u0000"], ["C\u0000a\u0000n\u0000 \u0000n\u0000o\u0000t\u0000 \u0000o\u0000p\u0000e\u0000n\u0000 \u00002\u0000 \u0000A\u0000S\u0000I\u0000O\u0000 \u0000d\u0000r\u0000i\u0000v\u0000e\u0000r\u0000s\u0000.\u0000", "\rNSb\u0000_2\u0000*NA\u0000S\u0000I\u0000O\u0000q¨R\u000bz^.\u0000", "2\u0000\u001c¬XÇ \u0000A\u0000S\u0000I\u0000O\u0000Ü´|·tÇ„¼|¹ \u0000ôÅ\u0018Â \u0000ÆÅµÂÈ²ä².\u0000"], ["A\u0000c\u0000q\u0000u\u0000i\u0000s\u0000i\u0000t\u0000i\u0000o\u0000n\u0000 \u0000c\u0000h\u0000a\u0000n\u0000n\u0000e\u0000l\u0000 \u0000d\u0000o\u0000e\u0000s\u0000 \u0000n\u0000o\u0000t\u0000 \u0000e\u0000x\u0000i\u0000s\u0000t\u0000.\u0000", "ÇÆ\u001aS¡l\tg.\u0000", "àÂ8ÖDÌÑÉ \u0000µÑ\\¸\u0000¬ \u0000tÈ¬ÇXÕÀÉ \u0000JÅµÂÈ²ä².\u0000"]] string[][] [["W\u0000r\u0000o\u0000n\u0000g\u0000 \u0000d\u0000a\u0000t\u0000a\u0000 \u0000t\u0000y\u0000p\u0000e\u0000 \u0000n\u0000a\u0000m\u0000e\u0000 \u0000f\u0000o\u0000r\u0000 \u0000t\u0000h\u0000i\u0000s\u0000 \u0000c\u0000o\u0000n\u0000v\u0000e\u0000r\u0000s\u0000i\u0000o\u0000n\u0000 \u0000V\u0000I\u0000", "dkHr,gV\u0000I\u0000„vpenc{|‹W\u0019•ï‹.\u0000", "ÇÌ¸\u0015ÖÝÂtÇ \u0000ÀÒ½¹È²ä².\u0000"], ["C\u0000u\u0000r\u0000r\u0000e\u0000n\u0000t\u0000 \u0000s\u0000e\u0000t\u0000t\u0000i\u0000n\u0000g\u0000 \u0000w\u0000e\u0000r\u0000e\u0000 \u0000n\u0000o\u0000t\u0000 \u0000a\u0000p\u0000p\u0000l\u0000i\u0000e\u0000d\u0000.\u0000", "S_MR¾n\rN\u0002(u.\u0000", "\u0004Ö¬Ç \u0000$Á\u0015È@Ç \u0000\u0001È©Æ ´\u0018Â \u0000ÆÅµÂÈ²ä².\u0000"], ["Y\u0000o\u0000u\u0000 \u0000m\u0000a\u0000y\u0000 \u0000n\u0000e\u0000e\u0000d\u0000 \u0000a\u0000 \u0000F\u0000r\u0000e\u0000q\u0000u\u0000e\u0000n\u0000c\u0000y\u0000 \u0000L\u0000o\u0000g\u0000 \u0000S\u0000w\u0000e\u0000e\u0000p\u0000 \u0000i\u0000n\u0000 \u0000y\u0000o\u0000u\u0000r\u0000 \u0000S\u0000t\u0000i\u0000m\u0000u\u0000l\u0000u\u0000s\u0000 \u0000s\u0000t\u0000e\u0000p\u0000 \u0000t\u0000o\u0000 \u0000r\u0000u\u0000n\u0000 \u0000y\u0000o\u0000u\u0000r\u0000 \u0000s\u0000e\u0000q\u0000u\u0000e\u0000n\u0000c\u0000e\u0000 \u0000w\u0000i\u0000t\u0000h\u0000 \u0000t\u0000h\u0000e\u0000 \u0000T\u0000i\u0000m\u0000e\u0000 \u0000S\u0000e\u0000l\u0000e\u0000c\u0000t\u0000i\u0000v\u0000e\u0000 \u0000R\u0000e\u0000s\u0000p\u0000o\u0000n\u0000s\u0000e\u0000 \u0000a\u0000l\u0000g\u0000o\u0000r\u0000i\u0000t\u0000h\u0000m\u0000.\u0000", "¨`ïSý\u0000(W¨`vÏ~NmÀo±Rekvsù[pekbÏc,\u0000ÐLöeô\téb'`^\u0017R.\u0000", "ÜÂ\u0004¬ ÁÝÐQÇõ²LÅà¬¬¹ì´DÇ \u0000\u0000¬ÀÉà¬ \u0000\u0004Ö¬Ç \u0000ü¬\u001cÈ,¸DÇ \u0000äÂ‰ÕXÕ$¸tº \u0000üÈ\fÓ\u0018Â\\¸ø­üÈ¬À|¹ \u0000¬À©ÆXÕíÂÜÂ$Æ.\u0000"], ["E\u0000d\u0000i\u0000t\u0000 \u0000H\u0000a\u0000r\u0000m\u0000o\u0000n\u0000i\u0000c\u0000 \u0000L\u0000i\u0000s\u0000t\u0000.\u0000", "\u0016\u0010âl\rT.\u0000", "pÈTÖ\fÓ©º]¸DÇ \u0000¸ÓÑÉXÕíÂÜÂ$Æ.\u0000"], ["Y\u0000o\u0000u\u0000 \u0000m\u0000u\u0000s\u0000t\u0000 \u0000a\u0000d\u0000d\u0000 \u0000H\u0000a\u0000r\u0000m\u0000o\u0000n\u0000i\u0000c\u0000s\u0000 \u0000o\u0000v\u0000e\u0000r\u0000 \u0000t\u0000h\u0000e\u0000 \u00009\u0000t\u0000h\u0000 \u0000t\u0000o\u0000 \u0000g\u0000e\u0000t\u0000 \u0000a\u0000 \u0000r\u0000e\u0000l\u0000i\u0000a\u0000b\u0000l\u0000e\u0000 \u0000R\u0000u\u0000b\u0000 \u0000&\u0000 \u0000B\u0000u\u0000z\u0000z\u0000 \u0000m\u0000e\u0000a\u0000s\u0000u\u0000r\u0000e\u0000m\u0000e\u0000n\u0000t\u0000.\u0000", "¨`Å_{˜ûm R(W9\u0000t\u0000h\u0000„v\u0010Œâl—_0RïS`—„v \u0000R\u0000u\u0000b\u0000 \u0000&\u0000 \u0000B\u0000u\u0000z\u0000z\u0000 \u0000KmÏ‘.\u0000", "R\u0000u\u0000b\u0000 \u0000&\u0000 \u0000B\u0000u\u0000z\u0000z\u0000 \u0000!Î\u0015ÈDÇ \u0000\u0015ÈUÖˆ× \u0000XÕ0® \u0000\u0004ÇXÕìÅ \u00009\u0000(ÌtÇÁÀXÇ \u0000pÈTÖ\fÓ|¹ \u0000 ÁÝÐXÕìÅ|Å \u0000iÕÈ²ä².\u0000"], ["C\u0000a\u0000n\u0000 \u0000n\u0000o\u0000t\u0000 \u0000r\u0000e\u0000v\u0000e\u0000r\u0000t\u0000.\u0000", "àeÕlØS.\u0000", "ÐÆø¼ÇÌ¸|¹ \u0000}Ç´Å \u0000ä´|Ç\u0018Â \u0000ÆÅµÂÈ²ä².\u0000"], ["T\u0000h\u0000e\u0000 \u0000f\u0000i\u0000r\u0000s\u0000t\u0000 \u0000n\u0000u\u0000m\u0000b\u0000e\u0000r\u0000 \u0000i\u0000n\u0000 \u0000t\u0000h\u0000e\u0000 \u0000r\u0000a\u0000n\u0000g\u0000e\u0000 \u0000m\u0000u\u0000s\u0000t\u0000 \u0000b\u0000e\u0000 \u0000l\u0000e\u0000s\u0000s\u0000 \u0000t\u0000h\u0000a\u0000n\u0000 \u0000t\u0000h\u0000e\u0000 \u0000s\u0000e\u0000c\u0000o\u0000n\u0000d\u0000 \u0000n\u0000u\u0000m\u0000b\u0000e\u0000r\u0000.\u0000", "\u0003ƒôV-N„v,{\u0000N*NpeW[Å_{˜\u000f\\ŽN,{ŒN*NpeW[.\u0000", ",¸XÇ \u0000«Ìˆ¼øÉˆ¼8Ö”² \u0000P´ˆ¼øÉˆ¼8Öô¼ä² \u0000‘ÇDÅ|Å \u0000iÕÈ²ä².\u0000"], ["H\u0000a\u0000r\u0000m\u0000o\u0000n\u0000i\u0000c\u0000 \u0000l\u0000i\u0000s\u0000t\u0000 \u0000i\u0000t\u0000e\u0000m\u0000 \u0000\"\u0000%\u0000s\u0000\"\u0000 \u0000i\u0000s\u0000 \u0000a\u0000l\u0000r\u0000e\u0000a\u0000d\u0000y\u0000 \u0000o\u0000n\u0000 \u0000t\u0000h\u0000e\u0000 \u0000l\u0000i\u0000s\u0000t\u0000.\u0000", "\u0010Œâl\u0017Rhˆy˜ \u0000\"\u0000%\u0000s\u0000\"\u0000/fò](W\rTUS\nN.\u0000", "XÕ¨ºÉ²©º]¸[\u0000%\u0000s\u0000]\u0000@Ç \u0000©º]¸ÐÅ \u0000tÇø» \u0000tÈ¬ÇiÕÈ²ä².\u0000"], ["T\u0000h\u0000e\u0000 \u0000w\u0000a\u0000v\u0000e\u0000f\u0000o\u0000r\u0000m\u0000s\u0000 \u0000%\u0000s\u0000 \u0000a\u0000n\u0000d\u0000 \u0000%\u0000s\u0000 \u0000d\u0000o\u0000n\u0000'\u0000t\u0000 \u0000h\u0000a\u0000v\u0000e\u0000 \u0000t\u0000h\u0000e\u0000 \u0000s\u0000a\u0000m\u0000e\u0000 \u0000s\u0000a\u0000m\u0000p\u0000l\u0000i\u0000n\u0000g\u0000 \u0000r\u0000a\u0000t\u0000e\u0000.\u0000\n\u0000T\u0000h\u0000e\u0000y\u0000 \u0000c\u0000a\u0000n\u0000n\u0000o\u0000t\u0000 \u0000b\u0000e\u0000 \u0000p\u0000r\u0000o\u0000c\u0000e\u0000s\u0000s\u0000e\u0000d\u0000 \u0000t\u0000o\u0000g\u0000e\u0000t\u0000h\u0000e\u0000r\u0000.\u0000", "âlb_ \u0000%\u0000s\u0000 \u0000T \u0000%\u0000s\u0000 \u0000\rNwQ\tgøv\fTvÇ7hs.\u0000\n\u0000ÖNìN\rNý\u0000Nw\u0004Y\u0006t.\u0000", "XÕ¨ºÉ²ÜÂ\u0004¬\fÓ\u0015Ö \u0000%\u0000s\u0000ü¬ \u0000%\u0000s\u0000@Ç \u0000\\Ôø¼TÖüÈ\fÓ\u0018Â\u0000¬ \u0000ä²…¹È²ä².\u0000\n\u0000tÇ \u0000\fÓ\u0015Öä´@Ç \u0000\u001cÁ\\¸ \u0000ðÅ°À`Õ\u0018Â \u0000ÆÅµÂÈ²ä².\u0000"]] _ _ string[][] [["T\u0000h\u0000e\u0000 \u0000A\u0000l\u0000i\u0000g\u0000n\u0000m\u0000e\u0000n\u0000t\u0000 \u0000r\u0000e\u0000f\u0000e\u0000r\u0000e\u0000n\u0000c\u0000e\u0000 \u0000p\u0000o\u0000i\u0000n\u0000t\u0000 \u0000i\u0000s\u0000 \u0000n\u0000o\u0000t\u0000 \u0000b\u0000e\u0000t\u0000w\u0000e\u0000e\u0000n\u0000 \u0000y\u0000o\u0000u\u0000r\u0000 \u0000l\u0000i\u0000m\u0000i\u0000t\u0000 \u0000c\u0000u\u0000r\u0000v\u0000e\u0000s\u0000.\u0000W\u0000o\u0000u\u0000l\u0000d\u0000 \u0000y\u0000o\u0000u\u0000 \u0000l\u0000i\u0000k\u0000e\u0000 \u0000t\u0000o\u0000 \u0000c\u0000o\u0000n\u0000t\u0000i\u0000n\u0000u\u0000e\u0000?\u0000", "-NÃ_!hÆQÂS\u0003¹p\rN/f`OvgPòf¿~KNôv.\u0000`Oó`ç~í~\u0017T?\u0000", "\u0011ÉìÂP­\u0015È8Ìà¬\u0010ÈtÇ \u0000\u001cÈ\\Õá¬ Á¬ÀtÇÐÅ \u0000ÇÀÉ \u0000JÅµÂÈ²ä².\u0000 \u0000Ä¬ÁXÕ ¬µÂÈ²L®?\u0000"], ["D\u0000o\u0000n\u0000'\u0000t\u0000 \u0000a\u0000p\u0000p\u0000l\u0000y\u0000,\u0000i\u0000f\u0000 \u0000t\u0000h\u0000e\u0000 \u0000d\u0000a\u0000t\u0000a\u0000 \u0000t\u0000y\u0000p\u0000e\u0000s\u0000 \u0000o\u0000f\u0000 \u0000u\u0000p\u0000p\u0000e\u0000r\u0000 \u0000l\u0000i\u0000m\u0000i\u0000t\u0000\n\u0000a\u0000n\u0000d\u0000 \u0000l\u0000o\u0000w\u0000e\u0000r\u0000 \u0000l\u0000i\u0000m\u0000i\u0000t\u0000 \u0000a\u0000r\u0000e\u0000 \u0000w\u0000a\u0000v\u0000e\u0000f\u0000o\u0000r\u0000m\u0000 \u0000!\u0000", "\rN^(u,\u0000Yg\nN\u000bNPpenc{|Wý/fâlb_!\u0000\u0000\u0000", "Ì¹|Ç \u0000DÅ˜·°Æ \u0000\u001cÈ\\Õá¬ ÁtÇ \u0000¨ºP´ \u0000ÜÂ\u0004¬\fÓ\u0015ÖtÇtº \u0000Ä¬°ÀXÕÀÉ \u0000È¹íÂÜÂ$Æ!\u0000"], ["T\u0000h\u0000e\u0000 \u0000L\u0000i\u0000m\u0000i\u0000t\u0000s\u0000 \u0000c\u0000u\u0000r\u0000v\u0000e\u0000(\u0000s\u0000)\u0000,\u0000v\u0000a\u0000l\u0000u\u0000e\u0000(\u0000s\u0000)\u0000 \u0000a\u0000n\u0000d\u0000/\u0000o\u0000r\u0000 \u0000t\u0000h\u0000e\u0000 \u0000m\u0000e\u0000a\u0000s\u0000u\u0000r\u0000e\u0000m\u0000e\u0000n\u0000t\u0000 \u0000c\u0000u\u0000r\u0000v\u0000e\u0000 \u0000h\u0000a\u0000v\u0000e\u0000 \u0000u\u0000n\u0000i\u0000t\u0000s\u0000 \u0000t\u0000h\u0000a\u0000t\u0000 \u0000d\u0000o\u0000n\u0000'\u0000t\u0000 \u0000m\u0000a\u0000t\u0000c\u0000h\u0000.\u0000R\u0000e\u0000s\u0000u\u0000l\u0000t\u0000s\u0000 \u0000m\u0000a\u0000y\u0000 \u0000b\u0000e\u0000 \u0000u\u0000n\u0000p\u0000r\u0000e\u0000d\u0000i\u0000c\u0000t\u0000a\u0000b\u0000l\u0000e\u0000 \u0000a\u0000n\u0000d\u0000 \u0000u\u0000n\u0000r\u0000e\u0000l\u0000i\u0000a\u0000b\u0000l\u0000e\u0000.\u0000", "gPòf¿~\u00010÷N<PT/\u0000\u0016b\tgUSMOvKmÏòf¿~\rN9SM.\u0000Ó~gïSý/f\rNïSåwvT\rNïS`v.\u0000", "\u001cÈ\\Õá¬ Á,\u0000è²\u001cÂ\u0012¬,\u0000!Î\u0015Èá¬ ÁXÇ \u0000è²\u0004Ç\u0000¬ \u0000Þ¹ÀÉ \u0000JÅDÅ\u001cÁ \u0000°¬ü¬”² \u0000\bÆ!Î`Õ\u0018Â \u0000ÆÅp¬˜° \u0000ÿ»DÇ\u0018Â \u0000ÆÅµÂÈ²ä².\u0000"], ["T\u0000h\u0000e\u0000 \u0000U\u0000p\u0000p\u0000e\u0000r\u0000 \u0000L\u0000i\u0000m\u0000i\u0000t\u0000 \u0000i\u0000s\u0000 \u0000l\u0000o\u0000w\u0000e\u0000r\u0000 \u0000t\u0000h\u0000a\u0000n\u0000 \u0000t\u0000h\u0000e\u0000 \u0000L\u0000o\u0000w\u0000e\u0000r\u0000 \u0000L\u0000i\u0000m\u0000i\u0000t\u0000.\u0000\n\u0000D\u0000o\u0000 \u0000y\u0000o\u0000u\u0000 \u0000w\u0000a\u0000n\u0000t\u0000 \u0000t\u0000o\u0000 \u0000c\u0000o\u0000n\u0000t\u0000i\u0000n\u0000u\u0000e\u0000?\u0000", "\nNPNON\u000bNP.\u0000\n\u0000`Oó`ç~í~\u0017T?\u0000\u0000\u0000", "ÁÀ\\ÕtÇ \u0000XÕ\\Õô¼ä² \u0000ÇµÂÈ²ä².\u0000 \u0000Ä¬ÁXÕ ¬µÂÈ²L®?\u0000"], ["A\u0000t\u0000 \u0000l\u0000e\u0000a\u0000s\u0000t\u0000 \u0000p\u0000a\u0000r\u0000t\u0000 \u0000o\u0000f\u0000 \u0000t\u0000h\u0000e\u0000 \u0000U\u0000p\u0000p\u0000e\u0000r\u0000 \u0000L\u0000i\u0000m\u0000i\u0000t\u0000 \u0000i\u0000s\u0000 \u0000l\u0000o\u0000w\u0000e\u0000r\u0000 \u0000t\u0000h\u0000a\u0000n\u0000 \u0000t\u0000h\u0000e\u0000 \u0000L\u0000o\u0000w\u0000e\u0000r\u0000 \u0000L\u0000i\u0000m\u0000i\u0000t\u0000.\u0000\n\u0000D\u0000o\u0000 \u0000y\u0000o\u0000u\u0000 \u0000w\u0000a\u0000n\u0000t\u0000 \u0000t\u0000o\u0000 \u0000c\u0000o\u0000n\u0000t\u0000i\u0000n\u0000u\u0000e\u0000?\u0000", "X[(W\u0000N¹p\u0016b\u001aY¹p\nNPNON\u000bNP.\u0000\n\u0000`Oó`ç~í~\u0017T?\u0000\u0000\u0000", "ÁÀ\\ÕXÇ \u0000\\Õ \u0000½½tÇ \u0000\u0001È´ÅÄ³ \u0000XÕ\\Õô¼ä² \u0000ÇµÂÈ²ä².\u0000 \u0000Ä¬ÁXÕ ¬µÂÈ²L®?\u0000"], ["W\u0000r\u0000o\u0000n\u0000g\u0000 \u0000d\u0000a\u0000t\u0000a\u0000 \u0000t\u0000y\u0000p\u0000e\u0000 \u0000n\u0000a\u0000m\u0000e\u0000 \u0000f\u0000o\u0000r\u0000 \u0000t\u0000h\u0000i\u0000s\u0000 \u0000c\u0000o\u0000n\u0000v\u0000e\u0000r\u0000s\u0000i\u0000o\u0000n\u0000 \u0000V\u0000I\u0000.\u0000", "dkHr,gV\u0000I\u0000„vpenc{|‹W\u0019•ï‹.\u0000", "ÇÌ¸\u0015ÖÝÂtÇ \u0000ÀÒ½¹È²ä².\u0000"], ["C\u0000a\u0000n\u0000 \u0000n\u0000o\u0000t\u0000 \u0000r\u0000e\u0000v\u0000e\u0000r\u0000t\u0000.\u0000", "àeÕlØS.\u0000", "ÐÆø¼ÇÌ¸|¹ \u0000}Ç´Å \u0000ä´|Ç\u0018Â \u0000ÆÅµÂÈ²ä².\u0000"], ["F\u0000l\u0000o\u0000a\u0000t\u0000i\u0000n\u0000g\u0000", "nm¨R", "X¹Ù³"]] _ string[][] [["W\u0000r\u0000o\u0000n\u0000g\u0000 \u0000d\u0000a\u0000t\u0000a\u0000 \u0000t\u0000y\u0000p\u0000e\u0000 \u0000n\u0000a\u0000m\u0000e\u0000 \u0000f\u0000o\u0000r\u0000 \u0000t\u0000h\u0000i\u0000s\u0000 \u0000c\u0000o\u0000n\u0000v\u0000e\u0000r\u0000s\u0000i\u0000o\u0000n\u0000 \u0000V\u0000I\u0000.\u0000", "dkHr,gV\u0000I\u0000„vpenc{|‹W\u0019•ï‹.\u0000", "ÇÌ¸\u0015ÖÝÂtÇ \u0000ÀÒ½¹È²ä².\u0000"]] string[][] [["W\u0000r\u0000o\u0000n\u0000g\u0000 \u0000d\u0000a\u0000t\u0000a\u0000 \u0000t\u0000y\u0000p\u0000e\u0000 \u0000n\u0000a\u0000m\u0000e\u0000 \u0000f\u0000o\u0000r\u0000 \u0000t\u0000h\u0000i\u0000s\u0000 \u0000c\u0000o\u0000n\u0000v\u0000e\u0000r\u0000s\u0000i\u0000o\u0000n\u0000 \u0000V\u0000I\u0000.\u0000", "dkHr,gV\u0000I\u0000„vpenc{|‹W\u0019•ï‹.\u0000", "ÇÌ¸\u0015ÖÝÂtÇ \u0000ÀÒ½¹È²ä².\u0000"], ["C\u0000a\u0000n\u0000 \u0000n\u0000o\u0000t\u0000 \u0000r\u0000e\u0000v\u0000e\u0000r\u0000t\u0000.\u0000", "àeÕlØS.\u0000", "ÐÆø¼ÇÌ¸|¹ \u0000}Ç´Å \u0000ä´|Ç\u0018Â \u0000ÆÅµÂÈ²ä².\u0000"]] _ _ _ string[][] [["Y\u0000o\u0000u\u0000 \u0000m\u0000u\u0000s\u0000t\u0000 \u0000f\u0000i\u0000r\u0000s\u0000t\u0000 \u0000s\u0000e\u0000l\u0000e\u0000c\u0000t\u0000 \u0000a\u0000n\u0000 \u0000i\u0000t\u0000e\u0000m\u0000.\u0000", "¨`Å_{HQ\téb\u0000N*Nyîv.\u0000", "mÕ©ºDÇ \u0000<º\u0000È \u0000 ÁÝÐXÕíÂÜÂ$Æ.\u0000"], ["T\u0000h\u0000e\u0000 \u0000f\u0000i\u0000l\u0000e\u0000 \u0000i\u0000s\u0000 \u0000c\u0000o\u0000r\u0000r\u0000u\u0000p\u0000t\u0000e\u0000d\u0000.\u0000 \u0000 \u0000D\u0000o\u0000 \u0000y\u0000o\u0000u\u0000 \u0000w\u0000i\u0000s\u0000h\u0000 \u0000t\u0000o\u0000\n\u0000c\u0000o\u0000n\u0000t\u0000i\u0000n\u0000u\u0000e\u0000 \u0000a\u0000n\u0000d\u0000 \u0000t\u0000r\u0000y\u0000 \u0000t\u0000o\u0000 \u0000e\u0000x\u0000t\u0000r\u0000a\u0000c\u0000t\u0000 \u0000d\u0000a\u0000t\u0000a\u0000 \u0000f\u0000r\u0000o\u0000m\u0000 \u0000i\u0000t\u0000\n\u0000(\u0000m\u0000a\u0000y\u0000 \u0000t\u0000a\u0000k\u0000e\u0000 \u0000s\u0000e\u0000v\u0000e\u0000r\u0000a\u0000l\u0000 \u0000s\u0000e\u0000c\u0000o\u0000n\u0000d\u0000s\u0000)\u0000?\u0000", "åeöNò]_cOW.\u0000 \u0000`Oó`ç~í~,\u0000v^ÕþVÐcÖSpenc(\u0000ïSý±9àQÒy)\u0000?\u0000\u0000\u0000", "tÇ \u0000\fÓ|Ç@Ç \u0000ÁÁÀ\u0018´\u0000ÆµÂÈ²ä².\u0000 \u0000\fÓ|Ç\\¸½0Ñ \u0000ÇÌ¸|¹ \u0000ÍÍXÕ ¬µÂÈ²L®?\u0000(\u0000ÜÂ\u0004¬tÇ \u0000x¬´¹\u0018Â \u0000ÇµÂÈ²ä².\u0000)\u0000"], ["T\u0000h\u0000e\u0000 \u0000f\u0000i\u0000l\u0000e\u0000 \u0000i\u0000s\u0000 \u0000c\u0000o\u0000r\u0000r\u0000u\u0000p\u0000t\u0000e\u0000d\u0000.\u0000 \u0000 \u0000D\u0000o\u0000 \u0000y\u0000o\u0000u\u0000 \u0000w\u0000i\u0000s\u0000h\u0000 \u0000t\u0000o\u0000\n\u0000c\u0000o\u0000n\u0000t\u0000i\u0000n\u0000u\u0000e\u0000 \u0000a\u0000n\u0000d\u0000 \u0000t\u0000r\u0000y\u0000 \u0000t\u0000o\u0000 \u0000e\u0000x\u0000t\u0000r\u0000a\u0000c\u0000t\u0000 \u0000r\u0000e\u0000s\u0000u\u0000l\u0000t\u0000s\u0000 \u0000f\u0000r\u0000o\u0000m\u0000 \u0000i\u0000t\u0000\n\u0000(\u0000m\u0000a\u0000y\u0000 \u0000t\u0000a\u0000k\u0000e\u0000 \u0000s\u0000e\u0000v\u0000e\u0000r\u0000a\u0000l\u0000 \u0000s\u0000e\u0000c\u0000o\u0000n\u0000d\u0000s\u0000)\u0000?\u0000", "åeöNò]_cOW.\u0000 \u0000`Oó`\n\u0000ç~í~,\u0000v^ÕþVÐcÖSÓ~g\n\u0000(\u0000ïSý±9àQÒy)\u0000?\u0000", "tÇ \u0000\fÓ|Ç@Ç \u0000ÁÁÀ\u0018´\u0000ÆµÂÈ²ä².\u0000 \u0000\fÓ|Ç\\¸½0Ñ \u0000°¬ü¬|¹ \u0000ÍÍXÕ ¬µÂÈ²L®?\u0000(\u0000ÜÂ\u0004¬tÇ \u0000x¬´¹\u0018Â \u0000ÇµÂÈ²ä².\u0000)\u0000"], ["T\u0000h\u0000e\u0000 \u0000f\u0000o\u0000l\u0000l\u0000o\u0000w\u0000i\u0000n\u0000g\u0000 \u0000i\u0000t\u0000e\u0000m\u0000 \u0000n\u0000u\u0000m\u0000b\u0000e\u0000r\u0000s\u0000 \u0000a\u0000r\u0000e\u0000 \u0000c\u0000o\u0000r\u0000r\u0000u\u0000p\u0000t\u0000 \u0000i\u0000n\u0000 \u0000t\u0000h\u0000e\u0000 \u0000f\u0000i\u0000l\u0000e\u0000 \u0000a\u0000n\u0000d\u0000 \u0000a\u0000r\u0000e\u0000 \u0000n\u0000o\u0000t\u0000 \u0000b\u0000e\u0000i\u0000n\u0000g\u0000 \u0000r\u0000e\u0000a\u0000d\u0000:\u0000", "\u000bN\u0017Ryîv\u0016÷S*al\f\rN«ûeöN:\u0000", "DÅ· \u0000mÕ©º¼8Ö\u0000¬ \u0000ÁÁÀ\u0018´ìÅ \u0000\fÓ|ÇDÇ \u0000}ÇDÇ\u0018Â \u0000ÆÅµÂÈ²ä²:\u0000"], ["T\u0000h\u0000i\u0000s\u0000 \u0000r\u0000e\u0000c\u0000a\u0000l\u0000l\u0000 \u0000f\u0000i\u0000l\u0000e\u0000 \u0000d\u0000o\u0000e\u0000s\u0000 \u0000n\u0000o\u0000t\u0000 \u0000e\u0000x\u0000i\u0000s\u0000t\u0000:\u0000", "Ù*NÞV>eeöN\rNX[(W:\u0000", "tÇ \u0000¬Ç8ÖœÍ\fÓ|Ç@Ç \u0000tÈ¬ÇXÕÀÉ \u0000JÅµÂÈ²ä²:\u0000"], ["P\u0000l\u0000e\u0000a\u0000s\u0000e\u0000 \u0000c\u0000h\u0000e\u0000c\u0000k\u0000 \u0000t\u0000h\u0000e\u0000 \u0000s\u0000p\u0000e\u0000l\u0000l\u0000i\u0000n\u0000g\u0000 \u0000o\u0000r\u0000 \u0000l\u0000o\u0000c\u0000a\u0000t\u0000i\u0000o\u0000n\u0000 \u0000o\u0000f\u0000 \u0000t\u0000h\u0000i\u0000s\u0000 \u0000f\u0000i\u0000l\u0000e\u0000(\u0000s\u0000)\u0000.\u0000", "÷ÀhågÙ*NeöNvübQTMOn.\u0000", "\fÓ|ÇXÇ \u0000\u0004ÇXÎ@Æ \u0000 ÌÇ|¹ \u0000¬¬ÀXÕíÂÜÂ$Æ.\u0000"], ["P\u0000l\u0000e\u0000a\u0000s\u0000e\u0000 \u0000e\u0000n\u0000t\u0000e\u0000r\u0000 \u0000a\u0000 \u0000n\u0000a\u0000m\u0000e\u0000 \u0000f\u0000o\u0000r\u0000 \u0000t\u0000h\u0000e\u0000 \u0000c\u0000u\u0000r\u0000v\u0000e\u0000 \u0000t\u0000o\u0000 \u0000b\u0000e\u0000 \u0000r\u0000e\u0000c\u0000a\u0000l\u0000l\u0000e\u0000d\u0000 \u0000:\u0000", "÷eQ\u0000N*N\rTðyvòf¿~«ìSÞV:\u0000", "¬Ç8ÖœÍ`Õ \u0000á¬ ÁtÇ„¹DÇ \u0000…Ç%¸XÕíÂÜÂ$Æ:\u0000"], ["W\u0000r\u0000o\u0000n\u0000g\u0000 \u0000d\u0000a\u0000t\u0000a\u0000 \u0000t\u0000y\u0000p\u0000e\u0000 \u0000n\u0000a\u0000m\u0000e\u0000 \u0000f\u0000o\u0000r\u0000 \u0000t\u0000h\u0000i\u0000s\u0000 \u0000c\u0000o\u0000n\u0000v\u0000e\u0000r\u0000s\u0000i\u0000o\u0000n\u0000 \u0000V\u0000I\u0000.\u0000", "dkHr,gV\u0000I\u0000„vpenc{|‹W\u0019•ï‹.\u0000", "ÇÌ¸\u0015ÖÝÂtÇ \u0000ÀÒ½¹È²ä².\u0000"], ["C\u0000a\u0000n\u0000 \u0000n\u0000o\u0000t\u0000 \u0000r\u0000e\u0000v\u0000e\u0000r\u0000t\u0000.\u0000", "àeÕlØS.\u0000", "ÐÆø¼ÇÌ¸|¹ \u0000}Ç´Å \u0000ä´|Ç\u0018Â \u0000ÆÅµÂÈ²ä².\u0000"], ["T\u0000h\u0000e\u0000 \u0000f\u0000i\u0000l\u0000e\u0000 \u0000i\u0000s\u0000 \u0000c\u0000o\u0000r\u0000r\u0000u\u0000p\u0000t\u0000e\u0000d\u0000.\u0000 \u0000 \u0000D\u0000o\u0000 \u0000y\u0000o\u0000u\u0000 \u0000w\u0000i\u0000s\u0000h\u0000 \u0000t\u0000o\u0000\n\u0000c\u0000o\u0000n\u0000t\u0000i\u0000n\u0000u\u0000e\u0000 \u0000a\u0000n\u0000d\u0000 \u0000t\u0000r\u0000y\u0000 \u0000t\u0000o\u0000 \u0000e\u0000x\u0000t\u0000r\u0000a\u0000c\u0000t\u0000 \u0000w\u0000a\u0000v\u0000e\u0000f\u0000o\u0000r\u0000m\u0000 \u0000f\u0000r\u0000o\u0000m\u0000 \u0000i\u0000t\u0000\n\u0000(\u0000m\u0000a\u0000y\u0000 \u0000t\u0000a\u0000k\u0000e\u0000 \u0000s\u0000e\u0000v\u0000e\u0000r\u0000a\u0000l\u0000 \u0000s\u0000e\u0000c\u0000o\u0000n\u0000d\u0000s\u0000)\u0000?\u0000", "åeöNò]_cOW.\u0000 \u0000`Oó`\n\u0000ç~í~,\u0000v^ÕþVÐcÖSâlb_\n\u0000(\u0000ïSý±9àQÒy)\u0000?\u0000", "tÇ \u0000\fÓ|Ç@Ç \u0000ÁÁÀ\u0018´\u0000ÆµÂÈ²ä².\u0000 \u0000\fÓ|Ç\\¸½0Ñ \u0000\fÓ\u0015ÖDÇ \u0000ÍÍXÕ ¬µÂÈ²L®?\u0000(\u0000ÜÂ\u0004¬tÇ \u0000x¬´¹\u0018Â \u0000ÇµÂÈ²ä².\u0000)\u0000"]] _ string[][] [["I\u0000n\u0000p\u0000u\u0000t\u0000 \u0000V\u0000a\u0000l\u0000u\u0000e\u0000 \u0000E\u0000r\u0000r\u0000o\u0000r\u0000", "eQ<P\u0019ï", "…Çl­\u0012¬tÇ \u0000ÀÒ½¹È²ä².\u0000"], ["S\u0000e\u0000l\u0000e\u0000c\u0000t\u0000 \u0000f\u0000i\u0000l\u0000e\u0000 \u0000t\u0000o\u0000 \u0000p\u0000l\u0000a\u0000y\u0000 \u0000a\u0000n\u0000d\u0000 \u0000c\u0000l\u0000i\u0000c\u0000k\u0000 \u0000O\u0000p\u0000e\u0000n\u0000", "\tébeöNSb6q\u000eTSb\u0000_", "¬ÇÝÀXÕ$¸”² \u0000\fÓ|ÇDÇ \u0000 ÁÝÐXÕà¬ \u0000ôÅ0®è²”Í|¹ \u0000\u0004²t¹íÂÜÂ$Æ.\u0000"], ["W\u0000r\u0000o\u0000n\u0000g\u0000 \u0000d\u0000a\u0000t\u0000a\u0000 \u0000t\u0000y\u0000p\u0000e\u0000 \u0000n\u0000a\u0000m\u0000e\u0000 \u0000f\u0000o\u0000r\u0000 \u0000t\u0000h\u0000i\u0000s\u0000 \u0000c\u0000o\u0000n\u0000v\u0000e\u0000r\u0000s\u0000i\u0000o\u0000n\u0000 \u0000V\u0000I\u0000.\u0000", "dkHr,gV\u0000I\u0000„vpenc{|‹W\u0019•ï‹.\u0000", "ÇÌ¸\u0015ÖÝÂtÇ \u0000ÀÒ½¹È²ä².\u0000"], ["D\u0000o\u0000n\u0000'\u0000t\u0000 \u0000e\u0000x\u0000i\u0000s\u0000t\u0000 \u0000f\u0000i\u0000l\u0000e\u0000 \u0000o\u0000r\u0000 \u0000i\u0000n\u0000c\u0000o\u0000r\u0000r\u0000e\u0000c\u0000t\u0000 \u0000f\u0000i\u0000l\u0000e\u0000 \u0000f\u0000o\u0000r\u0000m\u0000a\u0000t\u0000.\u0000", "\rNX[(W„v‡eöN\u0016b‡eöN<h\u000f_\rNcknx.\u0000", "\fÓ|ÇtÇ \u0000tÈ¬ÇXÕÀÉ \u0000JÅp¬˜° \u0000\fÓ|Ç\u0015ÖÝÂtÇ \u0000(ÌtÇ©°È²ä².\u0000"], ["C\u0000a\u0000n\u0000 \u0000n\u0000o\u0000t\u0000 \u0000o\u0000p\u0000e\u0000n\u0000 \u0000A\u0000S\u0000I\u0000O\u0000 \u0000D\u0000r\u0000i\u0000v\u0000e\u0000r\u0000.\u0000", "~b\rN0RA\u0000S\u0000I\u0000O\u0000q¨R\u000bz^.\u0000", "A\u0000S\u0000I\u0000O\u0000Ü´|·tÇ„¼|¹ \u0000>ÌDÇ\u0018Â \u0000ÆÅµÂÈ²ä².\u0000"]] string[][] [["T\u0000h\u0000e\u0000 \u0000s\u0000o\u0000u\u0000n\u0000d\u0000 \u0000c\u0000a\u0000r\u0000d\u0000 \u0000i\u0000s\u0000 \u0000n\u0000o\u0000t\u0000 \u0000r\u0000e\u0000t\u0000u\u0000r\u0000n\u0000i\u0000n\u0000g\u0000 \u0000d\u0000a\u0000t\u0000a\u0000.\u0000\n\u0000T\u0000h\u0000e\u0000 \u0000V\u0000o\u0000l\u0000t\u0000m\u0000e\u0000t\u0000e\u0000r\u0000 \u0000w\u0000i\u0000l\u0000l\u0000 \u0000b\u0000e\u0000 \u0000c\u0000l\u0000o\u0000s\u0000e\u0000d\u0000.\u0000\n\u0000Y\u0000o\u0000u\u0000 \u0000m\u0000a\u0000y\u0000 \u0000r\u0000e\u0000-\u0000r\u0000u\u0000n\u0000 \u0000V\u0000o\u0000l\u0000t\u0000m\u0000e\u0000t\u0000e\u0000r\u0000 \u0000i\u0000f\u0000 \u0000y\u0000o\u0000u\u0000 \u0000w\u0000i\u0000s\u0000h\u0000.\u0000", "ðXaS\rNÔÞVpenc\u000205uSh\u0006\\«sQí\u00020\n\u0000`OïSåNÍ°e5uShYg`O?a\u000favÝ\u00020", "Á¬¹tÎÜ´² \u0000ÇÌ¸|¹ \u0000Íl­XÕÀÉ \u0000JÅà¬ÇµÂÈ²ä².\u0000\n\u0000Ì¹¥²!Î\u0015ÈÄ¬0®|¹ \u0000ë²à¬ \u0000ä²ÜÂ \u0000äÂÕÜÂ¤ÐíÂÜÂ$Æ.\u0000"], ["W\u0000r\u0000o\u0000n\u0000g\u0000 \u0000d\u0000a\u0000t\u0000a\u0000 \u0000t\u0000y\u0000p\u0000e\u0000 \u0000n\u0000a\u0000m\u0000e\u0000 \u0000f\u0000o\u0000r\u0000 \u0000t\u0000h\u0000i\u0000s\u0000 \u0000c\u0000o\u0000n\u0000v\u0000e\u0000r\u0000s\u0000i\u0000o\u0000n\u0000 \u0000V\u0000I\u0000.\u0000", "dkHr,gV\u0000I\u0000„vpenc{|‹W\u0019•ï‹.\u0000", "ÇÌ¸\u0015ÖÝÂtÇ \u0000ÀÒ½¹È²ä².\u0000"]] _ string[][] [["W\u0000r\u0000o\u0000n\u0000g\u0000 \u0000d\u0000a\u0000t\u0000a\u0000 \u0000t\u0000y\u0000p\u0000e\u0000 \u0000n\u0000a\u0000m\u0000e\u0000 \u0000f\u0000o\u0000r\u0000 \u0000t\u0000h\u0000i\u0000s\u0000 \u0000c\u0000o\u0000n\u0000v\u0000e\u0000r\u0000s\u0000i\u0000o\u0000n\u0000 \u0000V\u0000I\u0000", "dkHr,gV\u0000I\u0000„vpenc{|‹W\u0019•ï‹.\u0000", "ÇÌ¸\u0015ÖÝÂtÇ \u0000ÀÒ½¹È²ä².\u0000"]] _ string[][] [["W\u0000r\u0000o\u0000n\u0000g\u0000 \u0000d\u0000a\u0000t\u0000a\u0000 \u0000t\u0000y\u0000p\u0000e\u0000 \u0000n\u0000a\u0000m\u0000e\u0000 \u0000f\u0000o\u0000r\u0000 \u0000t\u0000h\u0000i\u0000s\u0000 \u0000c\u0000o\u0000n\u0000v\u0000e\u0000r\u0000s\u0000i\u0000o\u0000n\u0000 \u0000V\u0000I\u0000", "dkHr,gV\u0000I\u0000„vpenc{|‹W\u0019•ï‹.\u0000", "ÇÌ¸\u0015ÖÝÂtÇ \u0000ÀÒ½¹È²ä².\u0000"]] string[][] [["C\u0000a\u0000n\u0000'\u0000t\u0000 \u0000s\u0000a\u0000v\u0000e\u0000 \u0000f\u0000i\u0000l\u0000e\u0000.\u0000\n\u0000P\u0000l\u0000e\u0000a\u0000s\u0000e\u0000 \u0000c\u0000o\u0000n\u0000f\u0000i\u0000r\u0000m\u0000 \u0000O\u0000p\u0000e\u0000r\u0000a\u0000t\u0000o\u0000r\u0000 \u0000s\u0000t\u0000a\u0000r\u0000t\u0000u\u0000p\u0000 \u0000c\u0000o\u0000n\u0000f\u0000i\u0000g\u0000u\u0000r\u0000a\u0000t\u0000i\u0000o\u0000n\u0000 \u0000p\u0000a\u0000t\u0000h\u0000 \u0000o\u0000r\u0000 \u0000u\u0000s\u0000i\u0000n\u0000g\u0000 \u0000s\u0000a\u0000t\u0000e\u0000.\u0000\n\u0000P\u0000l\u0000e\u0000a\u0000s\u0000e\u0000,\u0000 \u0000u\u0000s\u0000e\u0000 \u0000a\u0000n\u0000o\u0000t\u0000h\u0000e\u0000r\u0000 \u0000f\u0000i\u0000l\u0000e\u0000 \u0000n\u0000a\u0000m\u0000e\u0000.\u0000", "àeÕlÝOX[eöN\u00020\n\u0000÷nx¤Íd\\OXT/T¨RMnï_\u0016b\u0005O(ul9r\u00020\n\u0000÷O(uæS\u0000N*NeöN\rT\u00020\u0000\u0000", "äÂÜÂ\u0004¬ü¬\u001cÈ,¸ \u0000ÜÂ‘ÇDÇ \u0000\u0004Ç\\Õ \u0000XÖ½¬\fÓ|ÇDÇ \u0000ô¼\u0000­`Õ\u0018Â \u0000ÆÅµÂÈ²ä².\u0000\n\u0000ä²x¹ \u0000\u0004Õ\\¸ø­Œ·tÇ \u0000¬À©ÆXÕà¬ \u0000ˆÇà´ÀÉ \u0000µÑ\\¸\u0000¬ \u0000˜Ç»º\u0018´\u0000ÆµÂÈ²ä².\u0000\n\u0000ä²x¹ \u0000tÇ„¹<Ç\\¸ \u0000ô¼\u0000­XÕíÂÜÂ$Æ.\u0000"], ["C\u0000a\u0000n\u0000'\u0000t\u0000 \u0000l\u0000o\u0000a\u0000d\u0000 \u0000f\u0000i\u0000l\u0000e\u0000.\u0000\n\u0000P\u0000l\u0000e\u0000a\u0000s\u0000e\u0000 \u0000c\u0000o\u0000n\u0000f\u0000i\u0000r\u0000m\u0000 \u0000O\u0000p\u0000e\u0000r\u0000a\u0000t\u0000o\u0000r\u0000 \u0000s\u0000t\u0000a\u0000r\u0000t\u0000u\u0000p\u0000 \u0000c\u0000o\u0000n\u0000f\u0000i\u0000g\u0000u\u0000r\u0000a\u0000t\u0000i\u0000o\u0000n\u0000 \u0000p\u0000a\u0000t\u0000h\u0000 \u0000o\u0000r\u0000 \u0000u\u0000s\u0000i\u0000n\u0000g\u0000 \u0000s\u0000a\u0000t\u0000e\u0000.\u0000", "àeÕlÅ}eöN\u00020\n\u0000÷nx¤Íd\\OXT/T¨RMnï_\u0016b\u0005O(ul9r\u00020\u0000\u0000", "äÂÜÂ\u0004¬ü¬\u001cÈ,¸ \u0000ÜÂ‘ÇDÇ \u0000\u0004Ç\\Õ \u0000XÖ½¬\fÓ|ÇDÇ \u0000}ÇDÇ\u0018ÂÆÅµÂÈ²ä².\u0000\n\u0000ä²x¹ \u0000\u0004Õ\\¸ø­Œ·tÇ \u0000¬À©ÆXÕà¬ \u0000ˆÇà´ÀÉ \u0000µÑ\\¸\u0000¬ \u0000˜Ç»º\u0018´\u0000ÆµÂÈ²ä².\u0000"], ["C\u0000a\u0000n\u0000'\u0000t\u0000 \u0000l\u0000o\u0000a\u0000d\u0000 \u0000f\u0000i\u0000l\u0000e\u0000.\u0000 \u0000d\u0000a\u0000t\u0000a\u0000 \u0000f\u0000o\u0000r\u0000m\u0000a\u0000t\u0000 \u0000m\u0000i\u0000s\u0000t\u0000a\u0000k\u0000e\u0000s\u0000.\u0000", "àeÕlÅ}eöN\u00020penc<h\u000f_\u0019ï\u00020", "äÂÜÂ\u0004¬ü¬\u001cÈ,¸ \u0000ÜÂ‘ÇDÇ \u0000\u0004Ç\\Õ \u0000XÖ½¬\fÓ|ÇDÇ \u0000}ÇDÇ\u0018ÂÆÅµÂÈ²ä².\u0000\n\u0000\fÓ|Ç\u0015ÖÝÂtÇ \u0000(ÌtÇ©°È²ä².\u0000"]] string[][] [["W\u0000r\u0000o\u0000n\u0000g\u0000 \u0000d\u0000a\u0000t\u0000a\u0000 \u0000t\u0000y\u0000p\u0000e\u0000 \u0000n\u0000a\u0000m\u0000e\u0000 \u0000f\u0000o\u0000r\u0000 \u0000t\u0000h\u0000i\u0000s\u0000 \u0000c\u0000o\u0000n\u0000v\u0000e\u0000r\u0000s\u0000i\u0000o\u0000n\u0000 \u0000V\u0000I\u0000", "dkHr,gV\u0000I\u0000„vpenc{|‹W\u0019•ï‹.\u0000", "ÇÌ¸\u0015ÖÝÂtÇ \u0000ÀÒ½¹È²ä².\u0000"]] string[][] [["W\u0000r\u0000o\u0000n\u0000g\u0000 \u0000d\u0000a\u0000t\u0000a\u0000 \u0000t\u0000y\u0000p\u0000e\u0000 \u0000n\u0000a\u0000m\u0000e\u0000 \u0000f\u0000o\u0000r\u0000 \u0000t\u0000h\u0000i\u0000s\u0000 \u0000c\u0000o\u0000n\u0000v\u0000e\u0000r\u0000s\u0000i\u0000o\u0000n\u0000 \u0000V\u0000I\u0000", "dkHr,gV\u0000I\u0000„vpenc{|‹W\u0019•ï‹.\u0000", "ÇÌ¸\u0015ÖÝÂtÇ \u0000ÀÒ½¹È²ä².\u0000"]] string[][] [["W\u0000r\u0000o\u0000n\u0000g\u0000 \u0000d\u0000a\u0000t\u0000a\u0000 \u0000t\u0000y\u0000p\u0000e\u0000 \u0000n\u0000a\u0000m\u0000e\u0000 \u0000f\u0000o\u0000r\u0000 \u0000t\u0000h\u0000i\u0000s\u0000 \u0000v\u0000e\u0000r\u0000s\u0000i\u0000o\u0000n\u0000 \u0000V\u0000I\u0000", "dkHr,gV\u0000I\u0000„vpenc{|‹W\u0019•ï‹.\u0000", "ÇÌ¸\u0015ÖÝÂtÇ \u0000ÀÒ½¹È²ä².\u0000"]] string[][] [["W\u0000r\u0000o\u0000n\u0000g\u0000 \u0000d\u0000a\u0000t\u0000a\u0000 \u0000t\u0000y\u0000p\u0000e\u0000 \u0000n\u0000a\u0000m\u0000e\u0000 \u0000f\u0000o\u0000r\u0000 \u0000t\u0000h\u0000i\u0000s\u0000 \u0000c\u0000o\u0000n\u0000v\u0000e\u0000r\u0000s\u0000i\u0000o\u0000n\u0000 \u0000V\u0000I\u0000", "\u0019ïvpenc{|Wv\rTðylbc.\u0000", "ÇÌ¸\u0015ÖÝÂtÇ \u0000ÀÒ½¹È²ä².\u0000"]] string[][] [["Y\u0000o\u0000u\u0000 \u0000d\u0000o\u0000 \u0000n\u0000o\u0000t\u0000 \u0000h\u0000a\u0000v\u0000e\u0000 \u0000t\u0000h\u0000 \u0000r\u0000e\u0000q\u0000u\u0000i\u0000r\u0000e\u0000d\u0000 \u0000o\u0000p\u0000t\u0000i\u0000o\u0000n\u0000a\u0000l\u0000 \u0000m\u0000o\u0000d\u0000u\u0000l\u0000e\u0000(\u0000s\u0000)\u0000 \u0000t\u0000o\u0000 \u0000r\u0000u\u0000n\u0000 \u0000t\u0000h\u0000i\u0000s\u0000 \u0000s\u0000e\u0000q\u0000u\u0000e\u0000n\u0000c\u0000e\u0000:\u0000\n\u0000F\u0000u\u0000l\u0000l\u0000 \u0000V\u0000e\u0000r\u0000s\u0000i\u0000o\u0000n\u0000 \u0000o\u0000f\u0000 \u0000C\u0000R\u0000Y\u00006\u00001\u00008\u00001\u0000", "`O¡l\tg*N\u0000ïS\t!jWW:NNÐLÙ*N^\u0017R\u001aÿ \u0000\n\u0000C\u0000R\u0000Y\u00006\u00001\u00008\u00001\u0000v[teHr,g", "tÇ \u0000ü¬\u001cÈ,¸DÇ \u0000äÂ‰ÕXÕ”² \u0000p³ \u0000DÕ”Æ\\Õ \u0000¨ºÈ´tÇ \u0000ÆÅµÂÈ²ä²:\u0000 \u0000\n\u0000C\u0000R\u0000Y\u00006\u00001\u00008\u00001\u0000XÇ \u0000DÆ\u0004È\u0010Óø¼"], ["Y\u0000o\u0000u\u0000 \u0000c\u0000a\u0000n\u0000 \u0000n\u0000o\u0000t\u0000 \u0000s\u0000a\u0000v\u0000e\u0000 \u0000t\u0000h\u0000i\u0000s\u0000 \u0000s\u0000e\u0000q\u0000u\u0000e\u0000n\u0000c\u0000e\u0000 \u0000i\u0000n\u0000 \u0000C\u0000R\u0000Y\u00006\u00001\u00008\u00001\u0000 \u0000O\u0000n\u0000e\u0000.\u0000\n\u0000R\u0000e\u0000f\u0000e\u0000r\u0000 \u0000f\u0000u\u0000l\u0000l\u0000 \u0000v\u0000e\u0000r\u0000s\u0000i\u0000o\u0000n\u0000 \u0000o\u0000f\u0000 \u0000C\u0000R\u0000Y\u00006\u00001\u00008\u00001\u0000.\u0000", "¨`\rNýÝOX[(WC\u0000R\u0000Y\u00006\u00001\u00008\u00001\u0000\u0000N*Nz^.\u0000\n\u0000^\fÿåNÝOX[\fÿO(u[teHrC\u0000R\u0000Y\u00006\u00001\u00008\u00001\u0000v.\u0000", "C\u0000R\u0000Y\u00006\u00001\u00008\u00001\u0000 \u0000O\u0000n\u0000e\u0000ÐÅ\u001cÁ \u0000tÇ \u0000ü¬\u001cÈ,¸DÇ \u0000ô¼\u0000­`Õ\u0018Â \u0000ÆÅµÂÈ²ä².\u0000\n\u0000ô¼\u0000­XÕÜÂ$¸tº \u0000C\u0000R\u0000Y\u00006\u00001\u00008\u00001\u0000XÇ \u0000DÆ\u0004È\u0010Óø¼DÇ \u0000¬¹©ÆXÕíÂÜÂ$Æ."], ["Y\u0000o\u0000u\u0000 \u0000c\u0000a\u0000n\u0000 \u0000o\u0000n\u0000l\u0000y\u0000 \u0000v\u0000i\u0000e\u0000w\u0000 \u0000s\u0000e\u0000q\u0000u\u0000e\u0000n\u0000c\u0000e\u0000 \u0000,\u0000 \u0000b\u0000u\u0000t\u0000 \u0000c\u0000a\u0000n\u0000 \u0000n\u0000o\u0000t\u0000 \u0000r\u0000u\u0000n\u0000 \u0000a\u0000n\u0000d\u0000 \u0000s\u0000a\u0000v\u0000e\u0000 \u0000i\u0000n\u0000 \u0000C\u0000R\u0000Y\u00006\u00001\u00008\u00001\u0000 \u0000O\u0000n\u0000e\u0000.\u0000\n\u0000R\u0000e\u0000f\u0000e\u0000r\u0000 \u0000f\u0000u\u0000l\u0000l\u0000 \u0000v\u0000e\u0000r\u0000s\u0000i\u0000o\u0000n\u0000 \u0000o\u0000f\u0000 \u0000C\u0000R\u0000Y\u00006\u00001\u00008\u00001\u0000.\u0000", "¨`êSýåg\u000bw^\u0017R\fÿFO\rNýÐLv^ÝOX[(WC\u0000R\u0000Y\u00006\u00001\u00008\u00001\u0000 \u0000O\u0000n\u0000e\u0000\u00020 \u0000\n\u0000:NNôf\u001aYvRýO(u[teHrC\u0000R\u0000Y\u00006\u00001\u00008\u00001\u0000\u00020", "C\u0000R\u0000Y\u00006\u00001\u00008\u00001\u0000 \u0000O\u0000n\u0000e\u0000ÐÅ\u001cÁ”² \u0000ü¬\u001cÈ,¸DÇ \u0000\u0004ÖÜÂÌ¹ \u0000`Õ\u0018Â \u0000ˆÇà¬ \u0000äÂ‰Õü¬ \u0000ô¼\u0000­@Ç \u0000`Õ\u0018Â \u0000ÆÅµÂÈ²ä².\u0000\n\u0000T³ \u0000Î¹@Ç \u00000®¥²DÇ \u0000\u0004ÇXÕìÅ\u001cÁ”² \u0000G\u0000V\u0000S\u0000o\u0000u\u0000n\u0000d\u0000L\u0000a\u0000b\u0000XÇ \u0000DÆ\u0004È\u0010Óø¼DÇ \u0000¬¹©ÆXÕíÂÜÂ$Æ.\u0000"]] string[][] [[""]]] -> w21
    tunnel: w8 -> [_ _ _ _ _ _ _ _ _ _ _ _ w38 _ _ w48 _ _ _ _ _ w66 _ _ _ _ _ w104 w135 _ _ _ _ _ _ _ _ _ _ _ _ _ _ _ _]
    tunnel: [_ _ _ _ _ _ _ _ _ _ _ _ w37 _ _ w47 _ _ _ _ _ _ _ _ _ _ _ _ _ _ _ _ _ _ _ _ _ _ _ _ _ _ _ _ _] -> w18
    tunnel: "Error No" -> [_ _ _ _ _ _ _ _ _ _ _ _ _ _ _ w46 _ _ _ _ _ w68 _ _ _ _ _ w105 w136 _ _ _ _ _ w345 _ w351 _ _ _ _ _ _ _ _]
    tunnel: [_ _ _ _ _ _ _ _ _ _ _ _ _ _ _ _ _ _ w51 _ _ _ string[][] [["V\u0000a\u0000l\u0000u\u0000e\u0000", "<P", "\u0012¬"], ["O\u0000p\u0000e\u0000r\u0000a\u0000n\u0000d\u0000 \u0000V\u0000a\u0000l\u0000u\u0000e\u0000", "Íd\\O<P", "ðÅ°À\u0018Â\u0012¬"], ["1\u0000/\u0000n\u0000 \u0000O\u0000c\u0000t\u0000a\u0000v\u0000e\u0000", "1\u0000/\u0000n\u0000 \u0000\rP‘˜\u000bz", "1\u0000/\u0000n\u0000%ÆÀÐ\f¾"], ["H\u0000z\u0000", "H\u0000z\u0000", "H\u0000z\u0000"], ["s\u0000", "s\u0000", "s\u0000"], ["O\u0000p\u0000e\u0000r\u0000a\u0000n\u0000d\u0000 \u0000B\u0000", "Íd\\Ope \u0000B\u0000", "ðÅ°À\u0018Â \u0000B\u0000"], ["O\u0000p\u0000e\u0000r\u0000a\u0000n\u0000d\u0000 \u0000B\u0000 \u0000(\u0000S\u0000i\u0000n\u0000g\u0000l\u0000e\u0000 \u0000V\u0000a\u0000l\u0000u\u0000e\u0000s\u0000)\u0000", "Íd\\Ope \u0000B\u0000 \u0000(\u0000US<P)\u0000", "ðÅ°À\u0018Â \u0000B\u0000 \u0000(\u0000è²\u001cÂ\u0012¬)\u0000"]] _ string[][] [["U\u0000p\u0000p\u0000e\u0000r\u0000 \u0000L\u0000i\u0000m\u0000i\u0000t\u0000", "\nNP–", "ÃÆ\\ÕÄ¬"], ["L\u0000o\u0000w\u0000e\u0000r\u0000 \u0000L\u0000i\u0000m\u0000i\u0000t\u0000", "\u000bNP–", "DÅ˜·\\ÕÄ¬"], ["D\u0000a\u0000t\u0000a\u0000", "penc", "ÇÌ¸"], ["C\u0000r\u0000i\u0000t\u0000i\u0000c\u0000a\u0000l\u0000 \u0000P\u0000o\u0000i\u0000n\u0000t\u0000s\u0000", "4NLu¹p", "¼¹Ä¬\u0010È"], ["A\u0000l\u0000i\u0000g\u0000n\u0000m\u0000e\u0000n\u0000t\u0000 \u0000R\u0000e\u0000f\u0000", "ù[ÆQÂS\u0003€", "\u0011ÉìÂ8Ìà¬"], ["U\u0000p\u0000p\u0000e\u0000r\u0000 \u0000F\u0000a\u0000i\u0000l\u0000e\u0000d\u0000", "\nN1Y%¹p", "ÃÆäÂ(Ó\u0010È"], ["L\u0000o\u0000w\u0000e\u0000r\u0000 \u0000F\u0000a\u0000i\u0000l\u0000e\u0000d\u0000", "\u000bN1Y%¹p", "DÅ˜·äÂ(Ó\u0010È"], ["M\u0000a\u0000r\u0000g\u0000i\u0000n\u0000", "箯\u0018", "浆默"], ["V\u0000a\u0000l\u0000u\u0000e\u0000", "US<P", "\u0012¬"], ["I\u0000n\u0000d\u0000i\u0000v\u0000i\u0000d\u0000u\u0000a\u0000l\u0000 \u0000P\u0000o\u0000i\u0000n\u0000t\u0000s\u0000", "*N+R¹p", "\u001c¬Ä¼\u0010È"], ["A\u0000b\u0000s\u0000o\u0000l\u0000u\u0000t\u0000e\u0000 \u0000L\u0000i\u0000m\u0000i\u0000t\u0000s\u0000", "Ý~ù[P–6R", "\bÈ\u0000³\\ÕÄ¬"], ["F\u0000l\u0000o\u0000a\u0000t\u0000i\u0000n\u0000g\u0000 \u0000L\u0000i\u0000m\u0000i\u0000t\u0000s\u0000", "nm¨RP–6R", "X¹Ù³\\ÕÄ¬"], ["F\u0000l\u0000o\u0000a\u0000t\u0000i\u0000n\u0000g\u0000 \u0000D\u0000a\u0000t\u0000a\u0000", "nm¨Rpenc", "X¹Ù³ÇÌ¸"], ["A\u0000l\u0000i\u0000g\u0000n\u0000e\u0000d\u0000 \u0000L\u0000i\u0000m\u0000i\u0000t\u0000s\u0000", "ù[PŸP–6R", "\u0015È,¸\\ÕÄ¬"], ["A\u0000l\u0000i\u0000g\u0000n\u0000e\u0000d\u0000 \u0000D\u0000a\u0000t\u0000a\u0000", "ù[PŸpenc", "\u0015È,¸ÇÌ¸"]] _ _ _ _ string[][] [["D\u0000a\u0000t\u0000a\u0000", "penc", "ÇÌ¸"], ["R\u0000e\u0000s\u0000u\u0000l\u0000t\u0000s\u0000", "Ó~œg", "°¬ü¬\u0012¬"], ["W\u0000a\u0000v\u0000e\u0000f\u0000o\u0000r\u0000m\u0000s\u0000", "âlb_", "ÜÂ\u0004¬\fÓ\u0015Ö"], ["E\u0000n\u0000t\u0000e\u0000r\u0000 \u0000c\u0000o\u0000m\u0000m\u0000e\u0000n\u0000t\u0000 \u0000f\u0000o\u0000r\u0000 \u0000d\u0000a\u0000t\u0000a\u0000f\u0000i\u0000l\u0000e\u0000:\u0000", "eQeöNèlã.\u0000", "ÇÌ¸\fÓ|ÇXÇ \u0000üÈtÕ|¹ \u0000Ç%¸XÕíÂÜÂ$Æ.\u0000"], ["E\u0000n\u0000t\u0000e\u0000r\u0000 \u0000d\u0000a\u0000t\u0000a\u0000 \u0000f\u0000i\u0000l\u0000e\u0000n\u0000a\u0000m\u0000e\u0000 \u0000(\u0000n\u0000o\u0000 \u0000e\u0000x\u0000t\u0000e\u0000n\u0000s\u0000i\u0000o\u0000n\u0000)\u0000:\u0000", "eQpenceöNv\rTW[(\u0000¡l\tgibU\\\rT)\u0000:\u0000", "ÇÌ¸\fÓ|ÇtÇ¹DÇ \u0000Ç%¸XÕíÂÜÂ$Æ(\u0000UÖ¥ÇÇÆÅLÇ)\u0000:\u0000"]] _ string[][] [["F\u0000i\u0000l\u0000e\u0000 \u0000P\u0000a\u0000t\u0000h\u0000", "eöNï_", "\fÓ|Ç½¬\\¸"], ["B\u0000a\u0000s\u0000e\u0000 \u0000P\u0000a\u0000t\u0000h\u0000", "úW0Wï_", "0®\u0000É½¬\\¸"]] _ _ w346 _ w352 _ _ _ _ _ _ _ _] -> w15
    tunnel: "String In" -> [_ _ _ _ _ _ _ _ _ _ _ _ _ _ _ _ _ _ w52 _ _ w65 _ _ _ _ _ _ _ _ _ _ _ _ _ _ _ _ _ _ _ _ _ _ _]
    tunnel: [_ _ _ _ _ _ _ _ _ _ _ _ _ _ _ _ _ _ _ _ _ w67 _ _ _ _ _ w108 w134 _ _ _ _ _ _ _ _ _ _ _ _ _ _ _ _] -> w10
    tunnel: w7 -> [_ _ _ _ _ _ _ _ _ _ _ _ _ _ _ _ _ _ _ _ _ w63 _ _ _ _ _ w107 w132 _ _ _ _ _ _ _ _ _ _ _ _ _ _ _ _]
    frame "Main" {
      # "11"
    }
    frame "Login" {
    }
    frame "Project" {
      # "25"
      # "23"
      # "20"
      # "22"
    }
    frame "WorkState" {
    }
    frame "Curves Library" {
      # "17"
    }
    frame "Graph" {
    }
    frame "Add Step" {
      # "11"
    }
    frame "Add Step Sub" {
    }
    frame "Step Setup" {
    }
    frame "ViewData" {
      # "4"
    }
    frame "Document" {
    }
    frame "SoundCard" {
      # "9"
    }
    frame "SoundCard Sub" {
      w39 = string[][] [["A\u0000d\u0000d\u0000 \u0000A\u0000u\u0000d\u0000i\u0000o\u0000 \u0000O\u0000u\u0000t\u0000p\u0000u\u0000t\u0000 \u0000C\u0000h\u0000a\u0000n\u0000n\u0000e\u0000l\u0000", "ûm RóúQ\u001aS.\u0000", "œÍl­µÑ\\¸tÇ„¹DÇ \u0000”Í\u0000¬iÕÈ²ä².\u0000"], ["D\u0000e\u0000l\u0000e\u0000t\u0000e\u0000 \u0000A\u0000u\u0000d\u0000i\u0000o\u0000 \u0000O\u0000u\u0000t\u0000p\u0000u\u0000t\u0000 \u0000C\u0000h\u0000a\u0000n\u0000n\u0000e\u0000l\u0000", " RdóúQ\u001aS.\u0000", "œÍl­µÑ\\¸tÇ„¹DÇ \u0000­À\u001cÈiÕÈ²ä².\u0000"], ["R\u0000e\u0000n\u0000a\u0000m\u0000e\u0000 \u0000A\u0000u\u0000d\u0000i\u0000o\u0000 \u0000O\u0000u\u0000t\u0000p\u0000u\u0000t\u0000 \u0000C\u0000h\u0000a\u0000n\u0000n\u0000e\u0000l\u0000", "9eØSóúQ\u001aS.\u0000", "œÍl­µÑ\\¸tÇ„¹DÇ \u0000À¼½¬iÕÈ²ä².\u0000"], ["A\u0000d\u0000d\u0000 \u0000A\u0000u\u0000d\u0000i\u0000o\u0000 \u0000I\u0000n\u0000p\u0000u\u0000t\u0000 \u0000C\u0000h\u0000a\u0000n\u0000n\u0000e\u0000l\u0000", "ûm RóeQ\u001aS.\u0000", "…Çl­µÑ\\¸tÇ„¹DÇ \u0000”Í\u0000¬iÕÈ²ä².\u0000"], ["D\u0000e\u0000l\u0000e\u0000t\u0000e\u0000 \u0000A\u0000u\u0000d\u0000i\u0000o\u0000 \u0000I\u0000n\u0000p\u0000u\u0000t\u0000 \u0000C\u0000h\u0000a\u0000n\u0000n\u0000e\u0000l\u0000", "mdóeQ\u001aS.\u0000", "…Çl­µÑ\\¸tÇ„¹DÇ \u0000­À\u001cÈiÕÈ²ä².\u0000"], ["R\u0000e\u0000n\u0000a\u0000m\u0000e\u0000 \u0000A\u0000u\u0000d\u0000i\u0000o\u0000 \u0000I\u0000n\u0000p\u0000u\u0000t\u0000 \u0000C\u0000h\u0000a\u0000n\u0000n\u0000e\u0000l\u0000", "9eØSóeQ\u001aS.\u0000", "…Çl­µÑ\\¸tÇ„¹DÇ \u0000À¼½¬iÕÈ²ä².\u0000"]]
      n4 = Index Array(array=w39, index (col)=w38) -> (element=w37:string[])  [unwired: 1 in]
    }
    frame "Hardware" {
    }
    frame "Calibration" {
      # "13"
      # "11"
      # "9"
      # "8"
    }
    frame "Calibration Sub" {
      n5 = Equal To 0?(x=w46) -> (x = 0?=w45:bool)
      n6 = Select(t=string[][] [["A\u0000d\u0000d\u0000 \u0000C\u0000a\u0000l\u0000i\u0000b\u0000r\u0000a\u0000t\u0000e\u0000d\u0000 \u0000D\u0000e\u0000v\u0000i\u0000c\u0000e\u0000 \u0000N\u0000a\u0000m\u0000e\u0000", "ûm R!hÆQ¾‹\u0007Y\rTðy.\u0000", "P­\u0000É\\Õ \u0000¥ÇXÎtÇ„¹DÇ \u0000”Í\u0000¬iÕÈ²ä².\u0000"], ["D\u0000e\u0000l\u0000e\u0000t\u0000e\u0000 \u0000C\u0000a\u0000l\u0000i\u0000b\u0000r\u0000a\u0000t\u0000e\u0000d\u0000 \u0000D\u0000e\u0000v\u0000i\u0000c\u0000e\u0000 \u0000N\u0000a\u0000m\u0000e\u0000", " Rd–!hÆQ¾‹\u0007Y\rTðy.\u0000", "P­\u0000É\\Õ \u0000¥ÇXÎtÇ„¹DÇ \u0000­À\u001cÈiÕÈ²ä².\u0000"], ["R\u0000e\u0000n\u0000a\u0000m\u0000e\u0000 \u0000C\u0000a\u0000l\u0000i\u0000b\u0000r\u0000a\u0000t\u0000e\u0000d\u0000 \u0000D\u0000e\u0000v\u0000i\u0000c\u0000e\u0000 \u0000N\u0000a\u0000m\u0000e\u0000", "9eØS!hÆQ¾‹\u0007Y\rTðy.\u0000", "P­\u0000É\\Õ \u0000¥ÇXÎtÇ„¹DÇ \u0000À¼½¬iÕÈ²ä².\u0000"], ["C\u0000o\u0000p\u0000y\u0000 \u0000C\u0000a\u0000l\u0000i\u0000b\u0000r\u0000a\u0000t\u0000e\u0000d\u0000 \u0000D\u0000e\u0000v\u0000i\u0000c\u0000e\u0000 \u0000N\u0000a\u0000m\u0000e\u0000", "\rY6R!hÆQ¾‹\u0007Y\rTðy.\u0000", "P­\u0000É\\Õ \u0000¥ÇXÎtÇ„¹DÇ \u0000õ¼¬ÀiÕÈ²ä².\u0000"]], s=w45, f=string[][] [["N\u0000e\u0000w\u0000 \u0000S\u0000i\u0000g\u0000n\u0000a\u0000l\u0000 \u0000T\u0000y\u0000p\u0000e\u0000 \u0000N\u0000a\u0000m\u0000e\u0000", "°eváO÷S\u001aS\rTðy.\u0000", "ÈÀ\\¸´Æ \u0000àÂ8Ö\u0015ÖtÇ„¹"], ["D\u0000e\u0000l\u0000e\u0000t\u0000e\u0000d\u0000 \u0000S\u0000i\u0000g\u0000n\u0000a\u0000l\u0000 \u0000T\u0000y\u0000p\u0000e\u0000 \u0000N\u0000a\u0000m\u0000e\u0000", " RdáO÷S\u001aSv\rTðy.\u0000", "­À\u001cÈ`Õ \u0000àÂ8Ö\u0015ÖtÇ„¹"], ["N\u0000e\u0000w\u0000 \u0000C\u0000h\u0000a\u0000n\u0000g\u0000i\u0000n\u0000g\u0000 \u0000S\u0000i\u0000g\u0000n\u0000a\u0000l\u0000 \u0000T\u0000y\u0000p\u0000e\u0000 \u0000N\u0000a\u0000m\u0000e\u0000", "9eØSáO÷S\u001aSv\rTðy.\u0000", "À¼½¬`Õ \u0000ÈÀ\\¸´Æ \u0000àÂ8Ö\u0015ÖtÇ„¹"], ["N\u0000e\u0000w\u0000 \u0000S\u0000i\u0000g\u0000n\u0000a\u0000l\u0000 \u0000T\u0000y\u0000p\u0000e\u0000 \u0000N\u0000a\u0000m\u0000e\u0000", "°eváO÷S\u001aSv\rTðy.\u0000", "ÈÀ\\¸´Æ \u0000àÂ8Ö\u0015ÖtÇ„¹"]]) -> (s? t:f=w42:string[][])
      n7 = Index Array(array=w42, index (col)=w48) -> (element=w47:string[])  [unwired: 1 in]
    }
    frame "Messages" {
    }
    frame "Stimulus" {
      # "9"
    }
    frame "Stimulus Sub" {
      n8 = case shown="\"wavefile\"" w52 {
        tunnel: [string[][] [["S\u0000t\u0000i\u0000m\u0000u\u0000l\u0000u\u0000s\u0000 \u0000T\u0000y\u0000p\u0000e\u0000", "Ào±R{|‹W", "Çù­àÂ8Ö\u0015ÖÜÐ"], ["L\u0000e\u0000v\u0000e\u0000l\u0000(\u0000V\u0000)\u0000", "E^¦^(\u0000V\u0000)\u0000", "\u0000É\u0004Ç(\u0000V\u0000)\u0000"], ["S\u0000t\u0000a\u0000r\u0000t\u0000 \u0000F\u0000r\u0000e\u0000q\u0000(\u0000H\u0000z\u0000)\u0000", "\u0000_ËY‘˜‡s(\u0000H\u0000z\u0000)\u0000", "ÜÂ‘Ç(\u0000H\u0000z\u0000)\u0000"], ["S\u0000t\u0000o\u0000p\u0000 \u0000F\u0000r\u0000e\u0000q\u0000(\u0000H\u0000z\u0000)\u0000", "\\Pbk‘˜‡s(\u0000H\u0000z\u0000)\u0000", "\u0015ÈÀÉ(\u0000H\u0000z\u0000)\u0000"], ["C\u0000u\u0000r\u0000v\u0000e\u0000 \u0000v\u0000a\u0000l\u0000 \u0000l\u0000e\u0000v\u0000e\u0000l\u0000 \u0000n\u0000a\u0000m\u0000e\u0000", "òf¿~“^„v\rTðy", "á¬ Á\u001cÁà¬tÇ„¹"], ["U\u0000s\u0000e\u0000 \u0000C\u0000u\u0000r\u0000v\u0000e\u0000 \u0000V\u0000a\u0000l\u0000 \u0000l\u0000e\u0000v\u0000e\u0000l\u0000?\u0000", "òf¿~“^<P", "\u0012¬¬¹©Æ"], ["S\u0000t\u0000e\u0000p\u0000s\u0000 \u0000(\u0000#\u0000)\u0000", "ek¤š(\u0000#\u0000)\u0000", "x¬LÇ(\u0000#\u0000)\u0000"], ["C\u0000y\u0000c\u0000l\u0000e\u0000s\u0000/\u0000s\u0000t\u0000e\u0000p\u0000(\u0000#\u0000)\u0000", "hT\u001fg/\u0000ek(\u0000#\u0000)\u0000", "\\ÍŒÁüÈ0®(\u0000#\u0000)\u0000"], ["T\u0000i\u0000m\u0000e\u0000/\u0000s\u0000t\u0000e\u0000p\u0000 \u0000(\u0000s\u0000)\u0000", "öeô•/\u0000ek(\u0000s\u0000)\u0000", "\\ÍŒÁÜÂ\u0004¬(\u0000s\u0000)\u0000"], ["S\u0000t\u0000e\u0000p\u0000 \u0000R\u0000e\u0000s\u0000o\u0000l\u0000u\u0000t\u0000i\u0000o\u0000n\u0000", "ekÛ\u0006R¨s", "„½tÕ¥²"]] string[][] [["S\u0000t\u0000i\u0000m\u0000u\u0000l\u0000u\u0000s\u0000 \u0000T\u0000y\u0000p\u0000e\u0000", "Ào±R{|‹W", "Çù­àÂ8Ö\u0015ÖÜÐ"], ["L\u0000e\u0000v\u0000e\u0000l\u0000(\u0000V\u0000)\u0000", "E^¦^(\u0000V\u0000)\u0000", "\u0000É\u0004Ç(\u0000V\u0000)\u0000"], ["S\u0000t\u0000a\u0000r\u0000t\u0000 \u0000F\u0000r\u0000e\u0000q\u0000(\u0000H\u0000z\u0000)\u0000", "\u0000_ËY‘˜‡s(\u0000H\u0000z\u0000)\u0000", "ÜÂ‘Ç(\u0000H\u0000z\u0000)\u0000"], ["S\u0000t\u0000o\u0000p\u0000 \u0000F\u0000r\u0000e\u0000q\u0000(\u0000H\u0000z\u0000)\u0000", "\\Pbk‘˜‡s(\u0000H\u0000z\u0000)\u0000", "\u0015ÈÀÉ(\u0000H\u0000z\u0000)\u0000"], ["S\u0000w\u0000e\u0000e\u0000p\u0000 \u0000R\u0000a\u0000t\u0000e\u0000(\u0000s\u0000/\u0000d\u0000e\u0000c\u0000)\u0000", "kbÏc\u001fs(\u0000s\u0000/\u0000d\u0000e\u0000c\u0000)\u0000", "üÈ¬À`¹(\u0000s\u0000/\u0000d\u0000e\u0000c\u0000)\u0000"], ["U\u0000s\u0000e\u0000 \u0000C\u0000u\u0000r\u0000v\u0000e\u0000 \u0000V\u0000a\u0000l\u0000 \u0000l\u0000e\u0000v\u0000e\u0000l\u0000?\u0000", "òf¿~“^<P", "\u0012¬¬¹©Æ"], ["C\u0000u\u0000r\u0000v\u0000e\u0000 \u0000v\u0000a\u0000l\u0000 \u0000l\u0000e\u0000v\u0000e\u0000l\u0000 \u0000n\u0000a\u0000m\u0000e\u0000", "òf¿~“^„v\rTðy", "á¬ Á\u001cÁà¬tÇ„¹"], ["T\u0000S\u0000R\u0000 \u0000p\u0000a\u0000r\u0000a\u0000m\u0000s\u0000", "T\u0000S\u0000R\u0000„vÂSpe", "T\u0000S\u0000R\u0000\fÓ|·Tº0Ñ"]] string[][] [["S\u0000t\u0000i\u0000m\u0000u\u0000l\u0000u\u0000s\u0000 \u0000T\u0000y\u0000p\u0000e\u0000", "Ào±R{|‹W", "Çù­àÂ8Ö\u0015ÖÜÐ"], ["F\u0000r\u0000e\u0000q\u0000(\u0000H\u0000z\u0000)\u0000", "‘˜‡s(\u0000H\u0000z\u0000)\u0000", "üÈ\fÓ\u0018Â(\u0000H\u0000z\u0000)\u0000"], ["S\u0000t\u0000e\u0000p\u0000s\u0000(\u0000#\u0000)\u0000", "ek¤š(\u0000#\u0000)\u0000", "x¬LÇ"], ["C\u0000y\u0000c\u0000l\u0000e\u0000s\u0000(\u0000#\u0000)\u0000", "hT\u001fg(\u0000#\u0000)\u0000", "üÈ0®"], ["U\u0000s\u0000e\u0000 \u0000C\u0000u\u0000r\u0000v\u0000e\u0000 \u0000V\u0000a\u0000l\u0000 \u0000f\u0000r\u0000e\u0000w\u0000q\u0000?\u0000", "òf¿~“^<P", "\u0012¬¬¹©Æ"], ["C\u0000u\u0000r\u0000v\u0000e\u0000 \u0000v\u0000a\u0000l\u0000 \u0000l\u0000e\u0000v\u0000e\u0000l\u0000 \u0000n\u0000a\u0000m\u0000e\u0000", "òf¿~“^„v\rTðy", "á¬ Á\u001cÁà¬tÇ„¹"], ["S\u0000t\u0000a\u0000r\u0000t\u0000 \u0000A\u0000m\u0000p\u0000l\u0000(\u0000V\u0000)\u0000", "\u0000_ËYE^¦^(\u0000V\u0000)\u0000", "ÜÂ‘ÇÄÉíÓ(\u0000V\u0000)\u0000"], ["S\u0000t\u0000o\u0000p\u0000 \u0000A\u0000m\u0000p\u0000l\u0000(\u0000V\u0000)\u0000", "\\PbkE^¦^(\u0000V\u0000)\u0000", "\u0015ÈÀÉÄÉíÓ(\u0000V\u0000)\u0000"]] string[][] [["S\u0000t\u0000i\u0000m\u0000u\u0000l\u0000u\u0000s\u0000 \u0000T\u0000y\u0000p\u0000e\u0000", "Ào±R{|‹W", "Çù­àÂ8Ö\u0015ÖÜÐ"], ["L\u0000e\u0000v\u0000e\u0000l\u0000(\u0000V\u0000)\u0000", "E^¦^(\u0000V\u0000)\u0000", "\u0000É\u0004Ç(\u0000V\u0000)\u0000"], ["W\u0000a\u0000v\u0000e\u0000 \u0000P\u0000a\u0000t\u0000h\u0000", "âlï_", "1\u0000/\u0000n\u0000%ÆÀÐ\f¾"], ["W\u0000a\u0000v\u0000e\u0000 \u0000I\u0000n\u0000f\u0000o\u0000", "âláOo`", "\fÓ\u0015Ö\u0015Èô¼"], ["W\u0000a\u0000v\u0000e\u0000 \u0000T\u0000i\u0000m\u0000e\u0000", "âlöeô•", "\fÓ\u0015ÖÜÂ\u0004¬"], ["P\u0000e\u0000a\u0000k\u0000 \u0000V\u0000a\u0000l\u0000u\u0000e\u0000", "ð\\<P", "\\Í\u0000³\u0012¬"], ["R\u0000M\u0000S\u0000 \u0000V\u0000a\u0000l\u0000u\u0000e\u0000", "R\u0000M\u0000S\u0000<P", "R\u0000M\u0000S\u0000\u0012¬"], ["C\u0000u\u0000r\u0000v\u0000e\u0000 \u0000v\u0000a\u0000l\u0000 \u0000l\u0000e\u0000v\u0000e\u0000l\u0000 \u0000n\u0000a\u0000m\u0000e\u0000", "òf¿~“^„v\rTðy", "á¬ Á\u001cÁà¬tÇ„¹"], ["U\u0000s\u0000e\u0000 \u0000C\u0000u\u0000r\u0000v\u0000e\u0000 \u0000V\u0000a\u0000l\u0000 \u0000l\u0000e\u0000v\u0000e\u0000l\u0000?\u0000", "òf¿~“^<P", "\u0012¬¬¹©Æ"]] string[][] [["S\u0000t\u0000i\u0000m\u0000u\u0000l\u0000u\u0000s\u0000 \u0000T\u0000y\u0000p\u0000e\u0000", "Ào±R{|‹W", "Çù­àÂ8Ö\u0015ÖÜÐ"], ["L\u0000e\u0000v\u0000e\u0000l\u0000", "E^¦^", "\u0000É\u0004Ç"], ["d\u0000c\u0000 \u0000s\u0000r\u0000c\u0000 \u0000t\u0000y\u0000p\u0000e\u0000", "ôvAm5un{|W", "ÐÆœÌ\u0015ÖÜÐ"], ["d\u0000c\u0000m\u0000a\u0000x\u0000 \u0000I\u0000", "D\u0000C\u0000\u0000g'Y5uAm", "\\Í\u0000³\u0004ÈX¹"], ["d\u0000c\u0000 \u0000p\u0000o\u0000l\u0000a\u0000r\u0000", "ôvAmg'`", "ù­1Á"], ["d\u0000c\u0000 \u0000c\u0000t\u0000r\u0000l\u0000", "ôvAm§c6R", "pÈ…È)¼•¼"], ["S\u0000t\u0000e\u0000p\u0000s\u0000(\u0000#\u0000)\u0000", "ek¤š(\u0000#\u0000)\u0000", "x¬LÇ"], ["S\u0000t\u0000a\u0000r\u0000t\u0000 \u0000A\u0000m\u0000p\u0000l\u0000(\u0000V\u0000)\u0000", "\u0000_ËYE^¦^(\u0000V\u0000)\u0000", "ÜÂ‘ÇÄÉíÓ(\u0000V\u0000)\u0000"], ["S\u0000t\u0000o\u0000p\u0000 \u0000A\u0000m\u0000p\u0000l\u0000(\u0000V\u0000)\u0000", "\\PbkE^¦^(\u0000V\u0000)\u0000", "\u0015ÈÀÉÄÉíÓ(\u0000V\u0000)\u0000"], ["T\u0000i\u0000m\u0000e\u0000/\u0000s\u0000t\u0000e\u0000p\u0000(\u0000s\u0000)\u0000", "öeô•/\u0000ek(\u0000s\u0000)\u0000", "\\ÍŒÁÜÂ\u0004¬(\u0000s\u0000)\u0000"], ["S\u0000t\u0000e\u0000p\u0000 \u0000S\u0000i\u0000z\u0000e\u0000", "ek•", "x¬LÇlÐ0®"]] string[][] [["S\u0000t\u0000i\u0000m\u0000u\u0000l\u0000u\u0000s\u0000 \u0000T\u0000y\u0000p\u0000e\u0000", "Ào±R{|‹W", "Çù­àÂ8Ö\u0015ÖÜÐ"], ["T\u0000o\u0000n\u0000e\u0000 \u0000T\u0000y\u0000p\u0000e\u0000", "ó—{|‹W", "LÇpÈ\u0015ÖÜÐ"], ["S\u0000t\u0000e\u0000p\u0000s\u0000(\u0000#\u0000)\u0000", "ek¤š(\u0000#\u0000)\u0000", "x¬LÇ"], ["L\u0000e\u0000v\u0000e\u0000l\u0000(\u0000V\u0000)\u0000", "E^¦^(\u0000V\u0000)\u0000", "\u0000É\u0004Ç(\u0000V\u0000)\u0000"], ["F\u0000i\u0000x\u0000e\u0000d\u0000 \u0000F\u0000r\u0000e\u0000q\u0000(\u0000H\u0000z\u0000)\u0000", "úVš[‘˜‡s(\u0000H\u0000z\u0000)\u0000", "à¬\u0015È\u001c´ \u0000üÈ\fÓ\u0018Â"], ["T\u0000i\u0000m\u0000e\u0000/\u0000s\u0000t\u0000e\u0000p\u0000(\u0000s\u0000)\u0000", "öeô•/\u0000ek(\u0000s\u0000)\u0000", "\\ÍŒÁÜÂ\u0004¬(\u0000s\u0000)\u0000"], ["C\u0000y\u0000c\u0000l\u0000e\u0000/\u0000s\u0000t\u0000e\u0000p\u0000(\u0000#\u0000)\u0000", "hT\u001fg/\u0000ek(\u0000#\u0000)\u0000", "\\ÍŒÁüÈ0®"], ["C\u0000u\u0000r\u0000v\u0000e\u0000 \u0000v\u0000a\u0000l\u0000 \u0000l\u0000e\u0000v\u0000e\u0000l\u0000 \u0000n\u0000a\u0000m\u0000e\u0000", "òf¿~“^„v\rTðy", "á¬ Á\u001cÁà¬tÇ„¹"], ["U\u0000s\u0000e\u0000 \u0000C\u0000u\u0000r\u0000v\u0000e\u0000 \u0000V\u0000a\u0000l\u0000 \u0000l\u0000e\u0000v\u0000e\u0000l\u0000?\u0000", "òf¿~“^<P", "\u0012¬¬¹©Æ"], ["L\u0000e\u0000v\u0000e\u0000l\u00002\u0000(\u0000V\u0000)\u0000", "4ls^2\u0000(\u0000V\u0000)\u0000", "\u0000É\u0004Ç2\u0000(\u0000V\u0000)\u0000"], ["D\u0000i\u0000f\u0000f\u0000 \u0000F\u0000r\u0000e\u0000q\u0000(\u0000H\u0000z\u0000)\u0000", "î]\u0006R‘˜‡s(\u0000H\u0000z\u0000)\u0000", "(ÌüÈ\fÓ\u0018Â(\u0000H\u0000z\u0000)\u0000"], ["D\u0000i\u0000f\u0000f\u0000/\u0000R\u0000a\u0000t\u0000i\u0000o\u0000", "î]\u0002_/\u0000Ôk‡s", "à¬\u0015È/\u0000D¾`¹"], ["S\u0000t\u0000a\u0000r\u0000t\u0000 \u0000F\u0000r\u0000e\u0000q\u0000(\u0000H\u0000z\u0000)\u0000", "\u0000_ËY‘˜‡s(\u0000H\u0000z\u0000)\u0000", "ÜÂ‘Ç(\u0000H\u0000z\u0000)\u0000"], ["S\u0000t\u0000o\u0000p\u0000 \u0000F\u0000r\u0000e\u0000q\u0000(\u0000H\u0000z\u0000)\u0000", "\\Pbk‘˜‡s(\u0000H\u0000z\u0000)\u0000", "\u0015ÈÀÉ(\u0000H\u0000z\u0000)\u0000"], ["R\u0000a\u0000t\u0000i\u0000o\u0000 \u0000V\u0000a\u0000l\u0000", "Ôk<P", "D¾`¹\u0012¬"], ["C\u0000u\u0000r\u0000v\u0000e\u0000 \u0000v\u0000a\u0000l\u0000 \u0000l\u0000e\u0000v\u0000e\u0000l\u0000 \u0000n\u0000a\u0000m\u0000e\u00002\u0000", "òf¿~“^„v\rTðy2\u0000", "á¬ Á\u001cÁà¬tÇ„¹2\u0000"], ["U\u0000s\u0000e\u0000 \u0000C\u0000u\u0000r\u0000v\u0000e\u0000 \u0000V\u0000a\u0000l\u0000 \u0000l\u0000e\u0000v\u0000e\u0000l\u0000?\u00002\u0000", "òf¿~“^<P2\u0000", "\u0012¬¬¹©Æ2\u0000"], ["S\u0000t\u0000e\u0000p\u0000 \u0000R\u0000e\u0000s\u0000o\u0000l\u0000u\u0000t\u0000i\u0000o\u0000n\u0000", "ekÛ\u0006R¨s", "„½tÕ¥²"], ["R\u0000a\u0000t\u0000i\u0000o\u0000", "Ôk‡s", "D¾`¹"]] string[][] [["S\u0000t\u0000i\u0000m\u0000u\u0000l\u0000u\u0000s\u0000 \u0000T\u0000y\u0000p\u0000e\u0000", "Ào±R{|‹W", "Çù­àÂ8Ö\u0015ÖÜÐ"], ["N\u0000o\u0000i\u0000s\u0000e\u0000 \u0000T\u0000y\u0000p\u0000e\u0000", "jVðX{|‹W", "¡ÇLÇ\u0015ÖÜÐ"], ["M\u0000i\u0000n\u0000 \u0000F\u0000r\u0000e\u0000q\u0000(\u0000H\u0000z\u0000)\u0000", "\u0000g\u000f\\‘˜‡s(\u0000H\u0000z\u0000)\u0000", "\\ÍŒÁüÈ\fÓ\u0018Â"], ["M\u0000a\u0000x\u0000 \u0000F\u0000r\u0000e\u0000q\u0000(\u0000H\u0000z\u0000)\u0000", "\u0000g'Y‘˜‡s(\u0000H\u0000z\u0000)\u0000", "\\Í\u0000³üÈ\fÓ\u0018Â"], ["L\u0000e\u0000v\u0000e\u0000l\u0000(\u0000V\u0000)\u0000", "E^¦^(\u0000V\u0000)\u0000", "\u0000É\u0004Ç(\u0000V\u0000)\u0000"], ["D\u0000u\u0000r\u0000a\u0000t\u0000i\u0000o\u0000n\u0000(\u0000s\u0000)\u0000", "\u0001cí~öeô•(\u0000s\u0000)\u0000", "ÀÉÁÜÂ\u0004¬"], ["C\u0000u\u0000r\u0000v\u0000e\u0000 \u0000v\u0000a\u0000l\u0000 \u0000l\u0000e\u0000v\u0000e\u0000l\u0000 \u0000n\u0000a\u0000m\u0000e\u0000", "òf¿~“^„v\rTðy", "á¬ Á\u001cÁà¬tÇ„¹"], ["U\u0000s\u0000e\u0000 \u0000C\u0000u\u0000r\u0000v\u0000e\u0000 \u0000V\u0000a\u0000l\u0000 \u0000l\u0000e\u0000v\u0000e\u0000l\u0000?\u0000", "òf¿~“^<P", "\u0012¬¬¹©Æ"]] string[][] [["S\u0000t\u0000i\u0000m\u0000u\u0000l\u0000u\u0000s\u0000 \u0000T\u0000y\u0000p\u0000e\u0000", "Ào±R{|‹W", "Çù­àÂ8Ö\u0015ÖÜÐ"], ["L\u0000e\u0000v\u0000e\u0000l\u0000(\u0000V\u0000)\u0000", "E^¦^(\u0000V\u0000)\u0000", "\u0000É\u0004Ç(\u0000V\u0000)\u0000"], ["M\u0000i\u0000n\u0000 \u0000F\u0000r\u0000e\u0000q\u0000(\u0000H\u0000z\u0000)\u0000", "\u0000gNO‘˜‡s(\u0000H\u0000z\u0000)\u0000", "\\ÍŒÁüÈ\fÓ\u0018Â"], ["M\u0000a\u0000x\u0000 \u0000F\u0000r\u0000e\u0000q\u0000(\u0000H\u0000z\u0000)\u0000", "\u0000gØš‘˜‡s(\u0000H\u0000z\u0000)\u0000", "\\Í\u0000³üÈ\fÓ\u0018Â"], ["D\u0000u\u0000r\u0000a\u0000t\u0000i\u0000o\u0000n\u0000(\u0000s\u0000)\u0000", "\u0001cí~öeô•(\u0000s\u0000)\u0000", "ÀÉÁÜÂ\u0004¬"], ["F\u0000r\u0000e\u0000q\u0000 \u0000R\u0000o\u0000u\u0000n\u0000d\u0000i\u0000n\u0000g\u0000", "‘˜‡sÛV\r‚”NeQ", "üÈ\fÓ\u0018Âe´ø­¬¹0®"], ["R\u0000o\u0000u\u0000n\u0000d\u0000i\u0000n\u0000g\u0000 \u0000V\u0000a\u0000l\u0000", "ÛV\r‚”NeQ<P", "e´ø­¬¹0®\u0012¬(\u0000H\u0000z\u0000)\u0000"], ["T\u0000o\u0000n\u0000e\u0000s\u0000", "ó—", "LÇpÈ"], ["C\u0000u\u0000r\u0000v\u0000e\u0000 \u0000v\u0000a\u0000l\u0000 \u0000l\u0000e\u0000v\u0000e\u0000l\u0000 \u0000n\u0000a\u0000m\u0000e\u0000", "òf¿~“^„v\rTðy", "á¬ Á\u001cÁà¬tÇ„¹"], ["U\u0000s\u0000e\u0000 \u0000C\u0000u\u0000r\u0000v\u0000e\u0000 \u0000V\u0000a\u0000l\u0000 \u0000l\u0000e\u0000v\u0000e\u0000l\u0000?\u0000", "òf¿~“^<P", "\u0012¬¬¹©Æ"], ["S\u0000t\u0000e\u0000p\u0000 \u0000R\u0000e\u0000s\u0000o\u0000l\u0000u\u0000t\u0000i\u0000o\u0000n\u0000", "ekÛ\u0006R¨s", "„½tÕ¥²"]]] -> w51
        frame "fstepsw", Default {
        }
        frame "flogsw" {
        }
        frame "ampsw" {
        }
        frame "wavefile" {
        }
        frame "dcconn" {
        }
        frame "twotone" {
        }
        frame "noise" {
        }
        frame "mltitone" {
        }
      }
    }
    frame "Acquisition" {
      # "10"
    }
    frame "Analysis" {
      # "8"
    }
    frame "Post Processing" {
      n9 = call "CRYConvert ASCII to Unicode.vi"("ASCII"=w65) -> ("Unicode"=w64:string)  [unwired: 4 in]
      n10 = case shown="\"Chinese traditional\"" w63 {
        tunnel: [w94 w95 w96 w97] -> w69
        frame "English", Default {
          w94 = 0 items=["System default"=0, "Latin-1"=1252, "Japanese"=932, "Korean"=947, "Chinese simplified"=936, "Chinese traditional"=950, "Central Europe"=1250, "Cyrillic"=1251, "Greek"=1253, "Turkish"=1254, "Hebrew"=1255, "Arabic"=1256, "Baltic"=1257, "Thai"=874, "Vietnamese"=783, "UTF8"=65001, "UTF-7"=65000] ("Code Page")
        }
        frame "Chinese" {
          w95 = 936 items=["System default"=0, "Latin-1"=1252, "Japanese"=932, "Korean"=947, "Chinese simplified"=936, "Chinese traditional"=950, "Central Europe"=1250, "Cyrillic"=1251, "Greek"=1253, "Turkish"=1254, "Hebrew"=1255, "Arabic"=1256, "Baltic"=1257, "Thai"=874, "Vietnamese"=783, "UTF8"=65001, "UTF-7"=65000] ("Code Page")
        }
        frame "Korean" {
          w96 = 949 items=["System default"=0, "Latin-1"=1252, "Japanese"=932, "Korean"=949, "Chinese simplified"=936, "Chinese traditional"=950, "Central Europe"=1250, "Cyrillic"=1251, "Greek"=1253, "Turkish"=1254, "Hebrew"=1255, "Arabic"=1256, "Baltic"=1257, "Thai"=874, "Vietnamese"=783, "UTF8"=65001, "UTF-7"=65000] ("Code Page")
        }
        frame "Chinese traditional" {
          w97 = 950 items=["System default"=0, "Latin-1"=1252, "Japanese"=932, "Korean"=949, "Chinese simplified"=936, "Chinese traditional"=950, "Central Europe"=1250, "Cyrillic"=1251, "Greek"=1253, "Turkish"=1254, "Hebrew"=1255, "Arabic"=1256, "Baltic"=1257, "Thai"=874, "Vietnamese"=783, "UTF8"=65001, "UTF-7"=65000] ("Code Page")
        }
      }
      n11 = case shown="3..5, 7..13" w68 {
        selector: w68 -> [w73 _ w93]
        tunnel: string[][] [["T\u0000h\u0000i\u0000s\u0000 \u0000o\u0000p\u0000e\u0000r\u0000a\u0000t\u0000i\u0000o\u0000n\u0000 \u0000i\u0000s\u0000 \u0000u\u0000n\u0000a\u0000v\u0000a\u0000i\u0000l\u0000a\u0000b\u0000l\u0000e\u0000.\u0000", "Ù*NÐ{/f\rNïSýv.\u0000", "tÇ \u0000ðÅ°À@Ç \u0000ˆ½\u0000¬¥²iÕÈ²ä².\u0000"], ["T\u0000h\u0000i\u0000s\u0000 \u0000o\u0000p\u0000e\u0000r\u0000a\u0000t\u0000i\u0000o\u0000n\u0000 \u0000i\u0000s\u0000 \u0000u\u0000n\u0000a\u0000v\u0000a\u0000i\u0000l\u0000a\u0000b\u0000l\u0000e\u0000 \u0000f\u0000o\u0000r\u0000 \u0000S\u0000i\u0000n\u0000g\u0000l\u0000e\u0000 \u0000V\u0000a\u0000l\u0000u\u0000e\u0000s\u0000.\u0000", "(WUS¯~<PÙ*NÐ{/f\rNïSýv.\u0000", "è²\u001cÂ\u0012¬ÐÅ\u001cÁ \u0000tÇ \u0000ðÅ°À@Ç \u0000ˆ½\u0000¬¥²iÕÈ²ä².\u0000"], ["T\u0000h\u0000e\u0000 \u0000f\u0000o\u0000l\u0000l\u0000o\u0000w\u0000i\u0000n\u0000g\u0000 \u0000e\u0000r\u0000r\u0000o\u0000r\u0000s\u0000 \u0000w\u0000e\u0000r\u0000e\u0000 \u0000f\u0000o\u0000u\u0000n\u0000d\u0000.\u0000", "ÑS°s†N‚Y\u000bN„v\u0019•ï‹.\u0000", "ä²LÇXÇ \u0000$Æ Ç\u0000¬ \u0000\u001c¼¬¬\u0018´\u0000ÆµÂÈ²ä².\u0000"], ["I\u0000n\u0000v\u0000a\u0000l\u0000i\u0000d\u0000 \u0000v\u0000a\u0000r\u0000i\u0000a\u0000b\u0000l\u0000e\u0000", "\rNckS_„vÂSpe", "˜Ç»º\u001c´ \u0000À¼\u0018Â"], ["i\u0000n\u0000 \u0000e\u0000q\u0000u\u0000a\u0000t\u0000i\u0000o\u0000n\u0000.\u0000", "(W¹e\u000bz.\u0000", "\u0000¬ \u0000)¼\u0015ÈÝÂÐÅ \u0000ˆÇµÂÈ²ä².\u0000"], ["A\u0000 \u0000s\u0000e\u0000l\u0000e\u0000c\u0000t\u0000e\u0000d\u0000 \u0000o\u0000p\u0000e\u0000r\u0000a\u0000n\u0000d\u0000 \u0000w\u0000a\u0000s\u0000 \u0000d\u0000e\u0000l\u0000e\u0000t\u0000e\u0000d\u0000 \u0000f\u0000r\u0000o\u0000m\u0000 \u0000t\u0000h\u0000e\u0000 \u0000C\u0000u\u0000r\u0000v\u0000e\u0000 \u0000L\u0000i\u0000b\u0000r\u0000a\u0000r\u0000y\u0000.\u0000", "(Wòf¿~^-N\tébvÐ{pe«mdN.\u0000", " ÁÝÐ\u001c´ \u0000ðÅ°ÀÇ\u0000¬ \u0000á¬ Á\u001cÁà¬ÐÅ\u001cÁ \u0000ÀÉÌÆLÈµÂÈ²ä².\u0000"], ["S\u0000e\u0000l\u0000e\u0000c\u0000t\u0000 \u0000o\u0000p\u0000e\u0000r\u0000a\u0000n\u0000d\u0000 \u0000!\u0000", "÷\tébÐ{pe.\u0000", "ðÅ°ÀÇ|¹ \u0000 ÁÝÐXÕíÂÜÂ$Æ!\u0000"], ["W\u0000a\u0000r\u0000n\u0000i\u0000n\u0000g\u0000:\u0000 \u0000 \u0000O\u0000n\u0000e\u0000 \u0000o\u0000r\u0000 \u0000m\u0000o\u0000r\u0000e\u0000 \u0000d\u0000a\u0000t\u0000a\u0000 \u0000p\u0000o\u0000i\u0000n\u0000t\u0000s\u0000 \u0000h\u0000a\u0000v\u0000e\u0000 \u0000b\u0000e\u0000e\u0000n\u0000 \u0000i\u0000n\u0000t\u0000e\u0000r\u0000p\u0000o\u0000l\u0000a\u0000t\u0000e\u0000d\u0000\n\u0000b\u0000e\u0000c\u0000a\u0000u\u0000s\u0000e\u0000 \u0000a\u0000t\u0000 \u0000l\u0000e\u0000a\u0000s\u0000t\u0000 \u0000o\u0000n\u0000e\u0000 \u0000S\u0000e\u0000a\u0000r\u0000c\u0000h\u0000 \u0000R\u0000a\u0000n\u0000g\u0000e\u0000 \u0000s\u0000p\u0000e\u0000c\u0000i\u0000f\u0000i\u0000e\u0000d\u0000 \u0000c\u0000o\u0000n\u0000t\u0000a\u0000i\u0000n\u0000e\u0000d\u0000 \u0000n\u0000o\u0000\n\u0000a\u0000c\u0000t\u0000u\u0000a\u0000l\u0000 \u0000d\u0000a\u0000t\u0000a\u0000 \u0000p\u0000o\u0000i\u0000n\u0000t\u0000s\u0000 \u0000b\u0000u\u0000t\u0000 \u0000w\u0000a\u0000s\u0000 \u0000w\u0000i\u0000t\u0000h\u0000i\u0000n\u0000 \u0000t\u0000h\u0000e\u0000 \u0000e\u0000n\u0000d\u0000 \u0000p\u0000o\u0000i\u0000n\u0000t\u0000s\u0000 \u0000o\u0000f\u0000 \u0000t\u0000h\u0000e\u0000 \u0000c\u0000u\u0000r\u0000v\u0000e\u0000.\u0000", "fJT:\u0000\u0000N*N\u0016b\u001aY*NpencÒc<P\n\u0000àV:Nó\u0011\\\u0000N*N\u001cd\"}\u0003ôVQ*g\tg\n\u0000(W[Evpenc¹pòf¿~vÓ~_g¹p.\u0000", "½¬à¬:\u0000\u0001È´ÅÄ³ \u0000\\Õ\u001c¬XÇ \u0000ÐÐÉÀl­íÅtÇ \u0000á¬ ÁXÇ \u0000]°\u0010Èä´tÇ \u0000DÅÌ² \u0000äÂ\u001cÈ \u0000ÇÌ¸\u0010Èä´DÇ \u0000ìÓhÕXÕÀ»\\¸ \u0000\\Õ\u001c¬ \u0000\u0010¶² \u0000ø­ \u0000tÇÁÀXÇ \u0000ÇÌ¸\u0010ÈtÇ \u0000ô¼\u0004¬\u0018´\u0000ÆµÂÈ²ä².\u0000"], ["C\u0000a\u0000n\u0000n\u0000o\u0000t\u0000 \u0000r\u0000e\u0000s\u0000o\u0000l\u0000v\u0000e\u0000 \u0000t\u0000h\u0000e\u0000 \u0000e\u0000s\u0000t\u0000i\u0000m\u0000a\u0000t\u0000e\u0000d\u0000 \u0000r\u0000e\u0000s\u0000o\u0000n\u0000a\u0000n\u0000c\u0000e\u0000.\u0000", "\rNý€ã‰³Q0O¡‹qQ/c.\u0000", "ÉÓ\u0000¬\u001c´ \u0000õ¬ÄÉ@Ç \u0000€Ô\u0018Â \u0000ÆÅµÂÈ²ä².\u0000"], ["W\u0000a\u0000r\u0000n\u0000i\u0000n\u0000g\u0000:\u0000 \u0000 \u0000M\u0000o\u0000r\u0000e\u0000 \u0000t\u0000h\u0000a\u0000n\u0000 \u0000o\u0000n\u0000e\u0000 \u0000i\u0000n\u0000t\u0000e\u0000r\u0000s\u0000e\u0000c\u0000t\u0000i\u0000o\u0000n\u0000 \u0000p\u0000o\u0000i\u0000n\u0000t\u0000\n\u0000w\u0000a\u0000s\u0000 \u0000f\u0000o\u0000u\u0000n\u0000d\u0000 \u0000i\u0000n\u0000 \u0000t\u0000h\u0000e\u0000 \u0000s\u0000e\u0000a\u0000r\u0000c\u0000h\u0000 \u0000r\u0000a\u0000n\u0000g\u0000e\u0000.\u0000\n\u0000T\u0000h\u0000e\u0000 \u0000r\u0000e\u0000s\u0000u\u0000l\u0000t\u0000 \u0000i\u0000s\u0000 \u0000t\u0000h\u0000e\u0000 \u0000f\u0000i\u0000r\u0000s\u0000t\u0000 \u0000p\u0000o\u0000i\u0000n\u0000t\u0000 \u0000f\u0000o\u0000u\u0000n\u0000d\u0000.\u0000", "f‹JT:\u0000 \u0000\u0000N*NåN\nN¤NLu\u0004Y«ˆÑS°s(W\u001cd\"}\u0003ƒôV.\u0000\n\u0000Ó~œg/f,{\u0000N*N¹p„vÑS°s.\u0000", "½¬à¬:\u0000 \u0000\\Õ\u001c¬tÇÁÀXÇ \u0000P­(Ì\u0010ÈtÇ \u0000ÐÐÉÀl­íÅÐÅ\u001cÁ \u0000\u001c¼¬¬\u0018´\u0000ÆµÂÈ²ä².\u0000 \u0000°¬ü¬”² \u0000«ÌøÉ\u0010È…ÇÈ²ä².\u0000"], ["Y\u0000o\u0000u\u0000 \u0000m\u0000a\u0000y\u0000 \u0000o\u0000n\u0000l\u0000y\u0000 \u0000s\u0000e\u0000l\u0000e\u0000c\u0000t\u0000 \u0000o\u0000n\u0000e\u0000 \u0000w\u0000a\u0000v\u0000e\u0000f\u0000o\u0000r\u0000m\u0000 \u0000s\u0000e\u0000a\u0000r\u0000c\u0000h\u0000 \u0000r\u0000a\u0000n\u0000g\u0000e\u0000 \u0000a\u0000t\u0000 \u0000a\u0000 \u0000t\u0000i\u0000m\u0000e\u0000.\u0000 \u0000P\u0000r\u0000e\u0000v\u0000i\u0000o\u0000u\u0000s\u0000 \u0000s\u0000e\u0000l\u0000e\u0000c\u0000t\u0000i\u0000o\u0000n\u0000 \u0000w\u0000i\u0000l\u0000l\u0000 \u0000b\u0000e\u0000 \u0000d\u0000i\u0000s\u0000c\u0000a\u0000r\u0000d\u0000e\u0000d\u0000.\u0000", "`OêSý\téb\u0000N*Nâlb_\u001cd\"}v\u0003ôV.\u0000åNMRv\téb\u0006\\«\"N\u0003_.\u0000", "ù²àÂ@Ç \u0000\\Õ\u001c¬XÇ \u0000ÜÂ\u0004¬\fÓ\u0015ÖÐÐÉÀ”¼\u0004ÇÌ¹DÇ \u0000 ÁÝÐ`Õ\u0018Â \u0000ˆÇµÂÈ²ä².\u0000 \u0000tÇ\u0004ÈXÇ \u0000 ÁÝÐ@Ç \u00004»ÜÂ\u0018´\u0000ÆµÂÈ²ä².\u0000"], ["T\u0000h\u0000e\u0000 \u0000f\u0000i\u0000r\u0000s\u0000t\u0000 \u0000n\u0000u\u0000m\u0000b\u0000e\u0000r\u0000 \u0000i\u0000n\u0000 \u0000t\u0000h\u0000e\u0000 \u0000r\u0000a\u0000n\u0000g\u0000e\u0000\n\u0000m\u0000u\u0000s\u0000t\u0000 \u0000b\u0000e\u0000 \u0000l\u0000e\u0000s\u0000s\u0000 \u0000t\u0000h\u0000a\u0000n\u0000 \u0000t\u0000h\u0000e\u0000 \u0000s\u0000e\u0000c\u0000o\u0000n\u0000d\u0000 \u0000n\u0000u\u0000m\u0000b\u0000e\u0000r\u0000.\u0000", ",{\u0000N*NpeW[v\u0003ôV\rN_Ç,{N*NpeW[.\u0000", "«Ì¼øÉ \u0000\u0018ÂÇ² \u0000P´¼øÉ \u0000\u0018ÂÇ|¹ \u0000\bÍü¬`Õ\u0018Â \u0000ÆÅµÂÈ²ä².\u0000"], ["S\u0000e\u0000a\u0000r\u0000c\u0000h\u0000 \u0000R\u0000a\u0000n\u0000g\u0000e\u0000 \u0000l\u0000i\u0000s\u0000t\u0000 \u0000i\u0000t\u0000e\u0000m\u0000 \u0000\"\u0000%\u0000s\u0000\"\u0000\n\u0000i\u0000s\u0000 \u0000a\u0000l\u0000r\u0000e\u0000a\u0000d\u0000y\u0000 \u0000o\u0000n\u0000 \u0000t\u0000h\u0000e\u0000 \u0000l\u0000i\u0000s\u0000t\u0000.\u0000", "\u001cd\"}\u0003ƒôV„v\u0017Rhˆy˜îv \u0000[\u0000%\u0000s\u0000]\u0000 \u0000ò]Ï~\u0017R(W\rTUS\nN.\u0000", "ÐÐÉÀ”¼\u0004Ç©º]¸mÕ©º \u0000[\u0000%\u0000s\u0000]\u0000tÇ \u0000tÇø» \u0000©º]¸ÐÅ \u0000tÈ¬ÇiÕÈ²ä².\u0000"], ["W\u0000r\u0000o\u0000n\u0000g\u0000 \u0000d\u0000a\u0000t\u0000a\u0000 \u0000t\u0000y\u0000p\u0000e\u0000 \u0000n\u0000a\u0000m\u0000e\u0000 \u0000f\u0000o\u0000r\u0000 \u0000t\u0000h\u0000i\u0000s\u0000 \u0000c\u0000o\u0000n\u0000v\u0000e\u0000r\u0000s\u0000i\u0000o\u0000n\u0000 \u0000V\u0000I\u0000.\u0000", "dkHr,gV\u0000I\u0000„vpenc{|‹W\u0019•ï‹.\u0000", "ÇÌ¸\u0015ÖÝÂtÇ \u0000ÀÒ½¹È²ä².\u0000"], ["O\u0000n\u0000l\u0000y\u0000 \u0000u\u0000n\u0000i\u0000t\u0000s\u0000 \u0000f\u0000o\u0000r\u0000 \u0000U\u0000s\u0000e\u0000r\u0000 \u0000D\u0000e\u0000f\u0000i\u0000n\u0000e\u0000d\u0000 \u0000C\u0000o\u0000n\u0000s\u0000t\u0000a\u0000n\u0000t\u0000s\u0000 \u0000c\u0000a\u0000n\u0000 \u0000b\u0000e\u0000 \u0000e\u0000d\u0000i\u0000t\u0000e\u0000d\u0000.\u0000", "êS\tgUSMO(u7b[INv8^peïSåN\u0016.\u0000", "¬À©ÆÇ\u0000¬ \u0000\u0015ÈXÇ\\Õ \u0000ÁÀ\u0018ÂÐÅ\u001cÁÌ¹ \u0000è²\u0004Ç|¹ \u0000¸ÓÑÉ`Õ\u0018Â \u0000ÇµÂÈ²ä².\u0000"], ["C\u0000a\u0000n\u0000 \u0000n\u0000o\u0000t\u0000 \u0000r\u0000e\u0000v\u0000e\u0000r\u0000t\u0000.\u0000", "àeÕlØS.\u0000", "ÐÆø¼ÇÌ¸|¹ \u0000}Ç´Å \u0000ä´|Ç\u0018Â \u0000ÆÅµÂÈ²ä².\u0000"], ["O\u0000p\u0000e\u0000r\u0000a\u0000n\u0000d\u0000 \u0000A\u0000 \u0000i\u0000s\u0000 \u0000n\u0000o\u0000t\u0000 \u0000a\u0000 \u0000V\u0000a\u0000l\u0000u\u0000e\u0000.\u0000", "Íd\\OpeA\u0000\rN/f<P.\u0000", "ðÅ°ÀÇ \u0000A\u0000\u0000¬ \u0000\u0012¬tÇ \u0000DÅÙ²È²ä².\u0000"], ["O\u0000p\u0000e\u0000r\u0000a\u0000n\u0000d\u0000 \u0000B\u0000 \u0000i\u0000s\u0000 \u0000n\u0000o\u0000t\u0000 \u0000a\u0000 \u0000V\u0000a\u0000l\u0000u\u0000e\u0000.\u0000", "Íd\\OpeB\u0000\rN/f<P.\u0000", "ðÅ°ÀÇ \u0000B\u0000\u0000¬ \u0000\u0012¬tÇ \u0000DÅÙ²È²ä².\u0000"], ["O\u0000p\u0000e\u0000r\u0000a\u0000n\u0000d\u0000 \u0000A\u0000&\u0000B\u0000 \u0000a\u0000r\u0000e\u0000 \u0000n\u0000o\u0000t\u0000 \u0000t\u0000h\u0000e\u0000 \u0000V\u0000a\u0000l\u0000u\u0000e\u0000s\u0000.\u0000", "Íd\\OpeA\u0000TB\u0000ý\rN/f<P.\u0000", "ðÅ°ÀÇ \u0000A\u0000@ÆB\u0000\u0000¬ \u0000\u0012¬tÇ \u0000DÅÙ²È²ä².\u0000c\u0000"]] -> [w75 w87 w91]
        tunnel: w66 -> [w74 w83 w89]
        tunnel: [w72 w78 w88] -> w71
        tunnel: w64 -> [_ w80 _]
        frame 0, 1, 6, Default {
          n12 = Index Array(array=w75, index (row)=w73, index (col)=w74) -> (element=w72:string)
        }
        frame 2 {
          w76 = ""
          w77 = "\n\u0000"
          n13 = Index Array(array=w87, index (row) #1=2 ("index (row)"), index (col) #1=w83, index (row) #2=3 ("index (row)"), index (col) #2=w83, index (row) #3=4 ("disabled index (row)"), index (col) #3=w83) -> (element #1=w82:string, element #2=w81:string, element #3=w79:string)
          n14 = Concatenate Strings(w82, w77, w77, w81, w76, w80, w76, w79) -> (w78:string)
        }
        frame 3..5, 7..13 {
          n15 = Add(x=w93, y=2) -> (x+y=w90:i32)
          n16 = Index Array(array=w91, index (row)=w90, index (col)=w89) -> (element=w88:string)
        }
      }
      n17 = call "CRYConvert Unicode to Multibyte.vi"("Code Page"=w69, "Unicode String"=w71) -> ("Multibyte string"=w67:string)  [unwired: 8 in, 1 out]
    }
    frame "Post Processing Sub" {
    }
    frame "Limits" {
      # "7"
    }
    frame "Limits Sub" {
    }
    frame "Display" {
    }
    frame "Serial No" {
    }
    frame "Statistics" {
      n18 = case shown="\"Chinese traditional\"" w107 {
        tunnel: [w128 w129 w130 w131] -> w109
        frame "English", Default {
          w128 = 0 items=["System default"=0, "Latin-1"=1252, "Japanese"=932, "Korean"=947, "Chinese simplified"=936, "Chinese traditional"=950, "Central Europe"=1250, "Cyrillic"=1251, "Greek"=1253, "Turkish"=1254, "Hebrew"=1255, "Arabic"=1256, "Baltic"=1257, "Thai"=874, "Vietnamese"=783, "UTF8"=65001, "UTF-7"=65000] ("Code Page")
        }
        frame "Chinese" {
          w129 = 936 items=["System default"=0, "Latin-1"=1252, "Japanese"=932, "Korean"=947, "Chinese simplified"=936, "Chinese traditional"=950, "Central Europe"=1250, "Cyrillic"=1251, "Greek"=1253, "Turkish"=1254, "Hebrew"=1255, "Arabic"=1256, "Baltic"=1257, "Thai"=874, "Vietnamese"=783, "UTF8"=65001, "UTF-7"=65000] ("Code Page")
        }
        frame "Korean" {
          w130 = 949 items=["System default"=0, "Latin-1"=1252, "Japanese"=932, "Korean"=949, "Chinese simplified"=936, "Chinese traditional"=950, "Central Europe"=1250, "Cyrillic"=1251, "Greek"=1253, "Turkish"=1254, "Hebrew"=1255, "Arabic"=1256, "Baltic"=1257, "Thai"=874, "Vietnamese"=783, "UTF8"=65001, "UTF-7"=65000] ("Code Page")
        }
        frame "Chinese traditional" {
          w131 = 950 items=["System default"=0, "Latin-1"=1252, "Japanese"=932, "Korean"=949, "Chinese simplified"=936, "Chinese traditional"=950, "Central Europe"=1250, "Cyrillic"=1251, "Greek"=1253, "Turkish"=1254, "Hebrew"=1255, "Arabic"=1256, "Baltic"=1257, "Thai"=874, "Vietnamese"=783, "UTF8"=65001, "UTF-7"=65000] ("Code Page")
        }
      }
      n19 = case shown="6" w105 {
        selector: w105 -> [w112 _ _]
        tunnel: string[][] [["P\u0000l\u0000e\u0000a\u0000s\u0000e\u0000 \u0000s\u0000e\u0000l\u0000e\u0000c\u0000t\u0000 \u0000a\u0000 \u0000c\u0000u\u0000r\u0000v\u0000e\u0000 \u0000t\u0000o\u0000 \u0000p\u0000r\u0000o\u0000c\u0000e\u0000e\u0000d\u0000.\u0000", "÷\téb\u0000N*Nòf¿~ÛL.\u0000", "üÈ\fÓ\u0018Â9¸íÅá¬ ÁDÇ \u0000 \u0000 ÁÝÐXÕíÂÜÂ$Æ.\u0000"], ["P\u0000l\u0000e\u0000a\u0000s\u0000e\u0000 \u0000s\u0000e\u0000l\u0000e\u0000c\u0000t\u0000 \u0000a\u0000 \u0000r\u0000e\u0000s\u0000u\u0000l\u0000t\u0000 \u0000t\u0000o\u0000 \u0000p\u0000r\u0000o\u0000c\u0000e\u0000e\u0000d\u0000.\u0000", "÷\téb\u0000N*NÓ~gÛL.\u0000", "°¬ü¬\u0012¬DÇ \u0000 ÁÝÐXÕíÂÜÂ$Æ.\u0000"], ["P\u0000l\u0000e\u0000a\u0000s\u0000e\u0000 \u0000s\u0000e\u0000l\u0000e\u0000c\u0000t\u0000 \u0000a\u0000 \u0000s\u0000t\u0000a\u0000t\u0000i\u0000s\u0000t\u0000i\u0000c\u0000s\u0000 \u0000m\u0000e\u0000a\u0000s\u0000u\u0000r\u0000e\u0000m\u0000e\u0000n\u0000t\u0000.\u0000", "÷\téb\u0000N*Nß~¡KmÏ.\u0000", "µÑÄ¬!Î\u0015ÈDÇ \u0000 \u0000 ÁÝÐXÕíÂÜÂ$Æ.\u0000"], ["P\u0000p\u0000&\u0000P\u0000p\u0000k\u0000 \u0000c\u0000a\u0000n\u0000 \u0000o\u0000n\u0000l\u0000y\u0000 \u0000b\u0000e\u0000 \u0000p\u0000e\u0000r\u0000f\u0000o\u0000r\u0000m\u0000e\u0000d\u0000 \u0000o\u0000n\u0000 \u0000s\u0000i\u0000n\u0000g\u0000l\u0000e\u0000 \u0000v\u0000a\u0000l\u0000u\u0000e\u0000s\u0000.\u0000 \u0000", "P\u0000p\u0000&\u0000P\u0000p\u0000k\u0000êSý€/f1uUS\u0000N„v<P.\u0000", "P\u0000p\u0000&\u0000P\u0000p\u0000k\u0000”² \u0000ä²Ì¹ \u0000è²\u001cÂ\u0012¬<Ç\\¸€½0Ñ \u0000Ä¬°À)´È²ä².\u0000"], ["T\u0000h\u0000e\u0000 \u0000U\u0000S\u0000L\u0000 \u0000m\u0000u\u0000s\u0000t\u0000 \u0000b\u0000e\u0000 \u0000g\u0000r\u0000e\u0000a\u0000t\u0000e\u0000r\u0000 \u0000t\u0000h\u0000a\u0000n\u0000 \u0000t\u0000h\u0000e\u0000 \u0000L\u0000S\u0000L\u0000.\u0000", "U\u0000S\u0000L\u0000Å_{˜'YŽNL\u0000S\u0000L\u0000.\u0000", "U\u0000S\u0000L\u0000”² \u0000L\u0000S\u0000L\u0000ô¼ä² \u0000\u0018¼Ü´ÜÂ \u0000äÎ|Å \u0000iÕÈ²ä².\u0000"]] -> [w113 w118 w125]
        tunnel: [w110 w114 w121] -> w103
        tunnel: w104 -> [w111 w117 w124]
        frame 0..4, Default {
          n20 = Index Array(array=w113, index (row)=w112, index (col)=w111) -> (element=w110:string)
        }
        frame 5 {
          n21 = Index Array(array=w118, index (row) #1=0 ("index"), index (col) #1=w117, index (row) #2=2 ("index"), index (col) #2=w117) -> (element #1=w116:string, element #2=w115:string)
          n22 = Concatenate Strings(w116, w115) -> (w114:string)
        }
        frame 6 {
          n23 = Index Array(array=w125, index (row) #1=1 ("index"), index (col) #1=w124, index (row) #2=2 ("index"), index (col) #2=w124) -> (element #1=w123:string, element #2=w122:string)
          n24 = Concatenate Strings(w123, w122) -> (w121:string)
        }
      }
      n25 = call "CRYConvert Unicode to Multibyte.vi"("Code Page"=w109, "Unicode String"=w103) -> ("Multibyte string"=w108:string)  [unwired: 8 in, 1 out]
    }
    frame "Auto Save" {
      # "21"
      n26 = case shown="19..32" w136 {
        selector: w136 -> [_ _ _ _ _ _ _ _ _ _ _ _ _ _ _ _ _ _ _ w327]
        tunnel: string[][] [["W\u0000a\u0000r\u0000n\u0000i\u0000n\u0000g\u0000s\u0000:\u0000", "f‹JT:\u0000", "½¬à¬:\u0000"], ["P\u0000l\u0000e\u0000a\u0000s\u0000e\u0000 \u0000i\u0000n\u0000d\u0000i\u0000c\u0000a\u0000t\u0000e\u0000 \u0000a\u0000 \u0000f\u0000i\u0000l\u0000e\u0000 \u0000n\u0000a\u0000m\u0000e\u0000.\u0000", "÷‹\u0007cúQ‡eöN\rTW[.\u0000", "\fÓ|ÇtÇ„¹DÇ \u0000 ÁÝÐXÕíÂÜÂ$Æ.\u0000"], ["P\u0000l\u0000e\u0000a\u0000s\u0000e\u0000 \u0000s\u0000e\u0000l\u0000e\u0000c\u0000t\u0000 \u0000a\u0000 \u0000c\u0000u\u0000r\u0000v\u0000e\u0000 \u0000o\u0000r\u0000 \u0000r\u0000e\u0000s\u0000u\u0000l\u0000t\u0000 \u0000t\u0000o\u0000 \u0000s\u0000a\u0000v\u0000e\u0000.\u0000", "\u0005n\tébÝOX[vòf¿~\u0016b\u0005Ó~g\rTW[.\u0000", "ô¼\u0000­XÕ$¸”² \u0000üÈ\fÓ\u0018Â9¸íÅá¬ ÁtÇ˜° \u0000°¬ü¬\u0012¬DÇ \u0000 ÁÝÐXÕíÂÜÂ$Æ.\u0000"], ["P\u0000l\u0000e\u0000a\u0000s\u0000e\u0000 \u0000s\u0000e\u0000l\u0000e\u0000c\u0000t\u0000 \u0000a\u0000 \u0000d\u0000e\u0000s\u0000t\u0000i\u0000n\u0000a\u0000t\u0000i\u0000o\u0000n\u0000 \u0000f\u0000o\u0000r\u0000 \u0000y\u0000o\u0000u\u0000r\u0000 \u0000d\u0000a\u0000t\u0000a\u0000.\u0000", "÷\tébpencvÈ~¹p.\u0000", "ÇÌ¸XÇ \u0000©º\u0001ÈÀÉ|¹ \u0000 ÁÝÐXÕíÂÜÂ$Æ.\u0000"], ["P\u0000l\u0000e\u0000a\u0000s\u0000e\u0000 \u0000s\u0000e\u0000l\u0000e\u0000c\u0000t\u0000 \u0000a\u0000 \u0000d\u0000e\u0000s\u0000t\u0000i\u0000n\u0000a\u0000t\u0000i\u0000o\u0000n\u0000 \u0000f\u0000o\u0000r\u0000 \u0000y\u0000o\u0000u\u0000r\u0000 \u0000r\u0000e\u0000s\u0000u\u0000l\u0000t\u0000s\u0000.\u0000", "÷\tébÓ~gvÈ~¹p.\u0000", "°¬ü¬XÇ \u0000©º\u0001ÈÀÉ|¹ \u0000 ÁÝÐXÕíÂÜÂ$Æ.\u0000"], ["P\u0000l\u0000e\u0000a\u0000s\u0000e\u0000 \u0000s\u0000e\u0000l\u0000e\u0000c\u0000t\u0000 \u0000a\u0000 \u0000d\u0000e\u0000s\u0000t\u0000i\u0000n\u0000a\u0000t\u0000i\u0000o\u0000n\u0000 \u0000f\u0000o\u0000r\u0000 \u0000y\u0000o\u0000u\u0000r\u0000 \u0000d\u0000a\u0000t\u0000a\u0000 \u0000o\u0000r\u0000 \u0000r\u0000e\u0000s\u0000u\u0000l\u0000t\u0000s\u0000.\u0000", "÷\tébpenc\u0016b\u0005Ó~gvÈ~¹p.\u0000", "ÇÌ¸° \u0000°¬ü¬XÇ \u0000©º\u0001ÈÀÉ|¹ \u0000 ÁÝÐXÕíÂÜÂ$Æ.\u0000"], ["P\u0000l\u0000e\u0000a\u0000s\u0000e\u0000 \u0000s\u0000e\u0000l\u0000e\u0000c\u0000t\u0000 \u0000a\u0000 \u0000d\u0000e\u0000s\u0000t\u0000i\u0000n\u0000a\u0000t\u0000i\u0000o\u0000n\u0000 \u0000f\u0000o\u0000r\u0000 \u0000y\u0000o\u0000u\u0000r\u0000 \u0000w\u0000a\u0000v\u0000e\u0000f\u0000o\u0000r\u0000m\u0000s\u0000.\u0000", "÷\tébâlb_vÈ~¹p.\u0000", "ÜÂ\u0004¬\fÓ\u0015ÖXÇ \u0000©º\u0001ÈÀÉ|¹ \u0000 ÁÝÐXÕíÂÜÂ$Æ.\u0000"], ["E\u0000r\u0000r\u0000o\u0000r\u0000:\u0000 \u0000c\u0000l\u0000u\u0000s\u0000t\u0000e\u0000r\u0000 \u0000n\u0000o\u0000t\u0000 \u0000o\u0000f\u0000 \u0000t\u0000y\u0000p\u0000e\u0000 \u0000W\u0000a\u0000v\u0000e\u0000f\u0000o\u0000r\u0000m\u0000.\u0000", "\u0019•ï‹:\u0000\rN/fâlb_„v\u0007|.\u0000", "$Æ Ç:\u0000ÜÂ\u0004¬\fÓ\u0015ÖtÐ|·¤Â0Ñ\u0000¬ \u0000DÅÙ²È²ä².\u0000"], ["A\u0000u\u0000t\u0000o\u0000s\u0000a\u0000v\u0000e\u0000 \u0000D\u0000a\u0000t\u0000a\u0000 \u0000F\u0000o\u0000l\u0000d\u0000e\u0000r\u0000 \u0000d\u0000o\u0000e\u0000s\u0000 \u0000n\u0000o\u0000t\u0000 \u0000e\u0000x\u0000i\u0000s\u0000t\u0000.\u0000\n\u0000N\u0000o\u0000 \u0000d\u0000a\u0000t\u0000a\u0000 \u0000w\u0000e\u0000r\u0000e\u0000 \u0000s\u0000a\u0000v\u0000e\u0000d\u0000.\u0000", "ê¨RÝOX[penceöN9Y\rNX[(W.\u0000 \u0000¡l\tgÝOX[vpenc.\u0000", "ÇÙ³ô¼\u0000­ÇÌ¸ñ´]¸½\u0000¬ \u0000tÈ¬ÇXÕÀÉ \u0000JÅµÂÈ²ä².\u0000\n\u0000ô¼\u0000­\u001c´ \u0000ÇÌ¸\u0000¬ \u0000ÆÅµÂÈ²ä².\u0000 \u0000"], ["A\u0000u\u0000t\u0000o\u0000s\u0000a\u0000v\u0000e\u0000 \u0000R\u0000e\u0000s\u0000u\u0000l\u0000t\u0000s\u0000 \u0000F\u0000o\u0000l\u0000d\u0000e\u0000r\u0000 \u0000d\u0000o\u0000e\u0000s\u0000 \u0000n\u0000o\u0000t\u0000 \u0000e\u0000x\u0000i\u0000s\u0000t\u0000.\u0000\n\u0000N\u0000o\u0000 \u0000r\u0000e\u0000s\u0000u\u0000l\u0000t\u0000s\u0000 \u0000w\u0000e\u0000r\u0000e\u0000 \u0000s\u0000a\u0000v\u0000e\u0000d\u0000.\u0000", "ê¨RÝOX[Ó~geöN9Y\rNX[(W.\u0000 \u0000¡l\tgÝOX[vÓ~g.\u0000", "ÇÙ³ô¼\u0000­°¬ü¬ñ´]¸½\u0000¬ \u0000tÈ¬ÇXÕÀÉ \u0000JÅµÂÈ²ä².\u0000\n\u0000ô¼\u0000­\u001c´ \u0000°¬ü¬\u0000¬ \u0000ÆÅµÂÈ²ä².\u0000 \u0000"], ["A\u0000u\u0000t\u0000o\u0000s\u0000a\u0000v\u0000e\u0000 \u0000W\u0000a\u0000v\u0000e\u0000f\u0000o\u0000r\u0000m\u0000s\u0000 \u0000F\u0000o\u0000l\u0000d\u0000e\u0000r\u0000 \u0000d\u0000o\u0000e\u0000s\u0000 \u0000n\u0000o\u0000t\u0000 \u0000e\u0000x\u0000i\u0000s\u0000t\u0000.\u0000\n\u0000N\u0000o\u0000 \u0000w\u0000a\u0000v\u0000e\u0000f\u0000o\u0000r\u0000m\u0000s\u0000 \u0000w\u0000e\u0000r\u0000e\u0000 \u0000s\u0000a\u0000v\u0000e\u0000d\u0000.\u0000", "ê¨RÝOX[âlb_eöN9Y\rNX[(W.\u0000 \u0000¡l\tgÝOX[vâlb_.\u0000", "ÇÙ³ô¼\u0000­\fÓ\u0015Öñ´]¸½\u0000¬ \u0000tÈ¬ÇXÕÀÉ \u0000JÅµÂÈ²ä².\u0000\n\u0000ô¼\u0000­\u001c´ \u0000\fÓ\u0015ÖtÇ \u0000ÆÅµÂÈ²ä².\u0000 \u0000"], ["P\u0000l\u0000e\u0000a\u0000s\u0000e\u0000 \u0000e\u0000n\u0000t\u0000e\u0000r\u0000 \u0000a\u0000 \u0000n\u0000a\u0000m\u0000e\u0000.\u0000", "÷eQ\rTW[.\u0000", "tÇ„¹DÇ \u0000…Ç%¸XÕíÂÜÂ$Æ.\u0000"], ["A\u0000 \u0000n\u0000a\u0000m\u0000e\u0000 \u0000c\u0000a\u0000n\u0000n\u0000o\u0000t\u0000 \u0000c\u0000o\u0000n\u0000t\u0000a\u0000i\u0000n\u0000 \u0000a\u0000n\u0000y\u0000 \u0000o\u0000f\u0000 \u0000t\u0000h\u0000e\u0000 \u0000f\u0000o\u0000l\u0000l\u0000o\u0000w\u0000i\u0000n\u0000g\u0000 \u0000c\u0000h\u0000a\u0000r\u0000a\u0000c\u0000t\u0000e\u0000r\u0000s\u0000:\u0000\\\u0000 \u0000/\u0000 \u0000:\u0000 \u0000*\u0000 \u0000?\u0000 \u0000\"\u0000 \u0000<\u0000 \u0000>\u0000 \u0000|\u0000 \u0000", "\rTW[\rNý€\u0005S+T‚Y\u000bN„vW[&{:\u0000\\\u0000 \u0000/\u0000 \u0000:\u0000 \u0000*\u0000 \u0000?\u0000 \u0000\"\u0000 \u0000<\u0000 \u0000>\u0000 \u0000|\u0000 \u0000", "tÇ„¹@Ç \u0000DÅ˜·XÇ \u0000€½8Öä´DÇ \u0000ìÓhÕ`Õ\u0018Â \u0000ÆÅµÂÈ²ä²:\u0000\\\u0000 \u0000/\u0000 \u0000:\u0000 \u0000*\u0000 \u0000?\u0000 \u0000\"\u0000 \u0000<\u0000 \u0000>\u0000 \u0000|\u0000 \u0000"], ["C\u0000u\u0000r\u0000v\u0000e\u0000 \u0000n\u0000a\u0000m\u0000e\u0000 \u0000n\u0000o\u0000t\u0000 \u0000f\u0000o\u0000u\u0000n\u0000d\u0000.\u0000\n\u0000N\u0000o\u0000 \u0000d\u0000a\u0000t\u0000a\u0000 \u0000w\u0000a\u0000s\u0000 \u0000s\u0000a\u0000v\u0000e\u0000d\u0000.\u0000", "¡lÑS°spenc\rTW[.\u0000 \u0000¡l\tgÝOX[„vpenc.\u0000", "ÇÌ¸tÇ¹DÇ \u0000\u001c¼¬¬XÕÀÉ \u0000»ºÕµÂÈ²ä².\u0000\n\u0000ô¼\u0000­\u001c´ \u0000ÇÌ¸\u0000¬ \u0000ÆÅµÂÈ²ä².\u0000 \u0000"], ["R\u0000e\u0000s\u0000u\u0000l\u0000t\u0000 \u0000n\u0000a\u0000m\u0000e\u0000 \u0000n\u0000o\u0000t\u0000 \u0000f\u0000o\u0000u\u0000n\u0000d\u0000.\u0000\n\u0000N\u0000o\u0000 \u0000r\u0000e\u0000s\u0000u\u0000l\u0000t\u0000s\u0000 \u0000w\u0000e\u0000r\u0000e\u0000 \u0000s\u0000a\u0000v\u0000e\u0000d\u0000.\u0000", "¡lÑS°sÓ~œg\rTW[.\u0000 \u0000¡l\tgÝOX[„vÓ~œg.\u0000", "°¬ü¬\u0012¬tÇ„¹DÇ \u0000\u001c¼¬¬XÕÀÉ \u0000»ºˆÕµÂÈ²ä².\u0000 \u0000 \u0000ô¼\u0000­\u001c´ \u0000°¬ü¬\u0000¬ \u0000ÆÅµÂÈ²ä².\u0000"], ["W\u0000a\u0000v\u0000e\u0000f\u0000o\u0000r\u0000m\u0000 \u0000n\u0000a\u0000m\u0000e\u0000 \u0000n\u0000o\u0000t\u0000 \u0000f\u0000o\u0000u\u0000n\u0000d\u0000.\u0000N\u0000o\u0000 \u0000w\u0000a\u0000v\u0000e\u0000f\u0000o\u0000r\u0000m\u0000 \u0000w\u0000a\u0000s\u0000 \u0000s\u0000a\u0000v\u0000e\u0000d\u0000.\u0000 \u0000", "¡lÑS°sâlb_\rTW[.\u0000 \u0000¡l\tgÝOX[„vâlb_.\u0000", "ÜÂ\u0004¬\fÓ\u0015ÖtÇ„¹DÇ \u0000\u001c¼¬¬XÕÀÉ \u0000»ºˆÕµÂÈ²ä².\u0000ô¼\u0000­\u001c´ \u0000\fÓ\u0015ÖtÇ \u0000ÆÅµÂÈ²ä².\u0000 \u0000"], ["Y\u0000o\u0000u\u0000 \u0000c\u0000a\u0000n\u0000n\u0000o\u0000t\u0000 \u0000u\u0000s\u0000e\u0000 \u0000t\u0000h\u0000e\u0000 \u0000E\u0000x\u0000c\u0000e\u0000l\u0000 \u0000s\u0000a\u0000v\u0000e\u0000 \u0000o\u0000p\u0000t\u0000i\u0000o\u0000n\u0000 \u0000w\u0000i\u0000t\u0000h\u0000 \u0000w\u0000a\u0000v\u0000e\u0000f\u0000o\u0000r\u0000m\u0000s\u0000.\u0000", "âlb_ÝOX[\rNý€(uhˆ<h‡eöN.\u0000", "ÜÂ\u0004¬\fÓ\u0015Öô¼\u0000­@Ç \u0000\\Ô\fÓ|ÇDÇ \u0000¬¹©Æ`Õ\u0018Â \u0000ÆÅµÂÈ²ä².\u0000"], ["Y\u0000o\u0000u\u0000 \u0000c\u0000a\u0000n\u0000n\u0000o\u0000t\u0000 \u0000u\u0000s\u0000e\u0000 \u0000t\u0000h\u0000e\u0000 \u0000W\u0000A\u0000V\u0000 \u0000s\u0000a\u0000v\u0000e\u0000 \u0000o\u0000p\u0000t\u0000i\u0000o\u0000n\u0000 \u0000w\u0000i\u0000t\u0000h\u0000 \u0000r\u0000e\u0000s\u0000u\u0000l\u0000t\u0000s\u0000.\u0000", "Ó~œgÝOX[\rNý€(uâlb_‡eöN.\u0000", "°¬ü¬ô¼\u0000­@Ç \u0000ÜÂ\u0004¬\fÓ\u0015Ö\fÓ|ÇDÇ \u0000¬¹©Æ`Õ\u0018Â \u0000ÆÅµÂÈ²ä².\u0000"], ["Y\u0000o\u0000u\u0000 \u0000m\u0000u\u0000s\u0000t\u0000 \u0000f\u0000i\u0000r\u0000s\u0000t\u0000 \u0000s\u0000e\u0000l\u0000e\u0000c\u0000t\u0000 \u0000a\u0000n\u0000 \u0000i\u0000t\u0000e\u0000m\u0000.\u0000", "`Oå\téb,{\u0000N*Nyîv.\u0000", "«ÌøÉ \u0000mÕ©ºDÇ \u0000 ÁÝÐXÕíÂÜÂ$Æ.\u0000"], ["W\u0000r\u0000o\u0000n\u0000g\u0000 \u0000d\u0000a\u0000t\u0000a\u0000 \u0000t\u0000y\u0000p\u0000e\u0000 \u0000n\u0000a\u0000m\u0000e\u0000 \u0000f\u0000o\u0000r\u0000 \u0000t\u0000h\u0000i\u0000s\u0000 \u0000c\u0000o\u0000n\u0000v\u0000e\u0000r\u0000s\u0000i\u0000o\u0000n\u0000 \u0000V\u0000I\u0000.\u0000", "dkHr,gV\u0000I\u0000„vpenc{|‹W\u0019•ï‹.\u0000", "ÇÌ¸\u0015ÖÝÂtÇ \u0000ÀÒ½¹È²ä².\u0000"], ["C\u0000a\u0000n\u0000 \u0000n\u0000o\u0000t\u0000 \u0000r\u0000e\u0000v\u0000e\u0000r\u0000t\u0000.\u0000", "àeÕlØS.\u0000", "ÐÆø¼ÇÌ¸|¹ \u0000}Ç´Å \u0000ä´|Ç\u0018Â \u0000ÆÅµÂÈ²ä².\u0000"], ["U\u0000D\u0000L\u0000 \u0000o\u0000r\u0000 \u0000D\u0000S\u0000N\u0000 \u0000a\u0000d\u0000d\u0000r\u0000e\u0000s\u0000s\u0000 \u0000i\u0000s\u0000 \u0000w\u0000r\u0000o\u0000n\u0000g\u0000.\u0000 \u0000P\u0000l\u0000e\u0000a\u0000s\u0000e\u0000 \u0000c\u0000h\u0000o\u0000o\u0000s\u0000e\u0000 \u0000c\u0000o\u0000r\u0000r\u0000e\u0000c\u0000t\u0000 \u0000o\u0000n\u0000e\u0000.\u0000", "U\u0000D\u0000L\u0000\u0016bD\u0000S\u0000N\u00000W@W\u0019ï\fÿ÷Í°e\téb.\u0000", "U\u0000D\u0000L\u0000 \u00009Ö@Ç \u0000D\u0000S\u0000N\u0000 \u0000üÈŒÁ\u0000¬ \u0000˜Ç»º\u0018´\u0000ÆµÂÈ²ä².\u0000 \u0000\u0015ÈUÖ\\Õ \u0000üÈŒÁ|¹ \u0000 ÁÝÐXÕíÂÜÂ$Æ.\u0000"], ["Y\u0000o\u0000u\u0000 \u0000c\u0000a\u0000n\u0000n\u0000o\u0000t\u0000 \u0000u\u0000s\u0000e\u0000 \u0000t\u0000h\u0000e\u0000 \u0000D\u0000a\u0000t\u0000a\u0000b\u0000a\u0000s\u0000e\u0000 \u0000s\u0000a\u0000v\u0000e\u0000 \u0000o\u0000p\u0000t\u0000i\u0000o\u0000n\u0000 \u0000w\u0000i\u0000t\u0000h\u0000 \u0000w\u0000a\u0000v\u0000e\u0000f\u0000o\u0000r\u0000m\u0000s\u0000.\u0000", "àeÕlO(upenc“^ÝOX[âlb_‡eöN.\u0000", "ÜÂ\u0004¬\fÓ\u0015Öô¼\u0000­@Ç \u0000ÇÌ¸0®ÀÉ|¹ \u0000¬¹©Æ`Õ\u0018Â \u0000ÆÅµÂÈ²ä².\u0000"]] -> [w146 w152 w163 w172 w182 w192 w200 w208 w220 w230 w240 w249 w260 w270 w280 w288 w300 w310 w320 w330]
        tunnel: [w141 w151 w161 w171 w181 w191 w199 w207 w219 w229 w239 w248 w259 w269 w279 w287 w299 w309 w319 w329] -> w138
        tunnel: w135 -> [w140 w148 w160 w170 w180 w190 w198 w206 w218 w228 w238 w246 w258 w268 w278 w286 w298 w308 w318 w328]
        frame 0, Default {
          n27 = Index Array(array=w146, index (row) #1=0 ("index"), index (col) #1=w140, index (row) #2=2 ("index"), index (col) #2=w140) -> (element #1=w143:string, element #2=w142:string)
          n28 = Concatenate Strings(w143, "\n\u0000", w142) -> (w141:string)
        }
        frame 1 {
          w147 = "\n\u0000"
          n29 = Index Array(array=w152, index (row) #1=0 ("index"), index (col) #1=w148, index (row) #2=1 ("index"), index (col) #2=w148, index (row) #3=2 ("index"), index (col) #3=w148, index (row) #4=3 ("index"), index (col) #4=w148) -> (element #1=w156:string, element #2=w155:string, element #3=w153:string, element #4=w149:string)
          n30 = Concatenate Strings(w156, w147, w155, w147, w153, w147, w149) -> (w151:string)
        }
        frame 2 {
          w159 = "\n\u0000"
          n31 = Index Array(array=w163, index (row) #1=0 ("index"), index (col) #1=w160, index (row) #2=2 ("index"), index (col) #2=w160, index (row) #3=3 ("index"), index (col) #3=w160) -> (element #1=w162:string, element #2=w166:string, element #3=w164:string)
          n32 = Concatenate Strings(w162, w159, w166, w159, w164) -> (w161:string)
        }
        frame 3 {
          w169 = "\n\u0000"
          n33 = Index Array(array=w172, index (row) #1=0 ("index"), index (col) #1=w170, index (row) #2=1 ("index"), index (col) #2=w170, index (row) #3=2 ("index"), index (col) #3=w170) -> (element #1=w173:string, element #2=w176:string, element #3=w174:string)
          n34 = Concatenate Strings(w173, w169, w176, w169, w174) -> (w171:string)
        }
        frame 4 {
          w179 = "\n\u0000"
          n35 = Index Array(array=w182, index (row) #1=0 ("index"), index (col) #1=w180, index (row) #2=1 ("index"), index (col) #2=w180, index (row) #3=3 ("index"), index (col) #3=w180) -> (element #1=w183:string, element #2=w186:string, element #3=w184:string)
          n36 = Concatenate Strings(w183, w179, w186, w179, w184) -> (w181:string)
        }
        frame 5 {
          n37 = Index Array(array=w192, index (row) #1=0 ("index"), index (col) #1=w190, index (row) #2=3 ("index"), index (col) #2=w190) -> (element #1=w194:string, element #2=w193:string)
          n38 = Concatenate Strings(w194, "\n\u0000", w193) -> (w191:string)
        }
        frame 6 {
          n39 = Index Array(array=w200, index (row) #1=0 ("index"), index (col) #1=w198, index (row) #2=1 ("index"), index (col) #2=w198) -> (element #1=w202:string, element #2=w201:string)
          n40 = Concatenate Strings(w202, "\n\u0000", w201) -> (w199:string)
        }
        frame 7 {
          w205 = "\n\u0000"
          n41 = Index Array(array=w208, index (row) #1=0 ("index"), index (col) #1=w206, index (row) #2=1 ("index"), index (col) #2=w206, index (row) #3=2 ("index"), index (col) #3=w206, index (row) #4=4 ("index"), index (col) #4=w206) -> (element #1=w214:string, element #2=w213:string, element #3=w211:string, element #4=w209:string)
          n42 = Concatenate Strings(w214, w205, w213, w205, w211, w205, w209) -> (w207:string)
        }
        frame 8 {
          w217 = "\n\u0000"
          n43 = Index Array(array=w220, index (row) #1=0 ("index"), index (col) #1=w218, index (row) #2=2 ("index"), index (col) #2=w218, index (row) #3=4 ("index"), index (col) #3=w218) -> (element #1=w221:string, element #2=w224:string, element #3=w222:string)
          n44 = Concatenate Strings(w221, w217, w224, w217, w222) -> (w219:string)
        }
        frame 9 {
          w227 = "\n\u0000"
          n45 = Index Array(array=w230, index (row) #1=0 ("index"), index (col) #1=w228, index (row) #2=1 ("index"), index (col) #2=w228, index (row) #3=4 ("index"), index (col) #3=w228) -> (element #1=w231:string, element #2=w234:string, element #3=w232:string)
          n46 = Concatenate Strings(w231, w227, w234, w227, w232) -> (w229:string)
        }
        frame 10 {
          n47 = Index Array(array=w240, index (row) #1=0 ("index"), index (col) #1=w238, index (row) #2=4 ("index"), index (col) #2=w238) -> (element #1=w242:string, element #2=w241:string)
          n48 = Concatenate Strings(w242, "\n\u0000", w241) -> (w239:string)
        }
        frame 11 {
          w245 = "\n\u0000"
          n49 = Index Array(array=w249, index (row) #1=0 ("index"), index (col) #1=w246, index (row) #2=1 ("index"), index (col) #2=w246, index (row) #3=2 ("index"), index (col) #3=w246, index (row) #4=5 ("index"), index (col) #4=w246) -> (element #1=w255:string, element #2=w254:string, element #3=w252:string, element #4=w250:string)
          n50 = Concatenate Strings(w255, w245, w254, w245, w252, w245, w250) -> (w248:string)
        }
        frame 12 {
          w257 = "\n\u0000"
          n51 = Index Array(array=w260, index (row) #1=0 ("index"), index (col) #1=w258, index (row) #2=2 ("index"), index (col) #2=w258, index (row) #3=5 ("index"), index (col) #3=w258) -> (element #1=w264:string, element #2=w263:string, element #3=w261:string)
          n52 = Concatenate Strings(w264, w257, w263, w257, w261) -> (w259:string)
        }
        frame 13 {
          w267 = "\n\u0000"
          n53 = Index Array(array=w270, index (row) #1=0 ("index"), index (col) #1=w268, index (row) #2=1 ("index"), index (col) #2=w268, index (row) #3=5 ("index"), index (col) #3=w268) -> (element #1=w274:string, element #2=w273:string, element #3=w271:string)
          n54 = Concatenate Strings(w274, w267, w273, w267, w271) -> (w269:string)
        }
        frame 14 {
          n55 = Index Array(array=w280, index (row) #1=0 ("index"), index (col) #1=w278, index (row) #2=5 ("index"), index (col) #2=w278) -> (element #1=w282:string, element #2=w281:string)
          n56 = Concatenate Strings(w282, "\n\u0000", w281) -> (w279:string)
        }
        frame 15 {
          w285 = "\n\u0000"
          n57 = Index Array(array=w288, index (row) #1=0 ("index"), index (col) #1=w286, index (row) #2=1 ("index"), index (col) #2=w286, index (row) #3=2 ("index"), index (col) #3=w286, index (row) #4=6 ("index"), index (col) #4=w286) -> (element #1=w294:string, element #2=w293:string, element #3=w291:string, element #4=w289:string)
          n58 = Concatenate Strings(w294, w285, w293, w285, w291, w285, w289) -> (w287:string)
        }
        frame 16 {
          w297 = "\n\u0000"
          n59 = Index Array(array=w300, index (row) #1=0 ("index"), index (col) #1=w298, index (row) #2=2 ("index"), index (col) #2=w298, index (row) #3=6 ("index"), index (col) #3=w298) -> (element #1=w304:string, element #2=w303:string, element #3=w301:string)
          n60 = Concatenate Strings(w304, w297, w303, w297, w301) -> (w299:string)
        }
        frame 17 {
          w307 = "\n\u0000"
          n61 = Index Array(array=w310, index (row) #1=0 ("index"), index (col) #1=w308, index (row) #2=1 ("index"), index (col) #2=w308, index (row) #3=6 ("index"), index (col) #3=w308) -> (element #1=w314:string, element #2=w313:string, element #3=w311:string)
          n62 = Concatenate Strings(w314, w307, w313, w307, w311) -> (w309:string)
        }
        frame 18 {
          n63 = Index Array(array=w320, index (row) #1=0 ("index"), index (col) #1=w318, index (row) #2=6 ("index"), index (col) #2=w318) -> (element #1=w322:string, element #2=w321:string)
          n64 = Concatenate Strings(w322, "\n\u0000", w321) -> (w319:string)
        }
        frame 19..32 {
          n65 = Subtract(x=w327, y=12) -> (x-y=w325:i32)
          n66 = Index Array(array=w330, index (row)=w325, index (col)=w328) -> (element=w329:string)
        }
      }
      n67 = case shown="\"Chinese traditional\"" w132 {
        tunnel: [w331 w332 w333 w334] -> w137
        frame "English", Default {
          w331 = 0 items=["System default"=0, "Latin-1"=1252, "Japanese"=932, "Korean"=947, "Chinese simplified"=936, "Chinese traditional"=950, "Central Europe"=1250, "Cyrillic"=1251, "Greek"=1253, "Turkish"=1254, "Hebrew"=1255, "Arabic"=1256, "Baltic"=1257, "Thai"=874, "Vietnamese"=783, "UTF8"=65001, "UTF-7"=65000] ("Code Page")
        }
        frame "Chinese" {
          w332 = 936 items=["System default"=0, "Latin-1"=1252, "Japanese"=932, "Korean"=947, "Chinese simplified"=936, "Chinese traditional"=950, "Central Europe"=1250, "Cyrillic"=1251, "Greek"=1253, "Turkish"=1254, "Hebrew"=1255, "Arabic"=1256, "Baltic"=1257, "Thai"=874, "Vietnamese"=783, "UTF8"=65001, "UTF-7"=65000] ("Code Page")
        }
        frame "Korean" {
          w333 = 949 items=["System default"=0, "Latin-1"=1252, "Japanese"=932, "Korean"=949, "Chinese simplified"=936, "Chinese traditional"=950, "Central Europe"=1250, "Cyrillic"=1251, "Greek"=1253, "Turkish"=1254, "Hebrew"=1255, "Arabic"=1256, "Baltic"=1257, "Thai"=874, "Vietnamese"=783, "UTF8"=65001, "UTF-7"=65000] ("Code Page")
        }
        frame "Chinese traditional" {
          w334 = 950 items=["System default"=0, "Latin-1"=1252, "Japanese"=932, "Korean"=949, "Chinese simplified"=936, "Chinese traditional"=950, "Central Europe"=1250, "Cyrillic"=1251, "Greek"=1253, "Turkish"=1254, "Hebrew"=1255, "Arabic"=1256, "Baltic"=1257, "Thai"=874, "Vietnamese"=783, "UTF8"=65001, "UTF-7"=65000] ("Code Page")
        }
      }
      n68 = call "CRYConvert Unicode to Multibyte.vi"("Code Page"=w137, "Unicode String"=w138) -> ("Multibyte string"=w134:string)  [unwired: 8 in, 1 out]
    }
    frame "Auto Save Sub" {
    }
    frame "Recall" {
    }
    frame "Recall Sub" {
    }
    frame "Signal Generator" {
    }
    frame "Multimeter" {
    }
    frame "Multimeter Sub" {
      n69 = Equal To 0?(x=w345) -> (x = 0?=w348:bool)
      n70 = Equal?(x=w345, y=1) -> (x = y?=w341:bool)
      n71 = Select(t=string[][] [["C\u0000o\u0000n\u0000t\u0000i\u0000n\u0000u\u0000e\u0000", "ç~ \u0000í~", "Ä¬ \u0000Á"], ["S\u0000t\u0000o\u0000p\u0000", "\\P \u0000bk", "\u0015È \u0000ÀÉ"], ["C\u0000o\u0000n\u0000t\u0000i\u0000n\u0000u\u0000e\u0000", "ç~ \u0000í~", "Ä¬ \u0000Á"], ["S\u0000t\u0000o\u0000p\u0000", "\\P \u0000bk", "\u0015È \u0000ÀÉ"]], s=w341, f=string[][] [["R\u0000e\u0000s\u0000t\u0000a\u0000r\u0000t\u0000", "Í‘°e\u0000_ËY", "Ä¬ \u0000Á"], ["S\u0000t\u0000o\u0000p\u0000", "\\P \u0000bk", "\u0015È \u0000ÀÉ"], ["R\u0000e\u0000s\u0000t\u0000a\u0000r\u0000t\u0000", "Í‘°e\u0000_ËY", "Ä¬ \u0000Á"], ["S\u0000t\u0000o\u0000p\u0000", "\\P \u0000bk", "\u0015È \u0000ÀÉ"]]) -> (s? t:f=w340:string[][])
      n72 = Select(t=string[][] [["S\u0000t\u0000a\u0000r\u0000t\u0000", "\u0000_ \u0000ËY", "ÜÂ \u0000‘Ç"], ["S\u0000t\u0000o\u0000p\u0000", "\\P \u0000bk", "\u0015È \u0000ÀÉ"], ["S\u0000t\u0000a\u0000r\u0000t\u0000", "\u0000_ \u0000ËY", "ÜÂ \u0000‘Ç"], ["S\u0000t\u0000o\u0000p\u0000", "\\P \u0000bk", "\u0015È \u0000ÀÉ"]], s=w348, f=w340) -> (s? t:f=w346:string[][])
    }
    frame "Oscilloscope-FFT" {
    }
    frame "Oscilloscope-FFT Sub" {
      n73 = Equal To 0?(x=w351) -> (x = 0?=w354:bool)
      n74 = Select(t=string[][] [["S\u0000t\u0000a\u0000r\u0000t\u0000", "\u0000_ \u0000ËY", "ÜÂ \u0000‘Ç"], ["M\u0000e\u0000a\u0000s\u0000u\u0000r\u0000i\u0000n\u0000g\u0000.\u0000.\u0000.\u0000", "\\P \u0000bk", "\u0015È \u0000ÀÉ"], ["S\u0000t\u0000a\u0000r\u0000t\u0000", "\u0000_ \u0000ËY", "ÜÂ \u0000‘Ç"], ["M\u0000e\u0000a\u0000s\u0000u\u0000r\u0000i\u0000n\u0000g\u0000.\u0000.\u0000.\u0000", "\\P \u0000bk", "\u0015È \u0000ÀÉ"]], s=w354, f=string[][] [["C\u0000o\u0000n\u0000t\u0000i\u0000n\u0000u\u0000e\u0000s\u0000", "ç~ \u0000í~", "(¸ \u0000Á"], ["S\u0000t\u0000o\u0000p\u0000", "\\P \u0000bk", "\u0015È \u0000ÀÉ"], ["C\u0000o\u0000n\u0000t\u0000i\u0000n\u0000u\u0000e\u0000s\u0000", "ç~ \u0000í~", "(¸ \u0000Á"], ["S\u0000t\u0000o\u0000p\u0000", "\\P \u0000bk", "\u0015È \u0000ÀÉ"]]) -> (s? t:f=w352:string[][])
    }
    frame "RTA" {
    }
    frame "Operator Configure" {
    }
    frame "Start" {
    }
    frame "End" {
    }
    frame "Data" {
    }
    frame "Result" {
    }
    frame "CRY6181 One" {
    }
    frame Default {
    }
  }
  "Message Sub 3" <- w10
  n75 = global read "CRYMainGlobal.vi" "Launch Mode"() -> (w6:enum32{"CRY6181", "CRY6181 One"})
  n76 = Equal?(x=w6, y=enum32{"CRY6181", "CRY6181 One"}."CRY6181") -> (x = y?=w5:bool)
  n77 = Select(t=w2, s=w5, f=string[] ["C\u0000R\u0000Y\u00006\u00001\u00008\u00001\u0000 \u0000E\u0000l\u0000e\u0000c\u0000t\u0000r\u0000o\u0000-\u0000A\u0000c\u0000o\u0000u\u0000s\u0000t\u0000i\u0000c\u0000 \u0000A\u0000n\u0000a\u0000l\u0000y\u0000s\u0000i\u0000s\u0000 \u0000S\u0000y\u0000s\u0000t\u0000e\u0000m\u0000 \u0000O\u0000n\u0000e\u0000", "C\u0000R\u0000Y\u00006\u00001\u00008\u00001\u0000 \u00005uðX\u0006Rgû|ß~", "LÇ¥ÕtÕ\u001dÁ\u0004Õ\\¸ø­Œ· \u0000XÕ˜°"]) -> ()  [unwired: 1 out]
  n78 = for {
    tunnel: [w366] -> w1 mode=indexing
    tunnel: w2 -> [w363] mode=indexing
    n79 = global read "CRYMainGlobal.vi" "Verion Number Unicode"() -> (w365:string)
    n80 = Concatenate Strings(w363, " \u0000" ("message"), w365) -> (w366:string)
  }
  n81 = Index Array(array=w15, index (col)=w8) -> (element=→"Unicode Message Sub":string[])  [unwired: 1 in]
  n82 = Index Array(array=w21, index (row)="Error No", index (col)=w8) -> (element=w20:string)
  "Unicode Message" <- w20
  n83 = Index Array(array=w1, index=w8) -> (element=w13:string)
  n84 = case shown="\"Chinese traditional\"" w7 {
    tunnel: [w367 w368 w369 w370] -> w12
    frame "English", Default {
      w367 = 0 items=["System default"=0, "Latin-1"=1252, "Japanese"=932, "Korean"=947, "Chinese simplified"=936, "Chinese traditional"=950, "Central Europe"=1250, "Cyrillic"=1251, "Greek"=1253, "Turkish"=1254, "Hebrew"=1255, "Arabic"=1256, "Baltic"=1257, "Thai"=874, "Vietnamese"=783, "UTF8"=65001, "UTF-7"=65000] ("Code Page")
    }
    frame "Chinese" {
      w368 = 936 items=["System default"=0, "Latin-1"=1252, "Japanese"=932, "Korean"=947, "Chinese simplified"=936, "Chinese traditional"=950, "Central Europe"=1250, "Cyrillic"=1251, "Greek"=1253, "Turkish"=1254, "Hebrew"=1255, "Arabic"=1256, "Baltic"=1257, "Thai"=874, "Vietnamese"=783, "UTF8"=65001, "UTF-7"=65000] ("Code Page")
    }
    frame "Korean" {
      w369 = 949 items=["System default"=0, "Latin-1"=1252, "Japanese"=932, "Korean"=949, "Chinese simplified"=936, "Chinese traditional"=950, "Central Europe"=1250, "Cyrillic"=1251, "Greek"=1253, "Turkish"=1254, "Hebrew"=1255, "Arabic"=1256, "Baltic"=1257, "Thai"=874, "Vietnamese"=783, "UTF8"=65001, "UTF-7"=65000] ("Code Page")
    }
    frame "Chinese traditional" {
      w370 = 950 items=["System default"=0, "Latin-1"=1252, "Japanese"=932, "Korean"=949, "Chinese simplified"=936, "Chinese traditional"=950, "Central Europe"=1250, "Cyrillic"=1251, "Greek"=1253, "Turkish"=1254, "Hebrew"=1255, "Arabic"=1256, "Baltic"=1257, "Thai"=874, "Vietnamese"=783, "UTF8"=65001, "UTF-7"=65000] ("Code Page")
    }
  }
  n85 = for {
    tunnel: w18 -> [w373] mode=indexing
    tunnel: w12 -> [w372]
    tunnel: [w371] -> w17 mode=indexing
    n86 = call "CRYConvert Unicode to Multibyte.vi"("Code Page"=w372, "Unicode String"=w373) -> ("Multibyte string"=w371:string)  [unwired: 8 in, 1 out]
  }
  "Message Sub" <- w17
  n87 = call "CRYConvert Unicode to Multibyte.vi"("Code Page"=w12, "Unicode String"=w20) -> ("Multibyte string"=→"Message":string)  [unwired: 8 in, 1 out]
  n88 = call "CRYConvert Unicode to Multibyte.vi"("Code Page"=w12, "Unicode String"=w13) -> ("Multibyte string"=→"Window Title":string)  [unwired: 8 in, 1 out]
